vi "tui_DataLog Log Table.vi"() -> ()   [LabVIEW 2012]
doc: "Interactively retrieves and tabulates the content of multiple tag logs. The retrieved data can be filtered, graphed, and exported. This GUI is designed for quick and dirty analysis. When performing complex or recurring retrieval operations, it is advisable to use a query script instead.\n\nThis GUI has two phases. During the first phase you must specify what data is to be retrieved from the logging database. During the second phase you can perform actions on the retrieved data.\n\nSpecifying what data to retrieve involves assigning a set of tags to the table columns and specifying a time interval and optional interpolation time step. After retrieval and tabulation, it is possible to exclude or include rows of data so as to filter the dataset to a subset of interest. A suitable series of include and exclude actions can yield the equivalent of a boolean selection expression. For example, excluding all rows where tag \"foo\" is not equal to 2 and then including all rows where tag \"bar\" is larger than zero is equivalent to retaining all rows that satisfy the boolean expression \"foo==2 or bar>0\".\n\nThe optionally filtered data can be graphed or exported. Only when the dataset is cleared does it again become possible to specify a new set of tags, that is, the GUI will revert back from the second to the first phase.\n\nThe server-side memory usage is kept in check through configurable limits and by performing the retrieval on a per-tag basis. Still, some moderation is advisable since the client-side memory usage is not bounded. When retrieving lots of data for multiple tags, the table will likely take a long time to display and the client might even run out of memory."
uses:
  served/DataLog Database Infos_srv.ctl
  served/re_DataLog Query_srv.ctl
  served/DataLog Databases_srv.ctl
  typedefs/t_DataLog Log Table States.ctl
  library/typedefs/t_Library Session Methods.ctl
  typedefs/t_Datalog Table Columns Methods.ctl
  typedefs/t_DataLog Query Served Methods.ctl
  typedefs/t_DataLog Value Types.ctl
  library/glb_Library Configuration Globals.vi
panel:
  out "export path":path
  in  "string":string
  in  "match":T1(ring)
  in  "number":dbl
  in  "comparison":T2(ring)
  out "excluded":i32
  out "included":i32
  in  "xy graph":bool
  in  "time graph":bool
  in  "include":bool
  in  "exclude":bool
  in  "enable/disable":bool
  in  "time step":dbl=60.0 min=0.01 max=1000000000000.0 step=1.0 format="%<%H:%M:%S%2u>t"
  in  "mode":bool
  in  "reorder":bool
  in  "remove all":bool
  in  "insert":bool
  in  "subset":bool
  in  "add":bool
  in  "multi":bool
  in  "remove":bool
  in  "sort":bool
  in  "export":bool
  in  "clear":bool
  out "query":T3
  in  "database":i32(ring) items=["testdb"]
  out "log table":string[][](table)
  out "database infos":T4
  in  "earliest":bool
  in  "begin time":timestamp format="%<%H:%M:%S%2u\n%Y/%m/%d>T"
  in  "latest":bool
  in  "end time":timestamp format="%<%H:%M:%S%2u\n%Y/%m/%d>T"
  in  "retrieve":bool
  in  "exit":bool
  out "databases":T5
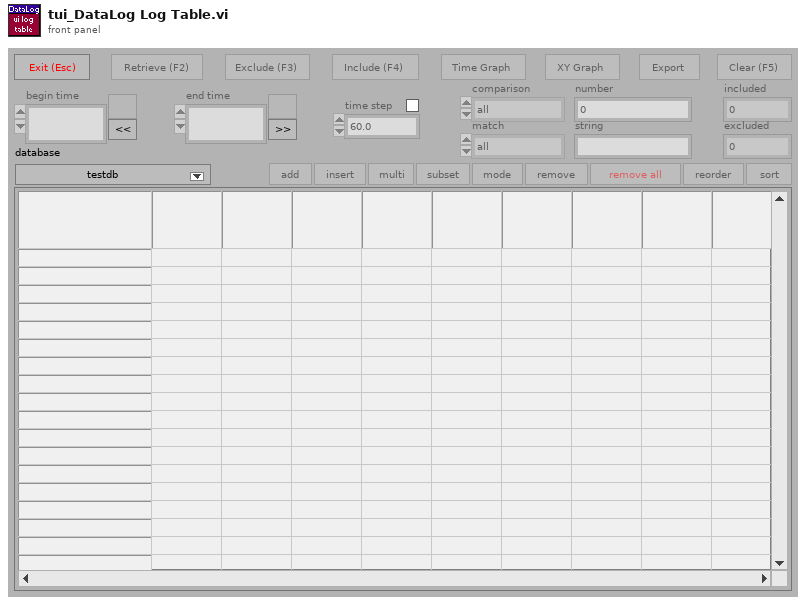
[diagram p1: front panel]
types:
  T1 = enum16{"all", "==", "~=", "contains", "contains c.i.", "lacks", "lacks c.i.", "starts with", "starts with c.i.", "UNDEFINED", "DEFINED"}
  T2 = enum16{"all", "==", "~=", ">", ">=", "<=", "<", "==NaN", "~=NaN"}
  T3 = typedef "re_DataLog Query_srv.ctl" = refnum<vi>
  T4 = typedef "DataLog Database Infos_srv.ctl" = refnum<vi>
  T5 = typedef "DataLog Databases_srv.ctl" = refnum<vi>
  T6 = typedef "t_DataLog Log Table States.ctl" = enum16{"empty queue", "retrieve", "ret clear", "ret presize", "ret range", "ret merge", "ret at", "ret step", "ret times", "ret interpolate", "ret tabulate", "ret free", "num. exclude", "num. include", "str. exclude", "str. include", "time graph", "graph xy", "xy query", "xy check", "xy open", "xy set", "xy correlate", "xy run", "export", "show string", "count rows", "time headers", "tabulate", "abort query", "clear query", "clear all", "set database", "deselect", "ablement", "resize", "initialize", "init refs", "init databases", "init persist", "cleanup", "stop"}
  T7 = typedef "t_Library Session Methods.ctl" = enum16{"run", "get arg", "set arg", "delist", "cleanup?", "start session", "stop session", "list empty?"}
  T8 = typedef "t_Datalog Table Columns Methods.ctl" = enum16{"clear", "#columns", "#number", "add", "insert", "remove", "change mode", "reorder", "sort", "index", "get by name", "interpolatable?", "ats?", "update"}
  T9 = typedef "t_DataLog Query Served Methods.ctl" = enum16{"set range", "step times", "get times", "interpolate", "interpolate str", "read range", "read str range", "merge&read range", "merge&read str range", "merge range", "clear"}
  T10 = cluster{"graph VI":refnum<vi>, "x tag":string, "y tag":string}
  T11 = cluster{"times":dbl[], "values":dbl[], "strings":string[]}
  T12 = typedef "t_DataLog Value Types.ctl" = enum16{"number", "string"}
  T13 = typedef "t_DataLog Tag Config.ctl" = cluster{"name":string, "unit":string, "temporal":T14, "value":T12, "index":i32, "capacity":i32, "is meta?":bool, "mincapacity":i32, "deadband":dbl, "limit delay":dbl, "format":T15, "precision":u8, "undefine":bool, "update":bool, "update period":u16, "expression":string, "description":string, "logging algorithm":T16, "logging parameters":dbl[]}
  T14 = typedef "t_DataLog Temporal Types.ctl" = enum16{"set&hold", "sample", "event"}
  T15 = typedef "t_DataLog Numerical Format.ctl" = enum8{"fractional", "exponential", "engineering"}
  T16 = typedef "t_DataLog Logging Algorithms.ctl" = enum16{"nothing", "changes", "everything", "every Nth", "time threshold", "value threshold + prior", "t or v threshold", "t or v threshold + prior"}
  T17 = enum32{"existing file", "new file", "new or existing file", "existing dir", "new dir", "new or existing dir", "existing file (use LLBs)", "new file (use LLBs)", "new or existing file (use LLBs)", "new or existing file or directory (use LLBs)"}
  T18 = typedef "LVRowAndColumnTypeDef.ctl" = cluster{"Row":i32, "Column":i32}
  T19 = typedef "eventvkey.ctl" = enum16{"ASCII", "Enter", "Return", "Shift", "Ctrl", "Alt", "Cmd", "Opt", "Caps", "NumLock", "Clear", "Break", "Up", "Down", "Left", "Right", "Insert", "Delete", "Home", "End", "PageUp", "PageDown", "Escape", "Help", "Pause", "ScrollLock", "F1", "F2", "F3", "F4", "F5", "F6", "F7", "F8", "F9", "F10", "F11", "F12", "F13", "F14", "F15", "F16", "F17", "F18", "F19", "F20", "F21", "F22", "F23", "F24", "Play", "VolumeUp", "VolumeDown", "Mute", "Two Byte Char"}
  T20 = cluster{"times":dbl[], "values":dbl[], "strings":string[]}[]
  T21 = typedef "t_DataLog Table Retrieval Modes.ctl" = enum16{"at", "interpolate", "at+interpolate"}
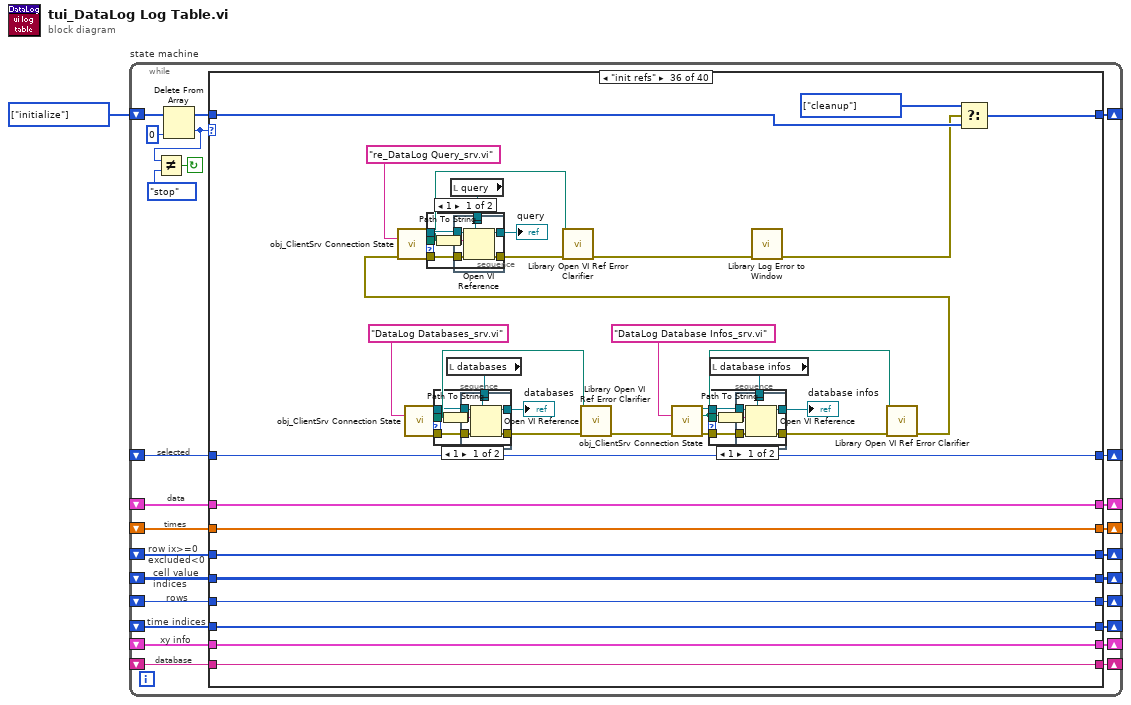
[diagram p0: block diagram]
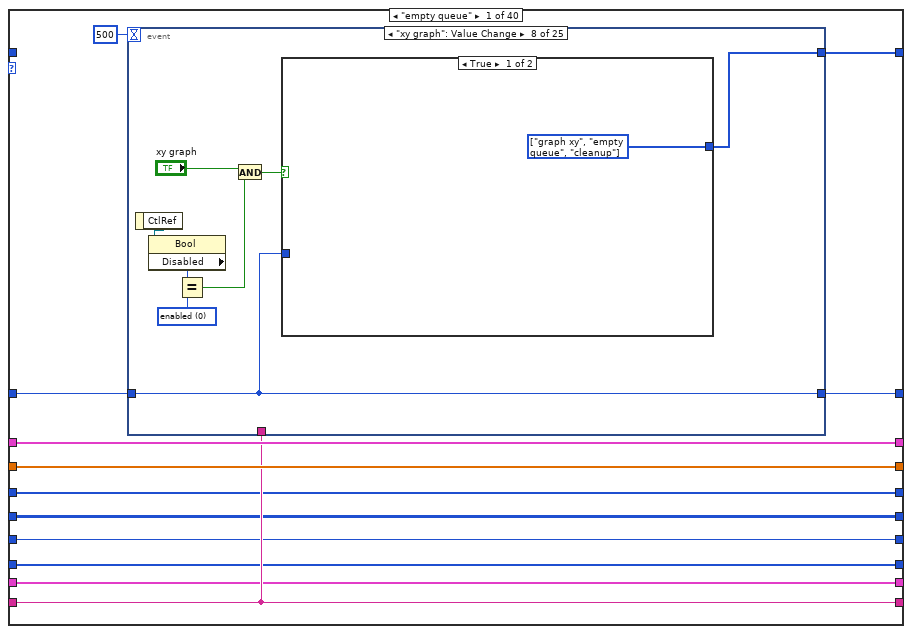
[diagram p2: hidden frame]
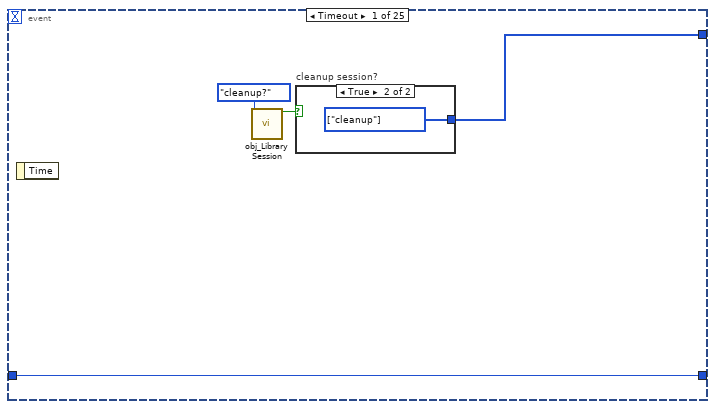
[diagram p3: hidden frame]
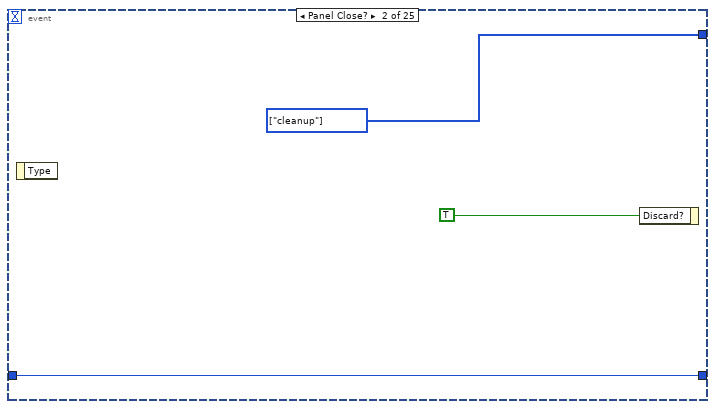
[diagram p5: hidden frame]
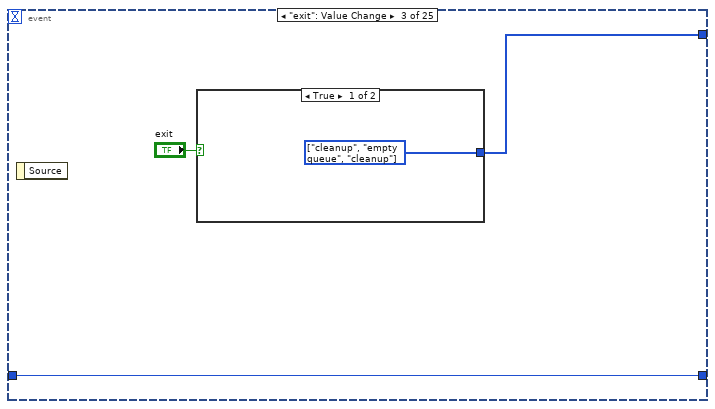
[diagram p6: hidden frame]
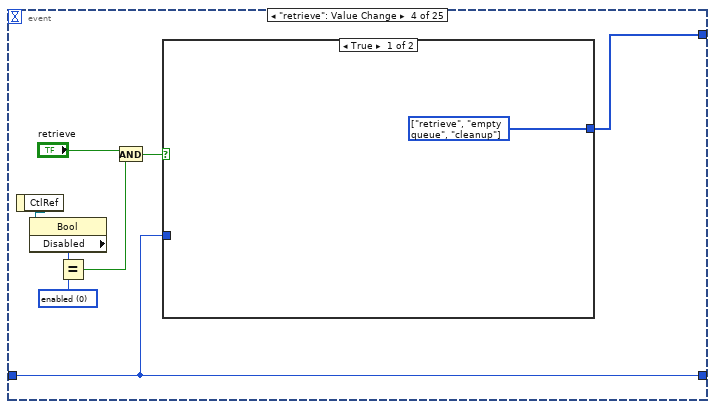
[diagram p8: hidden frame]
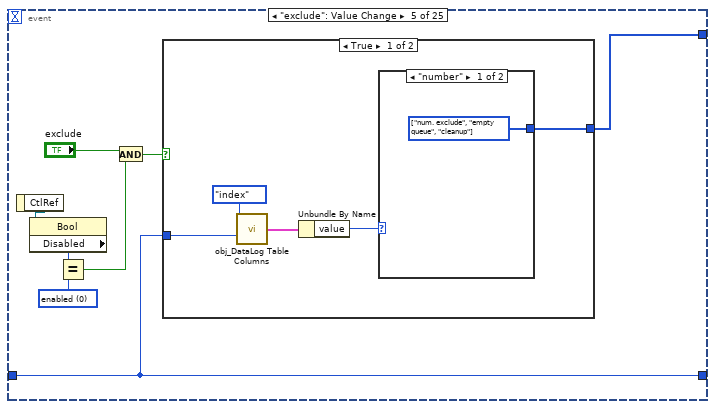
[diagram p10: hidden frame]
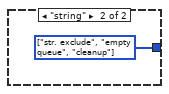
[diagram p11: hidden frame]
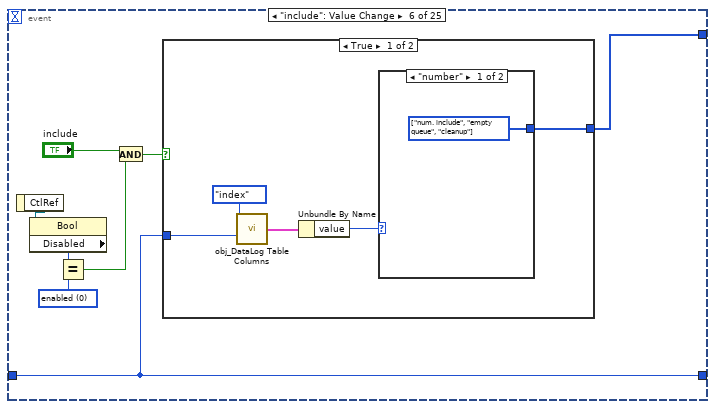
[diagram p13: hidden frame]
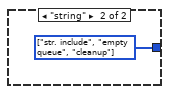
[diagram p14: hidden frame]
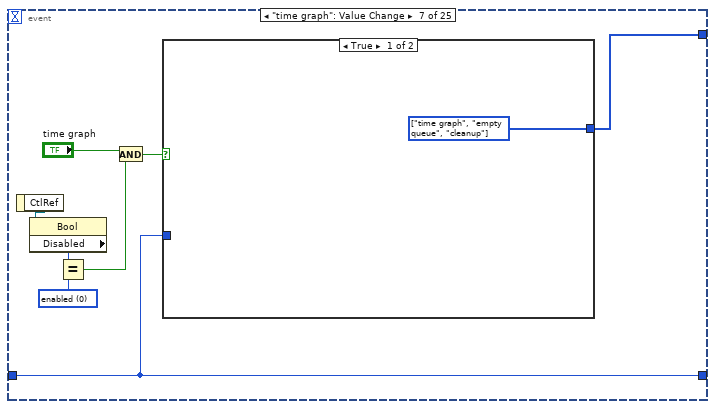
[diagram p16: hidden frame]
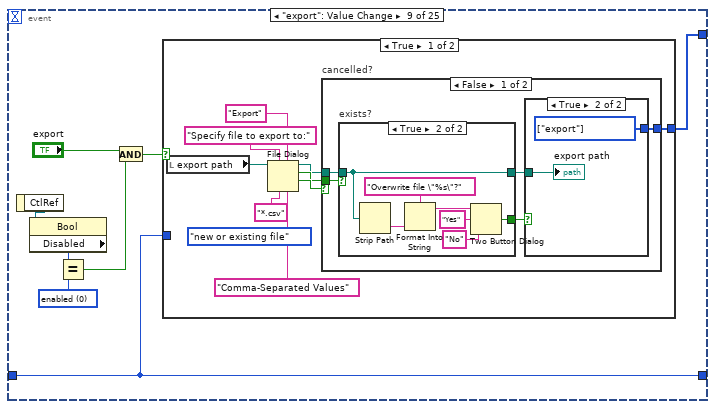
[diagram p19: hidden frame]
diagram:
  w1 = T6[] [enum."initialize"] items=["empty queue", "retrieve", "ret clear", "ret presize", "ret range", "ret merge", "ret at", "ret step", "ret times", "ret interpolate", "ret tabulate", "ret free", "num. exclude", "num. include", "str. exclude", "str. include", "time graph", "graph xy", "xy query", "xy check", "xy open", "xy set", "xy correlate", "xy run", "export", "show string", "count rows", "time headers", "tabulate", "abort query", "clear query", "clear all", "set database", "deselect", "ablement", "resize", "initialize", "init refs", "init databases", "init persist", "cleanup", "stop"] ("Array Constant")
  n1 = while "state machine" {
    shift-left: w1 -> [w23]
    shift-right: [w26] -> _
    shift-right: [w19] -> _
    shift-left: _ -> [w20]
    shift-right: [w17] -> _
    shift-left: _ -> [w18]
    shift-right: [w15] -> _
    shift-left: _ -> [w16]
    shift-right: [w12] -> _
    shift-left: _ -> [w13]
    shift-right: [w10] -> _
    shift-left: _ -> [w11]
    shift-right: [w9] -> _
    shift-left: _ -> [w8]
    shift-right: [w6] -> _
    shift-left: _ -> [w7]
    shift-right: [w5] -> _
    shift-left: _ -> [w4]
    shift-right: [w2] -> _
    shift-left: _ -> [w3]
    stop <- w25 continue-if-true
    # "xy info"
    # "time indices"
    # "cell value\nindices"
    # "rows"
    # "row ix>=0\nexcluded<0"
    # "selected"
    # "times"
    # "data"
    # "database"
    n2 = Delete From Array(array=w23, index=0) -> (deleted portion=w14:T6, array with subset deleted=w22:T6[])  [unwired: 1 in]
    n3 = Not Equal?(x=w14, y=t_DataLog_Log_Table_States."stop" ("states")) -> (x != y?=w25:bool)
    n4 = case "Case" shown="\"init refs\"" w14 {
      selector: w14 -> [_ _ _ _ _ _ _ _ _ _ _ _ w810 w982 _ _ _ _ _ _ _ _ _ _ _ _ _ _ _ _ _ _ _ _ _ _ _ _ _ _]
      tunnel: [w38 w371 w414 w428 w448 w479 w535 w638 w667 w689 w785 w797 w809 w981 w1217 w1295 w1331 w1388 w1450 w1483 w1505 w1754 w1776 w2011 w2077 w2127 w2167 w2408 w2428 w2453 w2483 w2502 w2579 w2618 w2680 w2741 w2825 w2836 w2854 w2864] -> w26
      tunnel: w22 -> [_ _ w418 w438 w446 w477 w533 w636 w666 w687 w789 w797 w820 w992 w1217 _ w1332 w1389 w1451 w1484 w1504 w1754 w1776 w2011 w2077 w2127 w2167 w2410 w2435 w2473 w2489 w2505 w2579 w2618 _ w2739 w2823 w2837 _ w2864]
      tunnel: w20 -> [w32 w374 w417 w437 w468 w482 w538 w641 w676 w692 w788 w803 w819 w991 w1199 w1298 w1341 w1390 w1460 w1485 w1524 w1756 w1778 w2010 w2081 w2131 w2166 w2411 w2437 w2464 _ w2504 w2578 w2617 w2679 w2738 w2826 w2839 _ w2863]
      tunnel: [w32 w374 w417 w437 w468 w482 w538 w641 w676 w692 w788 w803 w819 w991 w1199 w1298 w1341 w1390 w1460 w1485 w1524 w1756 w1778 w2010 w2081 w2131 w2166 w2411 w2437 w2464 w2484 w2504 w2578 w2617 w2679 w2738 w2826 w2839 "" w2863] -> w19
      tunnel: w18 -> [w36 w373 w415 w434 w467 w474 w541 w640 w675 w695 w783 w800 w817 w989 w1208 w1297 w1340 w1378 w1459 w1489 w1517 w1755 w1774 w2004 w2078 w2130 w2164 w2406 w2436 _ w2481 w2507 w2536 w2616 w2678 w2731 w2812 w2835 w2847 w2862]
      tunnel: [w36 w373 w415 w430 w467 w474 w539 w640 w675 w693 w783 w800 w818 w990 w1206 w1297 w1340 w1377 w1459 w1489 w1516 w1755 w1773 w2003 w2078 w2130 w2165 w2406 w2434 w2461 w2481 w2507 w2536 w2616 w2678 w2731 w2812 w2835 w2847 w2862] -> w17
      tunnel: w16 -> [w35 w372 w416 w436 w466 w485 w543 w639 _ w697 w787 w802 w816 w988 w1204 w1299 w1342 w1391 w1461 w1490 w1511 w1757 w1769 w2000 w2080 w2122 w2161 w2405 w2431 w2458 w2480 w2506 w2567 w2615 w2677 w2730 w2811 w2834 w2846 w2861]
      tunnel: [w35 w372 w416 w436 w466 w485 w543 w639 w658 w697 w787 w802 w815 w987 w1204 w1299 w1342 w1391 w1461 w1490 w1511 w1757 w1768 w2000 w2080 w2122 w2160 w2405 w2430 w2457 w2480 w2506 w2567 w2615 w2677 w2730 w2811 w2834 w2846 w2861] -> w15
      tunnel: w13 -> [w34 w370 w405 w429 w444 w475 w531 w634 w664 w685 w786 w801 w811 w983 w1218 w1304 w1347 w1394 w1466 w1495 w1527 w1762 w1777 w2009 w2079 w2128 w2163 w2409 w2429 _ w2479 w2500 w2542 w2614 w2676 w2729 w2810 w2833 w2845 w2860]
      tunnel: [w33 w370 w405 w429 w444 w475 w531 w634 w664 w685 w786 w801 w811 w983 w1218 w1304 w1347 w1394 w1466 w1495 w1527 w1762 w1777 w2009 w2079 w2128 w2162 w2409 w2429 -1 ("dimension size") w2479 -1 w2542 w2614 w2676 w2729 w2810 w2833 w2845 w2860] -> w12
      tunnel: w11 -> [w31 w369 w404 w426 w443 w473 w530 w630 _ w684 w782 w799 w812 w984 w1216 w1303 w1346 w1393 w1465 w1494 w1526 w1761 w1770 w2008 w2076 w2123 w2156 w2400 w2426 w2451 w2478 w2498 w2553 w2613 w2675 w2728 w2809 w2831 w2844 w2859]
      tunnel: [w31 w369 w404 w426 w443 w473 w530 w630 w653 w684 w782 w799 w813 w985 w1216 w1303 w1346 w1393 w1465 w1494 w1526 w1761 w1770 w2008 w2074 w2123 w2157 w2400 w2425 w2450 w2478 w2498 w2553 w2613 w2675 w2728 w2809 w2831 w2844 w2859] -> w10
      tunnel: [w30 w368 w403 w425 w442 w472 w529 w629 w654 w683 w781 w798 w814 w986 w1207 w1301 w1344 w1374 w1463 w1492 w1513 w1759 w1775 w2007 w2070 w2117 w2158 w2399 0 0 ("dimension size") w2477 w2497 w2552 w2612 w2674 w2727 w2808 w2830 w2843 w2858] -> w9
      tunnel: w8 -> [w30 w368 w403 w425 w442 w472 w529 w629 _ w683 w781 w798 w814 w986 w1207 w1301 w1344 w1374 w1463 w1492 w1513 w1759 w1775 w2007 _ w2117 w2159 w2399 _ _ w2477 w2497 w2552 w2612 w2674 w2727 w2808 w2830 w2843 w2858]
      tunnel: w7 -> [w29 w367 w402 w424 w441 w471 w528 w628 w655 w682 w780 w792 w806 w978 w1205 w1300 w1343 w1376 w1462 w1491 w1515 w1758 w1772 w2002 w2065 w2120 _ w2398 w2419 w2445 w2476 w2496 w2527 w2611 w2673 w2726 w2807 w2829 w2842 w2857]
      tunnel: [w29 w367 w402 w424 w441 w471 w528 w628 w655 w682 w780 w792 w806 w978 w1205 w1300 w1343 w1375 w1462 w1491 w1514 w1758 w1771 w2001 w2065 w2120 w2155 w2398 w2418 w2444 w2476 w2496 w2527 w2611 w2673 w2726 w2807 w2829 w2842 w2857] -> w6
      tunnel: [w28 w366 w401 w423 w440 w470 w527 w627 w652 w681 w779 w791 w805 w977 w1209 w1302 w1345 w1392 w1464 w1493 w1525 w1760 w1766 w1999 w2064 w2116 w2154 w2397 w2414 w2440 w2475 w2495 w2526 w2610 w2672 w2725 w2806 w2828 w2841 w2856] -> w5
      tunnel: w4 -> [w28 w366 w401 w423 w440 w470 w527 w627 w652 w681 w779 w791 w805 w977 w1209 w1302 w1345 w1392 w1464 w1493 w1525 w1760 w1767 w1999 w2064 _ w2154 w2397 w2415 w2441 w2475 w2495 w2526 w2610 w2672 w2725 w2806 w2828 w2841 w2856]
      tunnel: w3 -> [w27 w365 w400 w422 w439 w469 w526 w626 w651 w680 w778 w790 w804 w976 w1198 w1296 _ w1387 w1455 w1487 w1509 w1749 w1765 w1998 w2063 w2115 w2153 w2396 w2412 w2438 w2474 w2494 w2525 w2609 w2671 w2724 w2805 w2827 w2840 w2855]
      tunnel: [w27 w365 w400 w422 w439 w469 w526 w626 w651 w680 w778 w790 w804 w976 w1198 w1296 w1330 w1387 w1454 w1487 w1509 w1749 w1765 w1998 w2063 w2115 w2153 w2396 w2412 w2438 w2474 w2494 w2525 w2609 w2671 w2724 w2805 w2827 w2840 w2855] -> w2
      frame "empty queue" {
        n5 = event shown="[7] \"xy graph\": Value Change" {
          selector: _ -> [_ _ _ _ _ _ _ _ _ _ _ _ _ _ _ _ _ _ _ _ _ _ _ _ _]
          dyn-events: _ -> [_ _ _ _ _ _ _ _ _ _ _ _ _ _ _ _ _ _ _ _ _ _ _ _ _]
          timeout: 500 -> [_ _ _ _ _ _ _ _ _ _ _ _ _ _ _ _ _ _ _ _ _ _ _ _ _]
          tunnel: [w42 w46 w49 w58 w67 w75 w97 w106 w115 w148 w158 w176 w195 w205 w225 w244 w255 w264 w274 w278 w280 w281 _ _ w363] -> w38
          tunnel: w34 -> [w39 w44 w47 w52 w61 w77 w91 w100 w109 w142 w157 w175 w194 w206 w218 w237 w249 w258 w268 w277 w279 w285 w348 w359 w364]
          tunnel: [w39 w44 w47 w52 w61 w77 w91 w100 w109 w142 w157 w175 w194 w206 w218 w237 w249 w258 w268 w277 w279 w284 w348 w359 w364] -> w33
          tunnel: w32 -> [_ _ _ _ _ _ _ _ _ _ w150 w168 w188 w208 w217 _ _ _ _ _ _ _ _ _ _]
          event Timeout {
            n6 = event-data() -> ()  [unwired: 1 in, 1 out]
            n7 = call "obj_Library Session.vi"("method"=t_Library_Session_Methods."cleanup?") -> ("cleanup/empty?"=w40:bool)  [unwired: 11 in, 3 out]
            n8 = case "cleanup session?" shown="True" w40 {
              tunnel: [_ w43] -> w42
              frame False {
              }
              frame True {
                w43 = T6[] [enum."cleanup"] items=["empty queue", "retrieve", "ret clear", "ret presize", "ret range", "ret merge", "ret at", "ret step", "ret times", "ret interpolate", "ret tabulate", "ret free", "num. exclude", "num. include", "str. exclude", "str. include", "time graph", "graph xy", "xy query", "xy check", "xy open", "xy set", "xy correlate", "xy run", "export", "show string", "count rows", "time headers", "tabulate", "abort query", "clear query", "clear all", "set database", "deselect", "ablement", "resize", "initialize", "init refs", "init databases", "init persist", "cleanup", "stop"] ("Array Constant")
              }
            }
          }
          event Panel Close? {
            w46 = T6[] [enum."cleanup"] items=["empty queue", "retrieve", "ret clear", "ret presize", "ret range", "ret merge", "ret at", "ret step", "ret times", "ret interpolate", "ret tabulate", "ret free", "num. exclude", "num. include", "str. exclude", "str. include", "time graph", "graph xy", "xy query", "xy check", "xy open", "xy set", "xy correlate", "xy run", "export", "show string", "count rows", "time headers", "tabulate", "abort query", "clear query", "clear all", "set database", "deselect", "ablement", "resize", "initialize", "init refs", "init databases", "init persist", "cleanup", "stop"] ("Array Constant")
            n9 = event-data() -> ()  [unwired: 1 in, 1 out]
            n10 = event-data("Discard?"=TRUE) -> ()  [unwired: 1 in, 1 out]
          }
          event "exit": Value Change {
            n11 = event-data() -> ()  [unwired: 1 in, 1 out]
            n12 = case shown="True" "exit" {
              tunnel: [w50 _] -> w49
              frame True {
                w50 = T6[] [enum."cleanup", enum."empty queue", enum."cleanup"] items=["empty queue", "retrieve", "ret clear", "ret presize", "ret range", "ret merge", "ret at", "ret step", "ret times", "ret interpolate", "ret tabulate", "ret free", "num. exclude", "num. include", "str. exclude", "str. include", "time graph", "graph xy", "xy query", "xy check", "xy open", "xy set", "xy correlate", "xy run", "export", "show string", "count rows", "time headers", "tabulate", "abort query", "clear query", "clear all", "set database", "deselect", "ablement", "resize", "initialize", "init refs", "init databases", "init persist", "cleanup", "stop"] ("Array Constant")
              }
              frame False {
              }
            }
          }
          event "retrieve": Value Change {
            w55 = u8 0 items=["enabled", "disabled", "grayed"] ("disabled state")
            n13 = event-data() -> ("CtlRef"=w57:refnum<vi>)  [unwired: 1 in]
            n14 = property class="Bool"(reference=w57) -> ("Disabled"=w56:u8)  [unwired: 1 in, 2 out]
            n15 = Equal?(x=w56, y=w55) -> (x = y?=w53:bool)
            n16 = And(x="retrieve", y=w53) -> (x .and. y?=w54:bool)
            n17 = case shown="True" w54 {
              tunnel: [w59 _] -> w58
              tunnel: w52 -> [_ _]
              frame True {
                w59 = T6[] [enum."retrieve", enum."empty queue", enum."cleanup"] items=["empty queue", "retrieve", "ret clear", "ret presize", "ret range", "ret merge", "ret at", "ret step", "ret times", "ret interpolate", "ret tabulate", "ret free", "num. exclude", "num. include", "str. exclude", "str. include", "time graph", "graph xy", "xy query", "xy check", "xy open", "xy set", "xy correlate", "xy run", "export", "show string", "count rows", "time headers", "tabulate", "abort query", "clear query", "clear all", "set database", "deselect", "ablement", "resize", "initialize", "init refs", "init databases", "init persist", "cleanup", "stop"] ("Array Constant")
              }
              frame False {
              }
            }
          }
          event "exclude": Value Change {
            w64 = u8 0 items=["enabled", "disabled", "grayed"] ("disabled state")
            n18 = event-data() -> ("CtlRef"=w66:refnum<vi>)  [unwired: 1 in]
            n19 = property class="Bool"(reference=w66) -> ("Disabled"=w65:u8)  [unwired: 1 in, 2 out]
            n20 = Equal?(x=w65, y=w64) -> (x = y?=w62:bool)
            n21 = And(x="exclude", y=w62) -> (x .and. y?=w63:bool)
            n22 = case shown="True" w63 {
              tunnel: [w72 _] -> w67
              tunnel: w61 -> [w70 _]
              frame True {
                n23 = call "obj_DataLog Table Columns.vi"("method"=t_Datalog_Table_Columns_Methods."index", "index"=w70) -> ("tag config"=w69:T13)  [unwired: 8 in, 5 out]
                n24 = Unbundle By Name(w69) -> ("value"=w68:T12)
                n25 = case shown="\"number\"" w68 {
                  tunnel: [w73 w74] -> w72
                  frame "number" {
                    w73 = T6[] [enum."num. exclude", enum."empty queue", enum."cleanup"] items=["empty queue", "retrieve", "ret clear", "ret presize", "ret range", "ret merge", "ret at", "ret step", "ret times", "ret interpolate", "ret tabulate", "ret free", "num. exclude", "num. include", "str. exclude", "str. include", "time graph", "graph xy", "xy query", "xy check", "xy open", "xy set", "xy correlate", "xy run", "export", "show string", "count rows", "time headers", "tabulate", "abort query", "clear query", "clear all", "set database", "deselect", "ablement", "resize", "initialize", "init refs", "init databases", "init persist", "cleanup", "stop"] ("Array Constant")
                  }
                  frame "string" {
                    w74 = T6[] [enum."str. exclude", enum."empty queue", enum."cleanup"] items=["empty queue", "retrieve", "ret clear", "ret presize", "ret range", "ret merge", "ret at", "ret step", "ret times", "ret interpolate", "ret tabulate", "ret free", "num. exclude", "num. include", "str. exclude", "str. include", "time graph", "graph xy", "xy query", "xy check", "xy open", "xy set", "xy correlate", "xy run", "export", "show string", "count rows", "time headers", "tabulate", "abort query", "clear query", "clear all", "set database", "deselect", "ablement", "resize", "initialize", "init refs", "init databases", "init persist", "cleanup", "stop"] ("Array Constant")
                  }
                }
              }
              frame False {
              }
            }
          }
          event "include": Value Change {
            w80 = u8 0 items=["enabled", "disabled", "grayed"] ("disabled state")
            n26 = event-data() -> ("CtlRef"=w82:refnum<vi>)  [unwired: 1 in]
            n27 = property class="Bool"(reference=w82) -> ("Disabled"=w81:u8)  [unwired: 1 in, 2 out]
            n28 = Equal?(x=w81, y=w80) -> (x = y?=w79:bool)
            n29 = And(x="include", y=w79) -> (x .and. y?=w76:bool)
            n30 = case shown="True" w76 {
              tunnel: [w87 _] -> w75
              tunnel: w77 -> [w85 _]
              frame True {
                n31 = call "obj_DataLog Table Columns.vi"("method"=t_Datalog_Table_Columns_Methods."index", "index"=w85) -> ("tag config"=w84:T13)  [unwired: 8 in, 5 out]
                n32 = Unbundle By Name(w84) -> ("value"=w83:T12)
                n33 = case shown="\"number\"" w83 {
                  tunnel: [w88 w89] -> w87
                  frame "number" {
                    w88 = T6[] [enum."num. include", enum."empty queue", enum."cleanup"] items=["empty queue", "retrieve", "ret clear", "ret presize", "ret range", "ret merge", "ret at", "ret step", "ret times", "ret interpolate", "ret tabulate", "ret free", "num. exclude", "num. include", "str. exclude", "str. include", "time graph", "graph xy", "xy query", "xy check", "xy open", "xy set", "xy correlate", "xy run", "export", "show string", "count rows", "time headers", "tabulate", "abort query", "clear query", "clear all", "set database", "deselect", "ablement", "resize", "initialize", "init refs", "init databases", "init persist", "cleanup", "stop"] ("Array Constant")
                  }
                  frame "string" {
                    w89 = T6[] [enum."str. include", enum."empty queue", enum."cleanup"] items=["empty queue", "retrieve", "ret clear", "ret presize", "ret range", "ret merge", "ret at", "ret step", "ret times", "ret interpolate", "ret tabulate", "ret free", "num. exclude", "num. include", "str. exclude", "str. include", "time graph", "graph xy", "xy query", "xy check", "xy open", "xy set", "xy correlate", "xy run", "export", "show string", "count rows", "time headers", "tabulate", "abort query", "clear query", "clear all", "set database", "deselect", "ablement", "resize", "initialize", "init refs", "init databases", "init persist", "cleanup", "stop"] ("Array Constant")
                  }
                }
              }
              frame False {
              }
            }
          }
          event "time graph": Value Change {
            w94 = u8 0 items=["enabled", "disabled", "grayed"] ("disabled state")
            n34 = event-data() -> ("CtlRef"=w96:refnum<vi>)  [unwired: 1 in]
            n35 = property class="Bool"(reference=w96) -> ("Disabled"=w95:u8)  [unwired: 1 in, 2 out]
            n36 = Equal?(x=w95, y=w94) -> (x = y?=w92:bool)
            n37 = And(x="time graph", y=w92) -> (x .and. y?=w93:bool)
            n38 = case shown="True" w93 {
              tunnel: [w98 _] -> w97
              tunnel: w91 -> [_ _]
              frame True {
                w98 = T6[] [enum."time graph", enum."empty queue", enum."cleanup"] items=["empty queue", "retrieve", "ret clear", "ret presize", "ret range", "ret merge", "ret at", "ret step", "ret times", "ret interpolate", "ret tabulate", "ret free", "num. exclude", "num. include", "str. exclude", "str. include", "time graph", "graph xy", "xy query", "xy check", "xy open", "xy set", "xy correlate", "xy run", "export", "show string", "count rows", "time headers", "tabulate", "abort query", "clear query", "clear all", "set database", "deselect", "ablement", "resize", "initialize", "init refs", "init databases", "init persist", "cleanup", "stop"] ("Array Constant")
              }
              frame False {
              }
            }
          }
          event "xy graph": Value Change {
            w103 = u8 0 items=["enabled", "disabled", "grayed"] ("disabled state")
            n39 = event-data() -> ("CtlRef"=w105:refnum<vi>)  [unwired: 1 in]
            n40 = property class="Bool"(reference=w105) -> ("Disabled"=w104:u8)  [unwired: 1 in, 2 out]
            n41 = Equal?(x=w104, y=w103) -> (x = y?=w101:bool)
            n42 = And(x="xy graph", y=w101) -> (x .and. y?=w102:bool)
            n43 = case shown="True" w102 {
              tunnel: [w107 _] -> w106
              tunnel: w100 -> [_ _]
              frame True {
                w107 = T6[] [enum."graph xy", enum."empty queue", enum."cleanup"] items=["empty queue", "retrieve", "ret clear", "ret presize", "ret range", "ret merge", "ret at", "ret step", "ret times", "ret interpolate", "ret tabulate", "ret free", "num. exclude", "num. include", "str. exclude", "str. include", "time graph", "graph xy", "xy query", "xy check", "xy open", "xy set", "xy correlate", "xy run", "export", "show string", "count rows", "time headers", "tabulate", "abort query", "clear query", "clear all", "set database", "deselect", "ablement", "resize", "initialize", "init refs", "init databases", "init persist", "cleanup", "stop"] ("Array Constant")
              }
              frame False {
              }
            }
          }
          event "export": Value Change {
            w112 = u8 0 items=["enabled", "disabled", "grayed"] ("disabled state")
            n44 = event-data() -> ("CtlRef"=w114:refnum<vi>)  [unwired: 1 in]
            n45 = property class="Bool"(reference=w114) -> ("Disabled"=w113:u8)  [unwired: 1 in, 2 out]
            n46 = Equal?(x=w113, y=w112) -> (x = y?=w110:bool)
            n47 = And(x="export", y=w110) -> (x .and. y?=w111:bool)
            n48 = case shown="True" w111 {
              tunnel: [w118 _] -> w115
              tunnel: w109 -> [_ _]
              frame True {
                (unwired) T17."new or existing file" ("select mode (2)")
                n49 = local read "export path"() -> (w119:path)
                n50 = File Dialog(4:"Comma-Separated Values" ("pattern label"), 5:"Export" ("button label"), 6:"*.csv" ("pattern"), 7:"Specify file to export to:" ("prompt"), 11:w119) -> (1:w122:bool, 2:w121:bool, 3:w120:path)  [unwired: 2 in, 1 out]
                n51 = case "cancelled?" shown="False" w122 {
                  tunnel: w121 -> [w129 _]
                  tunnel: w120 -> [w128 _]
                  tunnel: [w125 _] -> w118
                  frame False {
                    n52 = case "exists?" shown="True" w129 {
                      tunnel: w128 -> [w133 w135]
                      tunnel: [TRUE ("T button?") w136] -> w126
                      tunnel: [w133 w135] -> w127
                      frame False {
                      }
                      frame True {
                        n53 = Strip Path(path=w135) -> (name=w134:string)  [unwired: 1 out]
                        n54 = Format Into String(format string="Overwrite file \"%s\"?", w134) -> (resulting string=w137:string)  [unwired: 2 in, 1 out]
                        n55 = Two Button Dialog(message=w137, 1:"No" ("F button name (\"Cancel\")"), 2:"Yes" ("T button name (\"OK\")")) -> (T button?=w136:bool)
                      }
                    }
                    n56 = case shown="True" w126 {
                      tunnel: w127 -> [_ w131]
                      tunnel: [_ w130] -> w125
                      frame False {
                      }
                      frame True {
                        w130 = T6[] [enum."export"] items=["empty queue", "retrieve", "ret clear", "ret presize", "ret range", "ret merge", "ret at", "ret step", "ret times", "ret interpolate", "ret tabulate", "ret free", "num. exclude", "num. include", "str. exclude", "str. include", "time graph", "graph xy", "xy query", "xy check", "xy open", "xy set", "xy correlate", "xy run", "export", "show string", "count rows", "time headers", "tabulate", "abort query", "clear query", "clear all", "set database", "deselect", "ablement", "resize", "initialize", "init refs", "init databases", "init persist", "cleanup", "stop"] ("Array Constant")
                        "export path" <- w131
                      }
                    }
                  }
                  frame True {
                  }
                }
              }
              frame False {
              }
            }
          }
          event "clear": Value Change {
            w145 = u8 0 items=["enabled", "disabled", "grayed"] ("disabled state")
            n57 = event-data() -> ("CtlRef"=w147:refnum<vi>)  [unwired: 1 in]
            n58 = property class="Bool"(reference=w147) -> ("Disabled"=w146:u8)  [unwired: 1 in, 2 out]
            n59 = Equal?(x=w146, y=w145) -> (x = y?=w143:bool)
            n60 = And(x="clear", y=w143) -> (x .and. y?=w144:bool)
            n61 = case shown="True" w144 {
              tunnel: [w149 _] -> w148
              tunnel: w142 -> [_ _]
              frame True {
                w149 = T6[] [enum."clear query", enum."empty queue", enum."cleanup"] items=["empty queue", "retrieve", "ret clear", "ret presize", "ret range", "ret merge", "ret at", "ret step", "ret times", "ret interpolate", "ret tabulate", "ret free", "num. exclude", "num. include", "str. exclude", "str. include", "time graph", "graph xy", "xy query", "xy check", "xy open", "xy set", "xy correlate", "xy run", "export", "show string", "count rows", "time headers", "tabulate", "abort query", "clear query", "clear all", "set database", "deselect", "ablement", "resize", "initialize", "init refs", "init databases", "init persist", "cleanup", "stop"] ("Array Constant")
              }
              frame False {
              }
            }
          }
          event "add": Value Change {
            w154 = u8 0 items=["enabled", "disabled", "grayed"] ("disabled state")
            n62 = event-data() -> ("CtlRef"=w156:refnum<vi>)  [unwired: 1 in]
            n63 = property class="Bool"(reference=w156) -> ("Disabled"=w155:u8)  [unwired: 1 in, 2 out]
            n64 = Equal?(x=w155, y=w154) -> (x = y?=w151:bool)
            n65 = And(x="add", y=w151) -> (x .and. y?=w153:bool)
            n66 = case shown="True" w153 {
              tunnel: [w163 _] -> w158
              tunnel: w150 -> [w159 _]
              frame True {
                n67 = call "ui_DataLog Query Tag.vi"("prompt"="Select tag to add to table:", "database"=w159) -> ("OK?"=w161:bool, "tag"=w160:string)  [unwired: 12 in]
                n68 = case shown="True" w161 {
                  tunnel: [_ w167] -> w163
                  tunnel: w160 -> [_ w164]
                  frame False {
                  }
                  frame True {
                    w167 = T6[] [enum."ablement", enum."empty queue", enum."cleanup"] items=["empty queue", "retrieve", "ret clear", "ret presize", "ret range", "ret merge", "ret at", "ret step", "ret times", "ret interpolate", "ret tabulate", "ret free", "num. exclude", "num. include", "str. exclude", "str. include", "time graph", "graph xy", "xy query", "xy check", "xy open", "xy set", "xy correlate", "xy run", "export", "show string", "count rows", "time headers", "tabulate", "abort query", "clear query", "clear all", "set database", "deselect", "ablement", "resize", "initialize", "init refs", "init databases", "init persist", "cleanup", "stop"] ("Array Constant")
                    n69 = call "obj_DataLog Table Columns.vi"("method"=t_Datalog_Table_Columns_Methods."add", "tag"=w164) -> ("error out"=w165:errorcluster)  [unwired: 8 in, 5 out]
                    n70 = call "Library Log Error to Window.vi"("error in (no error)"=w165) -> ()  [unwired: 13 in, 2 out]
                  }
                }
              }
              frame False {
              }
            }
          }
          event "multi": Value Change {
            w172 = u8 0 items=["enabled", "disabled", "grayed"] ("disabled state")
            n71 = event-data() -> ("CtlRef"=w174:refnum<vi>)  [unwired: 1 in]
            n72 = property class="Bool"(reference=w174) -> ("Disabled"=w173:u8)  [unwired: 1 in, 2 out]
            n73 = Equal?(x=w173, y=w172) -> (x = y?=w170:bool)
            n74 = And(x="multi", y=w170) -> (x .and. y?=w171:bool)
            n75 = case shown="True" w171 {
              tunnel: [w181 _] -> w176
              tunnel: w168 -> [w177 _]
              frame True {
                n76 = call "ui_DataLog Query Tags.vi"("prompt"="Select tags to add to table:", "database"=w177) -> ("OK?"=w179:bool, "tag"=w178:string[])  [unwired: 12 in]
                n77 = case shown="True" w179 {
                  tunnel: [_ w183] -> w181
                  tunnel: w178 -> [_ w182]
                  frame False {
                  }
                  frame True {
                    w183 = T6[] [enum."ablement", enum."empty queue", enum."cleanup"] items=["empty queue", "retrieve", "ret clear", "ret presize", "ret range", "ret merge", "ret at", "ret step", "ret times", "ret interpolate", "ret tabulate", "ret free", "num. exclude", "num. include", "str. exclude", "str. include", "time graph", "graph xy", "xy query", "xy check", "xy open", "xy set", "xy correlate", "xy run", "export", "show string", "count rows", "time headers", "tabulate", "abort query", "clear query", "clear all", "set database", "deselect", "ablement", "resize", "initialize", "init refs", "init databases", "init persist", "cleanup", "stop"] ("Array Constant")
                    n78 = for {
                      tunnel: w182 -> [w184] mode=indexing
                      n79 = call "obj_DataLog Table Columns.vi"("method"=t_Datalog_Table_Columns_Methods."add", "tag"=w184) -> ("error out"=w185:errorcluster)  [unwired: 8 in, 5 out]
                      n80 = call "Library Log Error to Window.vi"("error in (no error)"=w185) -> ()  [unwired: 13 in, 2 out]
                    }
                  }
                }
              }
              frame False {
              }
            }
          }
          event "subset": Value Change {
            w191 = u8 0 items=["enabled", "disabled", "grayed"] ("disabled state")
            n81 = event-data() -> ("CtlRef"=w193:refnum<vi>)  [unwired: 1 in]
            n82 = property class="Bool"(reference=w193) -> ("Disabled"=w192:u8)  [unwired: 1 in, 2 out]
            n83 = Equal?(x=w192, y=w191) -> (x = y?=w189:bool)
            n84 = And(x="subset", y=w189) -> (x .and. y?=w190:bool)
            n85 = case shown="True" w190 {
              tunnel: [w199 _] -> w195
              tunnel: w188 -> [w198 _]
              frame True {
                n86 = call "ui_DataLog Get or Query Subset.vi"("database"=w198) -> ("OK?"=w196:bool, "tags in subset"=w197:string[])  [unwired: 11 in, 2 out]
                n87 = case shown="True" w196 {
                  tunnel: [_ w201] -> w199
                  tunnel: w197 -> [_ w200]
                  frame False {
                  }
                  frame True {
                    w201 = T6[] [enum."ablement", enum."empty queue", enum."cleanup"] items=["empty queue", "retrieve", "ret clear", "ret presize", "ret range", "ret merge", "ret at", "ret step", "ret times", "ret interpolate", "ret tabulate", "ret free", "num. exclude", "num. include", "str. exclude", "str. include", "time graph", "graph xy", "xy query", "xy check", "xy open", "xy set", "xy correlate", "xy run", "export", "show string", "count rows", "time headers", "tabulate", "abort query", "clear query", "clear all", "set database", "deselect", "ablement", "resize", "initialize", "init refs", "init databases", "init persist", "cleanup", "stop"] ("Array Constant")
                    n88 = for {
                      tunnel: w200 -> [w202] mode=indexing
                      n89 = call "obj_DataLog Table Columns.vi"("method"=t_Datalog_Table_Columns_Methods."add", "tag"=w202) -> ("error out"=w203:errorcluster)  [unwired: 8 in, 5 out]
                      n90 = call "Library Log Error to Window.vi"("error in (no error)"=w203) -> ()  [unwired: 13 in, 2 out]
                    }
                  }
                }
              }
              frame False {
              }
            }
          }
          event "mode": Value Change {
            w211 = u8 0 items=["enabled", "disabled", "grayed"] ("disabled state")
            n91 = event-data() -> ("CtlRef"=w213:refnum<vi>)  [unwired: 1 in]
            n92 = property class="Bool"(reference=w213) -> ("Disabled"=w212:u8)  [unwired: 1 in, 2 out]
            n93 = Equal?(x=w212, y=w211) -> (x = y?=w209:bool)
            n94 = And(x="mode", y=w209) -> (x .and. y?=w210:bool)
            n95 = case shown="True" w210 {
              tunnel: w208 -> [_ _]
              tunnel: w206 -> [w215 _]
              tunnel: [w214 _] -> w205
              frame True {
                w214 = T6[] [enum."ablement"] items=["empty queue", "retrieve", "ret clear", "ret presize", "ret range", "ret merge", "ret at", "ret step", "ret times", "ret interpolate", "ret tabulate", "ret free", "num. exclude", "num. include", "str. exclude", "str. include", "time graph", "graph xy", "xy query", "xy check", "xy open", "xy set", "xy correlate", "xy run", "export", "show string", "count rows", "time headers", "tabulate", "abort query", "clear query", "clear all", "set database", "deselect", "ablement", "resize", "initialize", "init refs", "init databases", "init persist", "cleanup", "stop"] ("Array Constant")
                n96 = call "obj_DataLog Table Columns.vi"("method"=t_Datalog_Table_Columns_Methods."change mode", "index"=w215) -> ()  [unwired: 8 in, 6 out]
              }
              frame False {
              }
            }
          }
          event "insert": Value Change {
            w222 = u8 0 items=["enabled", "disabled", "grayed"] ("disabled state")
            n97 = event-data() -> ("CtlRef"=w224:refnum<vi>)  [unwired: 1 in]
            n98 = property class="Bool"(reference=w224) -> ("Disabled"=w223:u8)  [unwired: 1 in, 2 out]
            n99 = Equal?(x=w223, y=w222) -> (x = y?=w220:bool)
            n100 = And(x="insert", y=w220) -> (x .and. y?=w221:bool)
            n101 = case shown="True" w221 {
              tunnel: [w231 _] -> w225
              tunnel: w218 -> [w227 _]
              tunnel: w217 -> [w226 _]
              frame True {
                n102 = call "ui_DataLog Query Tag.vi"("prompt"="Select tag to insert:", "database"=w226) -> ("OK?"=w229:bool, "tag"=w228:string)  [unwired: 12 in]
                n103 = case shown="True" w229 {
                  tunnel: [_ w236] -> w231
                  tunnel: w228 -> [_ w233]
                  tunnel: w227 -> [_ w232]
                  frame False {
                  }
                  frame True {
                    w236 = T6[] [enum."ablement", enum."empty queue", enum."cleanup"] items=["empty queue", "retrieve", "ret clear", "ret presize", "ret range", "ret merge", "ret at", "ret step", "ret times", "ret interpolate", "ret tabulate", "ret free", "num. exclude", "num. include", "str. exclude", "str. include", "time graph", "graph xy", "xy query", "xy check", "xy open", "xy set", "xy correlate", "xy run", "export", "show string", "count rows", "time headers", "tabulate", "abort query", "clear query", "clear all", "set database", "deselect", "ablement", "resize", "initialize", "init refs", "init databases", "init persist", "cleanup", "stop"] ("Array Constant")
                    n104 = call "obj_DataLog Table Columns.vi"("method"=t_Datalog_Table_Columns_Methods."insert", "tag"=w233, "index"=w232) -> ("error out"=w234:errorcluster)  [unwired: 7 in, 5 out]
                    n105 = call "Library Log Error to Window.vi"("error in (no error)"=w234) -> ()  [unwired: 13 in, 2 out]
                  }
                }
              }
              frame False {
              }
            }
          }
          event "remove": Value Change {
            w241 = u8 0 items=["enabled", "disabled", "grayed"] ("disabled state")
            n106 = event-data() -> ("CtlRef"=w243:refnum<vi>)  [unwired: 1 in]
            n107 = property class="Bool"(reference=w243) -> ("Disabled"=w242:u8)  [unwired: 1 in, 2 out]
            n108 = Equal?(x=w242, y=w241) -> (x = y?=w239:bool)
            n109 = And(x="remove", y=w239) -> (x .and. y?=w240:bool)
            n110 = case shown="True" w240 {
              tunnel: [w247 _] -> w244
              tunnel: w237 -> [w245 _]
              frame True {
                w247 = T6[] [enum."deselect", enum."empty queue", enum."cleanup"] items=["empty queue", "retrieve", "ret clear", "ret presize", "ret range", "ret merge", "ret at", "ret step", "ret times", "ret interpolate", "ret tabulate", "ret free", "num. exclude", "num. include", "str. exclude", "str. include", "time graph", "graph xy", "xy query", "xy check", "xy open", "xy set", "xy correlate", "xy run", "export", "show string", "count rows", "time headers", "tabulate", "abort query", "clear query", "clear all", "set database", "deselect", "ablement", "resize", "initialize", "init refs", "init databases", "init persist", "cleanup", "stop"] ("Array Constant")
                n111 = call "obj_DataLog Table Columns.vi"("method"=t_Datalog_Table_Columns_Methods."remove", "index"=w245) -> ()  [unwired: 8 in, 6 out]
              }
              frame False {
              }
            }
          }
          event "remove all": Value Change {
            w252 = u8 0 items=["enabled", "disabled", "grayed"] ("disabled state")
            n112 = event-data() -> ("CtlRef"=w254:refnum<vi>)  [unwired: 1 in]
            n113 = property class="Bool"(reference=w254) -> ("Disabled"=w253:u8)  [unwired: 1 in, 2 out]
            n114 = Equal?(x=w253, y=w252) -> (x = y?=w250:bool)
            n115 = And(x="remove all", y=w250) -> (x .and. y?=w251:bool)
            n116 = case shown="True" w251 {
              tunnel: [w256 _] -> w255
              frame True {
                w256 = T6[] [enum."clear all", enum."empty queue", enum."cleanup"] items=["empty queue", "retrieve", "ret clear", "ret presize", "ret range", "ret merge", "ret at", "ret step", "ret times", "ret interpolate", "ret tabulate", "ret free", "num. exclude", "num. include", "str. exclude", "str. include", "time graph", "graph xy", "xy query", "xy check", "xy open", "xy set", "xy correlate", "xy run", "export", "show string", "count rows", "time headers", "tabulate", "abort query", "clear query", "clear all", "set database", "deselect", "ablement", "resize", "initialize", "init refs", "init databases", "init persist", "cleanup", "stop"] ("Array Constant")
              }
              frame False {
              }
            }
          }
          event "reorder": Value Change {
            w261 = u8 0 items=["enabled", "disabled", "grayed"] ("disabled state")
            n117 = event-data() -> ("CtlRef"=w263:refnum<vi>)  [unwired: 1 in]
            n118 = property class="Bool"(reference=w263) -> ("Disabled"=w262:u8)  [unwired: 1 in, 2 out]
            n119 = Equal?(x=w262, y=w261) -> (x = y?=w259:bool)
            n120 = And(x="reorder", y=w259) -> (x .and. y?=w260:bool)
            n121 = case shown="True" w260 {
              tunnel: [w266 _] -> w264
              frame True {
                w266 = T6[] [enum."deselect", enum."empty queue", enum."cleanup"] items=["empty queue", "retrieve", "ret clear", "ret presize", "ret range", "ret merge", "ret at", "ret step", "ret times", "ret interpolate", "ret tabulate", "ret free", "num. exclude", "num. include", "str. exclude", "str. include", "time graph", "graph xy", "xy query", "xy check", "xy open", "xy set", "xy correlate", "xy run", "export", "show string", "count rows", "time headers", "tabulate", "abort query", "clear query", "clear all", "set database", "deselect", "ablement", "resize", "initialize", "init refs", "init databases", "init persist", "cleanup", "stop"] ("Array Constant")
                n122 = call "obj_DataLog Table Columns.vi"("method"=t_Datalog_Table_Columns_Methods."reorder") -> ()  [unwired: 9 in, 6 out]
              }
              frame False {
              }
            }
          }
          event "sort": Value Change {
            w271 = u8 0 items=["enabled", "disabled", "grayed"] ("disabled state")
            n123 = event-data() -> ("CtlRef"=w273:refnum<vi>)  [unwired: 1 in]
            n124 = property class="Bool"(reference=w273) -> ("Disabled"=w272:u8)  [unwired: 1 in, 2 out]
            n125 = Equal?(x=w272, y=w271) -> (x = y?=w269:bool)
            n126 = And(x="sort", y=w269) -> (x .and. y?=w270:bool)
            n127 = case shown="True" w270 {
              tunnel: [w276 _] -> w274
              frame True {
                w276 = T6[] [enum."deselect", enum."empty queue", enum."cleanup"] items=["empty queue", "retrieve", "ret clear", "ret presize", "ret range", "ret merge", "ret at", "ret step", "ret times", "ret interpolate", "ret tabulate", "ret free", "num. exclude", "num. include", "str. exclude", "str. include", "time graph", "graph xy", "xy query", "xy check", "xy open", "xy set", "xy correlate", "xy run", "export", "show string", "count rows", "time headers", "tabulate", "abort query", "clear query", "clear all", "set database", "deselect", "ablement", "resize", "initialize", "init refs", "init databases", "init persist", "cleanup", "stop"] ("Array Constant")
                n128 = call "obj_DataLog Table Columns.vi"("method"=t_Datalog_Table_Columns_Methods."sort") -> ()  [unwired: 9 in, 6 out]
              }
              frame False {
              }
            }
          }
          event "database": Value Change {
            w278 = T6[] [enum."set database"] items=["empty queue", "retrieve", "ret clear", "ret presize", "ret range", "ret merge", "ret at", "ret step", "ret times", "ret interpolate", "ret tabulate", "ret free", "num. exclude", "num. include", "str. exclude", "str. include", "time graph", "graph xy", "xy query", "xy check", "xy open", "xy set", "xy correlate", "xy run", "export", "show string", "count rows", "time headers", "tabulate", "abort query", "clear query", "clear all", "set database", "deselect", "ablement", "resize", "initialize", "init refs", "init databases", "init persist", "cleanup", "stop"] ("Array Constant")
            n129 = event-data() -> ()  [unwired: 1 in, 1 out]
          }
          event "end time", "latest", "begin time", "earliest", "enable/disable", "comparison", "match": Value Change {
            w280 = T6[] [enum."ablement"] items=["empty queue", "retrieve", "ret clear", "ret presize", "ret range", "ret merge", "ret at", "ret step", "ret times", "ret interpolate", "ret tabulate", "ret free", "num. exclude", "num. include", "str. exclude", "str. include", "time graph", "graph xy", "xy query", "xy check", "xy open", "xy set", "xy correlate", "xy run", "export", "show string", "count rows", "time headers", "tabulate", "abort query", "clear query", "clear all", "set database", "deselect", "ablement", "resize", "initialize", "init refs", "init databases", "init persist", "cleanup", "stop"] ("Array Constant")
            n130 = event-data() -> ()  [unwired: 1 in, 1 out]
          }
          event "log table": Mouse Down {
            n131 = event-data() -> ("Button"=w283:u16, "CtlRef"=w282:refnum<vi>)  [unwired: 1 in]
            n132 = case shown="1" w283 {
              tunnel: w282 -> [_ w301]
              tunnel: w285 -> [w286 w300]
              tunnel: [w286 w299] -> w284
              tunnel: [_ w290] -> w281
              frame Default {
              }
              frame 1 {
                # "use the edit position to determine\nand toggle the clicked header"
                # "1==left mouse button"
                n133 = property class="Tbl (strict)"(reference=w301) -> (reference out=w302:refnum<vi>, "Old Edit Position"=w297:T18, "Column Header Strings[]"=w295:string[])  [unwired: 1 in, 1 out]
                n134 = Unbundle By Name(w297) -> ("Row"=w288:i32, "Column"=w294:i32)
                n135 = Array Size(array=w295) -> (size(s)=w293:i32)
                n136 = Bundle By Name(cluster=w297, "Row"=0) -> (w296:T18)
                n137 = Less?(x=w294, y=w293) -> (x < y?=w291:bool)
                n138 = Equal?(x=-1, y=w288) -> (x = y?=w289:bool)
                n139 = And(x=w289, y=w291) -> (x .and. y?=w292:bool)
                n140 = case shown="True" w292 {
                  tunnel: w302 -> [_ w314]
                  tunnel: w297 -> [_ w308]
                  tunnel: w300 -> [w304 w307]
                  tunnel: [w304 w312] -> w299
                  tunnel: w294 -> [_ w313]
                  tunnel: w296 -> [_ w309]
                  tunnel: [w303 w305] -> w290
                  frame False {
                    w303 = T6[] [enum."show string"] items=["empty queue", "retrieve", "ret clear", "ret presize", "ret range", "ret merge", "ret at", "ret step", "ret times", "ret interpolate", "ret tabulate", "ret free", "num. exclude", "num. include", "str. exclude", "str. include", "time graph", "graph xy", "xy query", "xy check", "xy open", "xy set", "xy correlate", "xy run", "export", "show string", "count rows", "time headers", "tabulate", "abort query", "clear query", "clear all", "set database", "deselect", "ablement", "resize", "initialize", "init refs", "init databases", "init persist", "cleanup", "stop"] ("Array Constant")
                  }
                  frame True {
                    w305 = T6[] [enum."ablement"] items=["empty queue", "retrieve", "ret clear", "ret presize", "ret range", "ret merge", "ret at", "ret step", "ret times", "ret interpolate", "ret tabulate", "ret free", "num. exclude", "num. include", "str. exclude", "str. include", "time graph", "graph xy", "xy query", "xy check", "xy open", "xy set", "xy correlate", "xy run", "export", "show string", "count rows", "time headers", "tabulate", "abort query", "clear query", "clear all", "set database", "deselect", "ablement", "resize", "initialize", "init refs", "init databases", "init persist", "cleanup", "stop"] ("Array Constant")
                    n141 = Bundle By Name(cluster=w308, "Column"=w307) -> (w306:T18)
                    n142 = Equal?(x=w313, y=w307) -> (x = y?=w311:bool)
                    n143 = Greater Or Equal To 0?(x=w307) -> (x >= 0?=w310:bool)
                    n144 = case shown="True" w311 {
                      tunnel: w314 -> [w319 w331]
                      tunnel: w308 -> [w318 w330]
                      tunnel: w309 -> [w317 w329]
                      tunnel: w313 -> [_ w328]
                      tunnel: [-1 w328] -> w312
                      tunnel: w310 -> [w316 w327]
                      tunnel: w306 -> [_ w326]
                      frame True {
                        n145 = case shown="True" w316 {
                          tunnel: w319 -> [_ w325]
                          tunnel: w318 -> [_ w324]
                          tunnel: w317 -> [_ w323]
                          frame False {
                          }
                          frame True {
                            n146 = property class="Tbl (strict)"(reference=w325, "Active Cell:Active Cell"=w324, "Old Edit Position"=w323, "Active Cell:Cell Background Color"=u32 15790320, "Active Cell:Cell FG Color"=u32 0, "Key Focus"=FALSE) -> ()  [unwired: 1 in, 2 out]
                          }
                        }
                      }
                      frame False {
                        n147 = case shown="True" w327 {
                          tunnel: w331 -> [w340 w346]
                          tunnel: w330 -> [w339 w345]
                          tunnel: w329 -> [w338 w344]
                          tunnel: w326 -> [w337 _]
                          frame True {
                            n148 = property class="Tbl (strict)"(reference=w340, "Active Cell:Active Cell"=w339, "Old Edit Position"=w338, "Active Cell:Cell Background Color"=u32 128, "Active Cell:Cell FG Color"=u32 16777215, "Active Cell:Active Cell"=w337, "Active Cell:Cell Background Color"=u32 15790320, "Active Cell:Cell FG Color"=u32 0, "Key Focus"=FALSE) -> ()  [unwired: 1 in, 2 out]
                          }
                          frame False {
                            n149 = property class="Tbl (strict)"(reference=w346, "Active Cell:Active Cell"=w345, "Old Edit Position"=w344, "Active Cell:Cell Background Color"=u32 128, "Active Cell:Cell FG Color"=u32 16777215, "Key Focus"=FALSE) -> ()  [unwired: 1 in, 2 out]
                          }
                        }
                      }
                    }
                  }
                }
              }
            }
          }
          event Key Down? {
            n150 = event-data() -> ("VKey"=w347:T19, "FocusObj"=w349:refnum<vi>)  [unwired: 1 in]
            n151 = call <vilib>:"compatReturnToEnter.vi"("VKey"=w347) -> ("VKey"=w351:T19)
            n152 = case shown="\"Up\", \"Down\"" w351 {
              tunnel: [TRUE _ _] -> w350
              tunnel: w349 -> [_ w356 _]
              frame "F1" {
                n153 = call "Library Show Help.vi"() -> ()  [unwired: 1 in]
              }
              frame "Up", "Down" {
                n154 = Type Cast(type=0, x=w356) -> (*(type *) &x=w355:i32)
                n155 = Equal To 0?(x=w355) -> (x = 0?=w353:bool)
                n156 = case shown="True" w353 {
                  frame False {
                  }
                  frame True {
                    n157 = property on="log table" class="Tbl (strict)"("Key Focus"=TRUE) -> ()  [unwired: 2 in, 2 out]
                  }
                }
              }
              frame Default {
              }
            }
            n158 = event-data("Discard?"=w350) -> ()  [unwired: 1 in, 1 out]
          }
          event event type 5.0.x8000000b {
            n159 = event-data() -> ("VKey"=w358:T19)  [unwired: 1 in]
            n160 = call <vilib>:"compatReturnToEnter.vi"("VKey"=w358) -> ("VKey"=w361:T19)
            n161 = case shown="\"F1\"" w361 {
              tunnel: [TRUE _] -> w360
              frame "F1" {
              }
              frame Default {
              }
            }
            n162 = event-data("Discard?"=w360) -> ()  [unwired: 1 in, 1 out]
          }
          event Panel Resize {
            w363 = T6[] [enum."resize"] items=["empty queue", "retrieve", "ret clear", "ret presize", "ret range", "ret merge", "ret at", "ret step", "ret times", "ret interpolate", "ret tabulate", "ret free", "num. exclude", "num. include", "str. exclude", "str. include", "time graph", "graph xy", "xy query", "xy check", "xy open", "xy set", "xy correlate", "xy run", "export", "show string", "count rows", "time headers", "tabulate", "abort query", "clear query", "clear all", "set database", "deselect", "ablement", "resize", "initialize", "init refs", "init databases", "init persist", "cleanup", "stop"] ("Array Constant")
            n163 = event-data() -> ()  [unwired: 1 in, 1 out]
          }
        }
      }
      frame "retrieve" {
        n164 = while "rebuild retrieve list on first run or after load or recompile" {
          shift-left: _ -> [w377]
          shift-right: [w376] -> w371
          stop <- FALSE continue-if-true
          n165 = Array Size(array=w377) -> (size(s)=w378:i32)
          n166 = case shown="0" w378 {
            tunnel: [w379 w399] -> w376
            tunnel: w377 -> [w380 w399]
            frame 0 {
              n167 = while {
                shift-left: w380 -> [w389]
                shift-right: [w387] -> w379
                shift-left: _ -> [w391]
                shift-right: [w386] -> _
                i -> [w394]
                stop <- w382 continue-if-true
                n168 = To Unsigned Word Integer(number=w394) -> (unsigned 16bit integer=w392:u16)
                n169 = Type Cast(type=t_DataLog_Log_Table_States."initialize" ("states"), x=w392) -> (*(type *) &x=w388:T6)
                n170 = Format Into String(format string="%s" ("Format String"), w388) -> (resulting string=w386:string)  [unwired: 2 in, 1 out]
                n171 = Not Equal?(x=w386, y=w391) -> (x != y?=w382:bool)
                n172 = Match Pattern(string=w386, regular expression="^ret ") -> (offset past match=w384:i32)  [unwired: 1 in, 3 out]
                n173 = Greater Or Equal To 0?(x=w384) -> (x >= 0?=w383:bool)
                n174 = And(x=w383, y=w382) -> (x .and. y?=w381:bool)
                n175 = case shown="True" w381 {
                  tunnel: w389 -> [w395 w398]
                  tunnel: w388 -> [_ w397]
                  tunnel: [w395 w396] -> w387
                  frame False {
                  }
                  frame True {
                    n176 = Build Array (concatenate)(w398, w397) -> (w396:T6[])
                  }
                }
              }
            }
            frame Default {
            }
          }
        }
      }
      frame "ret clear" {
        n177 = call "obj_ClientSrv Client Access State.vi"() -> ("certificate"=w410:string, "error out"=w412:errorcluster)  [unwired: 14 in]
        n178 = local read "query"() -> (w408:T3)
        n179 = call-by-ref "?"(reference=w408, error in=w412, "method"=t_DataLog_Query_Served_Methods."clear", "certificate"=w410) -> (error out=w413:errorcluster, 15:"error out"=w411:errorcluster)  [unwired: 8 in, 6 out]
        n180 = call "Library Remote Call Error Merger.vi"("call by reference node error"=w413, "called VI error (no error)"=w411) -> ("error out"=w407:errorcluster)  [unwired: 13 in]
        n181 = call "Library Log Error to Window.vi"("error in (no error)"=w407) -> ("dup error"=w406:errorcluster)  [unwired: 13 in, 1 out]
        n182 = case shown="No Error" w406 {
          tunnel: w418 -> [w421 _]
          tunnel: [w420 _] -> w414
          frame No Error {
            n183 = Build Array (concatenate)(t_DataLog_Log_Table_States."clear query" ("states"), w421) -> (w420:T6[])
          }
          frame Error {
          }
        }
      }
      frame "ret presize" {
        n184 = Index Array(array=w434, index=-1) -> (element=w432:T11)
        n185 = call "obj_DataLog Table Columns.vi"("method"=t_Datalog_Table_Columns_Methods."#columns") -> ("#columns"=w431:i32)  [unwired: 9 in, 5 out]
        n186 = Initialize Array(w432, w431) -> (w430:T20)
        n187 = Build Array (concatenate)(t_DataLog_Log_Table_States."deselect" ("states"), w438) -> (w428:T6[])
      }
      frame "ret range" {
        w447 = T6[] [enum."abort query"] items=["empty queue", "retrieve", "ret clear", "ret presize", "ret range", "ret merge", "ret at", "ret step", "ret times", "ret interpolate", "ret tabulate", "ret free", "num. exclude", "num. include", "str. exclude", "str. include", "time graph", "graph xy", "xy query", "xy check", "xy open", "xy set", "xy correlate", "xy run", "export", "show string", "count rows", "time headers", "tabulate", "abort query", "clear query", "clear all", "set database", "deselect", "ablement", "resize", "initialize", "init refs", "init databases", "init persist", "cleanup", "stop"] ("Array Constant")
        n188 = local read "earliest"() -> (w458:bool)
        n189 = local read "latest"() -> (w459:bool)
        n190 = To Double Precision Float(number="begin time") -> (double precision float=w463:dbl)
        n191 = To Double Precision Float(number="end time") -> (double precision float=w461:dbl)
        n192 = Select(t=-inf ("double precision float"), s=w458, f=w463) -> (s? t:f=w453:dbl)
        n193 = Select(t=inf ("double precision float"), s=w459, f=w461) -> (s? t:f=w450:dbl)
        n194 = call "obj_ClientSrv Client Access State.vi"() -> ("certificate"=w454:string, "error out"=w456:errorcluster)  [unwired: 14 in]
        n195 = local read "query"() -> (w451:T3)
        n196 = call-by-ref "?"(reference=w451, error in=w456, "method"=t_DataLog_Query_Served_Methods."set range", "begin of range"=w453, "certificate"=w454, "end of range"=w450, "database (current)"=w468) -> (error out=w457:errorcluster, 15:"error out"=w455:errorcluster)  [unwired: 5 in, 6 out]
        n197 = call "Library Remote Call Error Merger.vi"("call by reference node error"=w457, "called VI error (no error)"=w455) -> ("error out"=w449:errorcluster)  [unwired: 13 in]
        n198 = call "Library Log Error to Window.vi"("error in (no error)"=w449) -> ("dup error"=w445:errorcluster)  [unwired: 13 in, 1 out]
        n199 = Select(t=w447, s=w445, f=w446) -> (s? t:f=w448:T6[])
      }
      frame "ret merge" {
        w480 = T6[] [enum."abort query"] items=["empty queue", "retrieve", "ret clear", "ret presize", "ret range", "ret merge", "ret at", "ret step", "ret times", "ret interpolate", "ret tabulate", "ret free", "num. exclude", "num. include", "str. exclude", "str. include", "time graph", "graph xy", "xy query", "xy check", "xy open", "xy set", "xy correlate", "xy run", "export", "show string", "count rows", "time headers", "tabulate", "abort query", "clear query", "clear all", "set database", "deselect", "ablement", "resize", "initialize", "init refs", "init databases", "init persist", "cleanup", "stop"] ("Array Constant")
        n200 = call "obj_DataLog Table Columns.vi"("method"=t_Datalog_Table_Columns_Methods."#columns") -> ("#columns"=w483:i32)  [unwired: 9 in, 5 out]
        n201 = for {
          N: w483 -> [_]
          tunnel: w482 -> [w489]
          shift-right: [w487] -> w481
          shift-left: errorcluster {"status"=FALSE, "code"=0, "source"=""} -> [w486]
          i -> [w488]
          n202 = case shown="No Error" w486 {
            selector: w486 -> [w491 w525]
            tunnel: w489 -> [w495 _]
            tunnel: w488 -> [w494 _]
            tunnel: [w493 w525] -> w487
            frame No Error {
              n203 = call "obj_DataLog Table Columns.vi"("method"=t_Datalog_Table_Columns_Methods."index", "index"=w494, "error in (no error)"=w491) -> ("tag config"=w496:T13, "mode"=w490:T21, "error out"=w492:errorcluster)  [unwired: 7 in, 3 out]
              n204 = case shown="\"at+interpolate\"" w490 {
                tunnel: w496 -> [_ w503]
                tunnel: w495 -> [_ w502]
                tunnel: w494 -> [_ w501]
                tunnel: [w498 w500] -> w493
                tunnel: w492 -> [w498 w499]
                frame "at", "interpolate" {
                }
                frame "at+interpolate" {
                  n205 = stacked-sequence {
                    tunnel: w503 -> [_ w513 _]
                    tunnel: w502 -> [_ w509 _]
                    tunnel: w501 -> [w506 _ w524]
                    tunnel: [_ w511 _] -> w500
                    tunnel: w499 -> [_ w510 _]
                    frame #0 {
                      n206 = Bundle("element"=-1, w506) -> (w505:cluster{"element":i32, i32})  [unwired: 1 in]
                      n207 = call <vilib>:"Set Busy.vi"() -> ()  [unwired: 10 in, 2 out]
                      n208 = property on="log table" class="Tbl (strict)"("Active Cell:Active Cell"=w505, "Active Cell:Cell Background Color"=u32 8404992, "Active Cell:Cell FG Color"=u32 16777215) -> ()  [unwired: 2 in, 2 out]
                    }
                    frame #1 {
                      n209 = Unbundle By Name(w513) -> ("name"=w512:string)
                      n210 = local read "query"() -> (w514:T3)
                      n211 = call "obj_ClientSrv Client Access State.vi"("error in (no error)"=w510) -> ("certificate"=w516:string, "error out"=w518:errorcluster)  [unwired: 13 in]
                      n212 = call-by-ref "?"(reference=w514, error in=w518, "method"=t_DataLog_Query_Served_Methods."merge range", "certificate"=w516, "tag"=w512, "database (current)"=w509) -> (error out=w519:errorcluster, 15:"error out"=w517:errorcluster)  [unwired: 6 in, 6 out]
                      n213 = call "Library Remote Call Error Merger.vi"("call by reference node error"=w519, "called VI error (no error)"=w517) -> ("error out"=w511:errorcluster)  [unwired: 13 in]
                    }
                    frame #2 {
                      n214 = Bundle("element"=-1, w524) -> (w523:cluster{"element":i32, i32})  [unwired: 1 in]
                      n215 = call <vilib>:"Unset Busy.vi"() -> ()  [unwired: 11 in, 1 out]
                      n216 = property on="log table" class="Tbl (strict)"("Active Cell:Active Cell"=w523, "Active Cell:Cell Background Color"=u32 15790320, "Active Cell:Cell FG Color"=u32 0) -> ()  [unwired: 2 in, 2 out]
                    }
                  }
                }
              }
            }
            frame Error {
            }
          }
        }
        n217 = call "Library Log Error to Window.vi"("error in (no error)"=w481) -> ("dup error"=w478:errorcluster)  [unwired: 13 in, 1 out]
        n218 = Select(t=w480, s=w478, f=w477) -> (s? t:f=w479:T6[])
      }
      frame "ret at" {
        w536 = T6[] [enum."abort query"] items=["empty queue", "retrieve", "ret clear", "ret presize", "ret range", "ret merge", "ret at", "ret step", "ret times", "ret interpolate", "ret tabulate", "ret free", "num. exclude", "num. include", "str. exclude", "str. include", "time graph", "graph xy", "xy query", "xy check", "xy open", "xy set", "xy correlate", "xy run", "export", "show string", "count rows", "time headers", "tabulate", "abort query", "clear query", "clear all", "set database", "deselect", "ablement", "resize", "initialize", "init refs", "init databases", "init persist", "cleanup", "stop"] ("Array Constant")
        n219 = call "obj_DataLog Table Columns.vi"("method"=t_Datalog_Table_Columns_Methods."#columns") -> ("#columns"=w540:i32)  [unwired: 9 in, 5 out]
        n220 = for {
          N: w540 -> [_]
          shift-right: [w547] -> w539
          shift-left: w541 -> [w548]
          tunnel: w538 -> [w549]
          shift-right: [w545] -> w537
          shift-left: errorcluster {"status"=FALSE, "code"=0, "source"=""} -> [w544]
          i -> [w546]
          n221 = case shown="No Error" w544 {
            selector: w544 -> [w551 w624]
            tunnel: w549 -> [w557 _]
            tunnel: w548 -> [w556 w625]
            tunnel: [w555 w625] -> w547
            tunnel: w546 -> [w554 _]
            tunnel: [w553 w624] -> w545
            frame No Error {
              n222 = call "obj_DataLog Table Columns.vi"("method"=t_Datalog_Table_Columns_Methods."index", "index"=w554, "error in (no error)"=w551) -> ("tag config"=w558:T13, "mode"=w550:T21, "error out"=w552:errorcluster)  [unwired: 7 in, 3 out]
              n223 = case shown="\"at\"" w550 {
                tunnel: w558 -> [_ w568]
                tunnel: w557 -> [_ w567]
                tunnel: w556 -> [w560 w566]
                tunnel: [w560 w565] -> w555
                tunnel: w554 -> [_ w564]
                tunnel: [w561 w563] -> w553
                tunnel: w552 -> [w561 w562]
                frame "interpolate", "at+interpolate" {
                }
                frame "at" {
                  n224 = stacked-sequence {
                    tunnel: w568 -> [_ w575 _]
                    tunnel: w567 -> [_ w581 _]
                    tunnel: w566 -> [_ w580 _]
                    tunnel: [_ w579 _] -> w565
                    tunnel: w564 -> [w571 w578 w623]
                    tunnel: [_ w577 _] -> w563
                    tunnel: w562 -> [_ w576 _]
                    frame #0 {
                      n225 = Bundle("element"=-1, w571) -> (w570:cluster{"element":i32, i32})  [unwired: 1 in]
                      n226 = call <vilib>:"Set Busy.vi"() -> ()  [unwired: 10 in, 2 out]
                      n227 = property on="log table" class="Tbl (strict)"("Active Cell:Active Cell"=w570, "Active Cell:Cell Background Color"=u32 32768, "Active Cell:Cell FG Color"=u32 16777215) -> ()  [unwired: 2 in, 2 out]
                    }
                    frame #1 {
                      n228 = Unbundle By Name(w575) -> ("value"=w574:T12)
                      n229 = case shown="\"string\"" w574 {
                        tunnel: w575 -> [w593 w612]
                        tunnel: w581 -> [w591 w610]
                        tunnel: w580 -> [w590 w609]
                        tunnel: [w588 w607] -> w579
                        tunnel: w578 -> [w587 w606]
                        tunnel: [w585 w604] -> w577
                        tunnel: w576 -> [w584 w603]
                        frame "number" {
                          n230 = Unbundle By Name(w593) -> ("name"=w592:string)
                          n231 = local read "query"() -> (w594:T3)
                          n232 = call "obj_ClientSrv Client Access State.vi"("error in (no error)"=w584) -> ("certificate"=w596:string, "error out"=w598:errorcluster)  [unwired: 13 in]
                          n233 = Index Array(array=w590, index=w587) -> (element=w589:T11)
                          n234 = call-by-ref "?"(reference=w594, error in=w598, "method"=t_DataLog_Query_Served_Methods."merge&read range", "certificate"=w596, "tag"=w592, "database (current)"=w591) -> (error out=w599:errorcluster, "values"=w583:dbl[], "times"=w582:dbl[], 15:"error out"=w597:errorcluster)  [unwired: 6 in, 4 out]
                          n235 = Bundle By Name(cluster=w589, "values"=w583, "times"=w582) -> (w586:T11)
                          n236 = call "Library Remote Call Error Merger.vi"("call by reference node error"=w599, "called VI error (no error)"=w597) -> ("error out"=w585:errorcluster)  [unwired: 13 in]
                          n237 = Replace Array Subset(array=w590, new element=w586, index=w587) -> (w588:T20)
                        }
                        frame "string" {
                          n238 = Unbundle By Name(w612) -> ("name"=w611:string)
                          n239 = local read "query"() -> (w613:T3)
                          n240 = call "obj_ClientSrv Client Access State.vi"("error in (no error)"=w603) -> ("certificate"=w615:string, "error out"=w617:errorcluster)  [unwired: 13 in]
                          n241 = Index Array(array=w609, index=w606) -> (element=w608:T11)
                          n242 = call-by-ref "?"(reference=w613, error in=w617, "method"=t_DataLog_Query_Served_Methods."merge&read str range", "certificate"=w615, "tag"=w611, "database (current)"=w610) -> (error out=w618:errorcluster, "values"=w600:dbl[], "times"=w601:dbl[], "strings"=w602:string[], 15:"error out"=w616:errorcluster)  [unwired: 6 in, 3 out]
                          n243 = Bundle By Name(cluster=w608, "values"=w600, "times"=w601, "strings"=w602) -> (w605:T11)
                          n244 = call "Library Remote Call Error Merger.vi"("call by reference node error"=w618, "called VI error (no error)"=w616) -> ("error out"=w604:errorcluster)  [unwired: 13 in]
                          n245 = Replace Array Subset(array=w609, new element=w605, index=w606) -> (w607:T20)
                        }
                      }
                    }
                    frame #2 {
                      n246 = Bundle("element"=-1, w623) -> (w622:cluster{"element":i32, i32})  [unwired: 1 in]
                      n247 = call <vilib>:"Unset Busy.vi"() -> ()  [unwired: 11 in, 1 out]
                      n248 = property on="log table" class="Tbl (strict)"("Active Cell:Active Cell"=w622, "Active Cell:Cell Background Color"=u32 15790320, "Active Cell:Cell FG Color"=u32 0) -> ()  [unwired: 2 in, 2 out]
                    }
                  }
                }
              }
            }
            frame Error {
            }
          }
        }
        n249 = call "Library Log Error to Window.vi"("error in (no error)"=w537) -> ("dup error"=w534:errorcluster)  [unwired: 13 in, 1 out]
        n250 = Select(t=w536, s=w534, f=w533) -> (s? t:f=w535:T6[])
      }
      frame "ret step" {
        w632 = u8 0 items=["enabled", "disabled", "grayed"] ("disabled state")
        w637 = T6[] [enum."abort query"] items=["empty queue", "retrieve", "ret clear", "ret presize", "ret range", "ret merge", "ret at", "ret step", "ret times", "ret interpolate", "ret tabulate", "ret free", "num. exclude", "num. include", "str. exclude", "str. include", "time graph", "graph xy", "xy query", "xy check", "xy open", "xy set", "xy correlate", "xy run", "export", "show string", "count rows", "time headers", "tabulate", "abort query", "clear query", "clear all", "set database", "deselect", "ablement", "resize", "initialize", "init refs", "init databases", "init persist", "cleanup", "stop"] ("Array Constant")
        n251 = property on="time step" class="DigNum (strict)"() -> ("Disabled"=w633:u8)  [unwired: 2 in, 2 out]
        n252 = Equal?(x=w633, y=w632) -> (x = y?=w631:bool)
        n253 = case shown="True" w631 {
          tunnel: [_ w643] -> w635
          frame False {
          }
          frame True {
            n254 = call "obj_ClientSrv Client Access State.vi"() -> ("certificate"=w647:string, "error out"=w649:errorcluster)  [unwired: 14 in]
            n255 = local read "query"() -> (w645:T3)
            n256 = call-by-ref "?"(reference=w645, error in=w649, "method"=t_DataLog_Query_Served_Methods."step times", "time step"="time step", "certificate"=w647) -> (error out=w650:errorcluster, 15:"error out"=w648:errorcluster)  [unwired: 7 in, 6 out]
            n257 = call "Library Remote Call Error Merger.vi"("call by reference node error"=w650, "called VI error (no error)"=w648) -> ("error out"=w644:errorcluster)  [unwired: 13 in]
            n258 = call "Library Log Error to Window.vi"("error in (no error)"=w644) -> ("dup error"=w643:errorcluster)  [unwired: 13 in, 1 out]
          }
        }
        n259 = Select(t=w637, s=w635, f=w636) -> (s? t:f=w638:T6[])
      }
      frame "ret times" {
        w668 = T6[] [enum."abort query"] items=["empty queue", "retrieve", "ret clear", "ret presize", "ret range", "ret merge", "ret at", "ret step", "ret times", "ret interpolate", "ret tabulate", "ret free", "num. exclude", "num. include", "str. exclude", "str. include", "time graph", "graph xy", "xy query", "xy check", "xy open", "xy set", "xy correlate", "xy run", "export", "show string", "count rows", "time headers", "tabulate", "abort query", "clear query", "clear all", "set database", "deselect", "ablement", "resize", "initialize", "init refs", "init databases", "init persist", "cleanup", "stop"] ("Array Constant")
        n260 = call "obj_ClientSrv Client Access State.vi"() -> ("certificate"=w672:string, "error out"=w665:errorcluster)  [unwired: 14 in]
        n261 = local read "query"() -> (w670:T3)
        n262 = call-by-ref "?"(reference=w670, error in=w665, "method"=t_DataLog_Query_Served_Methods."get times", "certificate"=w672) -> (error out=w674:errorcluster, "times"=w658:dbl[], 15:"error out"=w673:errorcluster)  [unwired: 8 in, 5 out]
        n263 = call "Library Remote Call Error Merger.vi"("call by reference node error"=w674, "called VI error (no error)"=w673) -> ("error out"=w669:errorcluster)  [unwired: 13 in]
        n264 = Array Size(array=w658) -> (size(s)=w654:i32)
        n265 = Equal To 0?(x=w654) -> (x = 0?=w657:bool)
        n266 = call "Library Log Error to Window.vi"("error in (no error)"=w669) -> ("error?"=w661:bool)  [unwired: 13 in, 1 out]
        n267 = local write "included"(w654) -> ()
        n268 = for {
          N: w654 -> [_]
          tunnel: [w679] -> w653 mode=indexing
          i -> [w679]
        }
        n269 = case shown="True" w657 {
          tunnel: [_ w678] -> w659
          frame False {
          }
          frame True {
            n270 = One Button Dialog(message="No data could be retrieved.\nNone of the tags with \"at\" or\n\"at+interpolate\" retrieval mode\nhave logged data within the\nspecified time range.") -> (true=w678:bool)  [unwired: 1 in]
          }
        }
        n271 = Build Array (concatenate)(t_DataLog_Log_Table_States."time headers" ("states"), w666) -> (w663:T6[])
        n272 = local write "excluded"(0 ("dimension size")) -> ()
        n273 = Or(x=w661, y=w659) -> (x .or. y?=w660:bool)
        n274 = Select(t=w668, s=w660, f=w663) -> (s? t:f=w667:T6[])
      }
      frame "ret interpolate" {
        w690 = T6[] [enum."abort query"] items=["empty queue", "retrieve", "ret clear", "ret presize", "ret range", "ret merge", "ret at", "ret step", "ret times", "ret interpolate", "ret tabulate", "ret free", "num. exclude", "num. include", "str. exclude", "str. include", "time graph", "graph xy", "xy query", "xy check", "xy open", "xy set", "xy correlate", "xy run", "export", "show string", "count rows", "time headers", "tabulate", "abort query", "clear query", "clear all", "set database", "deselect", "ablement", "resize", "initialize", "init refs", "init databases", "init persist", "cleanup", "stop"] ("Array Constant")
        n275 = call "obj_DataLog Table Columns.vi"("method"=t_Datalog_Table_Columns_Methods."#columns") -> ("#columns"=w694:i32)  [unwired: 9 in, 5 out]
        n276 = for {
          N: w694 -> [_]
          shift-right: [w701] -> w693
          shift-left: w695 -> [w702]
          tunnel: w692 -> [w703]
          shift-right: [w699] -> w691
          shift-left: errorcluster {"status"=FALSE, "code"=0, "source"=""} -> [w698]
          i -> [w700]
          n277 = case shown="No Error" w698 {
            selector: w698 -> [w705 w776]
            tunnel: w703 -> [w711 _]
            tunnel: w702 -> [w710 w777]
            tunnel: [w709 w777] -> w701
            tunnel: w700 -> [w708 _]
            tunnel: [w707 w776] -> w699
            frame No Error {
              n278 = call "obj_DataLog Table Columns.vi"("method"=t_Datalog_Table_Columns_Methods."index", "index"=w708, "error in (no error)"=w705) -> ("tag config"=w712:T13, "mode"=w704:T21, "error out"=w706:errorcluster)  [unwired: 7 in, 3 out]
              n279 = case shown="\"interpolate\", \"at+interpolate\"" w704 {
                tunnel: w712 -> [_ w716]
                tunnel: w711 -> [_ w722]
                tunnel: w710 -> [w714 w721]
                tunnel: [w714 w720] -> w709
                tunnel: w708 -> [_ w719]
                tunnel: [w715 w718] -> w707
                tunnel: w706 -> [w715 w717]
                frame "at" {
                }
                frame "interpolate", "at+interpolate" {
                  n280 = stacked-sequence {
                    tunnel: w716 -> [_ w728 _]
                    tunnel: w722 -> [_ w735 _]
                    tunnel: w721 -> [_ w734 _]
                    tunnel: [_ w733 _] -> w720
                    tunnel: w719 -> [w725 w732 w775]
                    tunnel: [_ w731 _] -> w718
                    tunnel: w717 -> [_ w730 _]
                    frame #0 {
                      n281 = Bundle("element"=-1, w725) -> (w724:cluster{"element":i32, i32})  [unwired: 1 in]
                      n282 = call <vilib>:"Set Busy.vi"() -> ()  [unwired: 10 in, 2 out]
                      n283 = property on="log table" class="Tbl (strict)"("Active Cell:Active Cell"=w724, "Active Cell:Cell Background Color"=u32 32768, "Active Cell:Cell FG Color"=u32 16777215) -> ()  [unwired: 2 in, 2 out]
                    }
                    frame #1 {
                      n284 = Unbundle By Name(w728) -> ("value"=w729:T12)
                      n285 = case shown="\"string\"" w729 {
                        tunnel: w728 -> [w747 w764]
                        tunnel: w735 -> [w745 w762]
                        tunnel: w734 -> [w744 w761]
                        tunnel: [w741 w759] -> w733
                        tunnel: w732 -> [w740 w758]
                        tunnel: [w738 w756] -> w731
                        tunnel: w730 -> [w737 w755]
                        frame "number" {
                          n286 = Unbundle By Name(w747) -> ("name"=w746:string)
                          n287 = local read "query"() -> (w736:T3)
                          n288 = call "obj_ClientSrv Client Access State.vi"("error in (no error)"=w737) -> ("certificate"=w749:string, "error out"=w751:errorcluster)  [unwired: 13 in]
                          n289 = Index Array(array=w744, index=w740) -> (element=w743:T11)
                          n290 = call-by-ref "?"(reference=w736, error in=w751, "method"=t_DataLog_Query_Served_Methods."interpolate", "certificate"=w749, "tag"=w746, "database (current)"=w745) -> (error out=w752:errorcluster, "values"=w742:dbl[], 15:"error out"=w750:errorcluster)  [unwired: 6 in, 5 out]
                          n291 = call "Library Remote Call Error Merger.vi"("call by reference node error"=w752, "called VI error (no error)"=w750) -> ("error out"=w738:errorcluster)  [unwired: 13 in]
                          n292 = Bundle By Name(cluster=w743, "values"=w742) -> (w739:T11)
                          n293 = Replace Array Subset(array=w744, new element=w739, index=w740) -> (w741:T20)
                        }
                        frame "string" {
                          n294 = Unbundle By Name(w764) -> ("name"=w763:string)
                          n295 = local read "query"() -> (w765:T3)
                          n296 = call "obj_ClientSrv Client Access State.vi"("error in (no error)"=w755) -> ("certificate"=w767:string, "error out"=w769:errorcluster)  [unwired: 13 in]
                          n297 = Index Array(array=w761, index=w758) -> (element=w760:T11)
                          n298 = call-by-ref "?"(reference=w765, error in=w769, "method"=t_DataLog_Query_Served_Methods."interpolate str", "certificate"=w767, "tag"=w763, "database (current)"=w762) -> (error out=w770:errorcluster, "values"=w753:dbl[], "strings"=w754:string[], 15:"error out"=w768:errorcluster)  [unwired: 6 in, 4 out]
                          n299 = Bundle By Name(cluster=w760, "values"=w753, "strings"=w754) -> (w757:T11)
                          n300 = call "Library Remote Call Error Merger.vi"("call by reference node error"=w770, "called VI error (no error)"=w768) -> ("error out"=w756:errorcluster)  [unwired: 13 in]
                          n301 = Replace Array Subset(array=w761, new element=w757, index=w758) -> (w759:T20)
                        }
                      }
                    }
                    frame #2 {
                      n302 = Bundle("element"=-1, w775) -> (w774:cluster{"element":i32, i32})  [unwired: 1 in]
                      n303 = call <vilib>:"Unset Busy.vi"() -> ()  [unwired: 11 in, 1 out]
                      n304 = property on="log table" class="Tbl (strict)"("Active Cell:Active Cell"=w774, "Active Cell:Cell Background Color"=u32 15790320, "Active Cell:Cell FG Color"=u32 0) -> ()  [unwired: 2 in, 2 out]
                    }
                  }
                }
              }
            }
            frame Error {
            }
          }
        }
        n305 = call "Library Log Error to Window.vi"("error in (no error)"=w691) -> ("dup error"=w688:errorcluster)  [unwired: 13 in, 1 out]
        n306 = Select(t=w690, s=w688, f=w687) -> (s? t:f=w689:T6[])
      }
      frame "ret tabulate" {
        n307 = Build Array (concatenate)(t_DataLog_Log_Table_States."tabulate" ("states"), w789) -> (w785:T6[])
      }
      frame "ret free" {
        # "ignore errors:\nthis serves to free server-side\nmemory but is not essential"
        n308 = local read "query"() -> (w793:T3)
        n309 = call "obj_ClientSrv Client Access State.vi"() -> ("certificate"=w795:string, "error out"=w796:errorcluster)  [unwired: 14 in]
        n310 = call-by-ref "?"(reference=w793, error in=w796, "method"=t_DataLog_Query_Served_Methods."clear", "certificate"=w795) -> ()  [unwired: 8 in, 8 out]
      }
      frame "num. exclude", "num. include" {
        w808 = T6[] [enum."count rows", enum."time headers", enum."tabulate"] items=["empty queue", "retrieve", "ret clear", "ret presize", "ret range", "ret merge", "ret at", "ret step", "ret times", "ret interpolate", "ret tabulate", "ret free", "num. exclude", "num. include", "str. exclude", "str. include", "time graph", "graph xy", "xy query", "xy check", "xy open", "xy set", "xy correlate", "xy run", "export", "show string", "count rows", "time headers", "tabulate", "abort query", "clear query", "clear all", "set database", "deselect", "ablement", "resize", "initialize", "init refs", "init databases", "init persist", "cleanup", "stop"] ("Array Constant")
        n311 = local read "comparison"() -> (w807:T2)
        n312 = case shown="Default" w807 {
          selector: w807 -> [_ w832]
          tunnel: [w823 w844] -> w818
          tunnel: w817 -> [w823 w843]
          tunnel: w816 -> [w824 w842]
          tunnel: [w824 w841] -> w815
          tunnel: [w821 w840] -> w813
          tunnel: w812 -> [w822 w839]
          tunnel: w811 -> [_ w835]
          tunnel: w810 -> [w825 w833]
          frame "all" {
            n313 = for {
              tunnel: w825 -> [w828]
              tunnel: w822 -> [w827] mode=indexing
              tunnel: [w826] -> w821 mode=indexing
              n314 = case shown="\"num. include\"" w828 {
                tunnel: [w829 -1 0] -> w826
                tunnel: w827 -> [w829 _ _]
                frame Default {
                }
                frame "num. exclude" {
                }
                frame "num. include" {
                }
              }
            }
          }
          frame Default {
            n315 = call "obj_DataLog Table Columns.vi"("method"=t_Datalog_Table_Columns_Methods."index", "index"=w835) -> ("tag config"=w837:T13, "mode"=w836:T21)  [unwired: 8 in, 4 out]
            n316 = case shown="\"at\"" w836 {
              tunnel: w843 -> [w853 w912]
              tunnel: w835 -> [w849 w911]
              tunnel: w837 -> [_ _]
              tunnel: [w853 w912] -> w844
              tunnel: w842 -> [w852 w910]
              tunnel: [w852 w909] -> w841
              tunnel: w839 -> [w851 w908]
              tunnel: [w848 w907] -> w840
              tunnel: "number" -> [w846 w905]
              tunnel: w832 -> [w847 w904]
              tunnel: w833 -> [w845 w903]
              frame "interpolate", "at+interpolate" {
                n317 = Index Array(array=w853, index=w849) -> (element=w854:T11)
                n318 = Unbundle By Name(w854) -> ("values"=w850:dbl[])
                n319 = for {
                  tunnel: w850 -> [w861] mode=indexing
                  shift-right: [w857] -> w848
                  shift-left: w851 -> [w858]
                  tunnel: w847 -> [w862]
                  tunnel: w846 -> [w860]
                  tunnel: w845 -> [w859]
                  i -> [w855]
                  n320 = case shown="\"~=NaN\"" w862 {
                    tunnel: w861 -> [_ w880 w883 w886 w889 w892 w895 w897 w900]
                    tunnel: w860 -> [_ w879 w882 w885 w888 w891 w894 _ _]
                    tunnel: [TRUE w878 w881 w884 w887 w890 w893 w896 w898] -> w856
                    frame "all" {
                    }
                    frame "==" {
                      n321 = Equal?(x=w880, y=w879) -> (x = y?=w878:bool)
                    }
                    frame "~=" {
                      n322 = Not Equal?(x=w883, y=w882) -> (x != y?=w881:bool)
                    }
                    frame ">" {
                      n323 = Greater?(x=w886, y=w885) -> (0:w884:bool)
                    }
                    frame ">=" {
                      n324 = Less?(x=w889, y=w888) -> (x < y?=w887:bool)
                    }
                    frame "<=" {
                      n325 = Less Or Equal?(x=w892, y=w891) -> (x <= y?=w890:bool)
                    }
                    frame "<" {
                      n326 = Less?(x=w895, y=w894) -> (x < y?=w893:bool)
                    }
                    frame "==NaN" {
                      n327 = Not A Number/Path/Refnum?(number/path/refnum=w897) -> (NaN/Path/Refnum?=w896:bool)
                    }
                    frame "~=NaN" {
                      n328 = Not A Number/Path/Refnum?(number/path/refnum=w900) -> (NaN/Path/Refnum?=w899:bool)
                      n329 = Not(x=w899) -> (.not. x?=w898:bool)
                    }
                  }
                  n330 = case shown="True" w856 {
                    tunnel: w859 -> [_ w867]
                    tunnel: w858 -> [w863 w866]
                    tunnel: [w863 w865] -> w857
                    tunnel: w855 -> [_ w864]
                    frame False {
                    }
                    frame True {
                      n331 = case shown="\"num. include\"" w867 {
                        tunnel: [w868 w869 w873] -> w865
                        tunnel: w866 -> [w868 w872 w876]
                        tunnel: w864 -> [_ w871 w875]
                        frame Default {
                        }
                        frame "num. exclude" {
                          n332 = Replace Array Subset(array=w872, new element=-1, index=w871) -> (w869:i32[])
                        }
                        frame "num. include" {
                          n333 = Replace Array Subset(array=w876, new element=0, index=w875) -> (w873:i32[])
                        }
                      }
                    }
                  }
                }
              }
              frame "at" {
                n334 = Index Array(array=w912, index=w911) -> (element=w913:T11)
                n335 = Unbundle By Name(w913) -> ("values"=w902:dbl[], "times"=w901:dbl[])
                n336 = for {
                  shift-right: [w928] -> w909
                  shift-left: w910 -> [w929]
                  shift-right: [w926] -> _
                  shift-left: 0 -> [w927]
                  shift-right: [w920] -> w907
                  shift-left: w908 -> [w919]
                  tunnel: w905 -> [w924]
                  tunnel: w904 -> [w923]
                  tunnel: w903 -> [w921]
                  tunnel: w902 -> [w915] mode=indexing
                  tunnel: w901 -> [w914] mode=indexing
                  n337 = Search 1D Array(1D array=w929, element=w914, start index (0)=w927) -> (index of element=w925:i32)
                  n338 = case shown="\"~=NaN\"" w923 {
                    tunnel: w915 -> [_ w948 w951 w954 w957 w960 w963 w964 w967]
                    tunnel: w924 -> [_ w947 w950 w953 w956 w959 w962 _ _]
                    tunnel: [TRUE w946 w949 w952 w955 w958 w961 w965 w966] -> w922
                    frame "all" {
                    }
                    frame "==" {
                      n339 = Equal?(x=w948, y=w947) -> (x = y?=w946:bool)
                    }
                    frame "~=" {
                      n340 = Not Equal?(x=w951, y=w950) -> (x != y?=w949:bool)
                    }
                    frame ">" {
                      n341 = Greater?(x=w954, y=w953) -> (0:w952:bool)
                    }
                    frame ">=" {
                      n342 = Less?(x=w957, y=w956) -> (x < y?=w955:bool)
                    }
                    frame "<=" {
                      n343 = Less Or Equal?(x=w960, y=w959) -> (x <= y?=w958:bool)
                    }
                    frame "<" {
                      n344 = Less?(x=w963, y=w962) -> (x < y?=w961:bool)
                    }
                    frame "==NaN" {
                      n345 = Not A Number/Path/Refnum?(number/path/refnum=w964) -> (NaN/Path/Refnum?=w965:bool)
                    }
                    frame "~=NaN" {
                      n346 = Not A Number/Path/Refnum?(number/path/refnum=w967) -> (NaN/Path/Refnum?=w968:bool)
                      n347 = Not(x=w968) -> (.not. x?=w966:bool)
                    }
                  }
                  n348 = Greater Or Equal To 0?(x=w925) -> (x >= 0?=w930:bool)
                  n349 = case shown="False" w930 {
                    tunnel: w929 -> [w970 w975]
                    tunnel: [w970 w975] -> w928
                    tunnel: w927 -> [w971 _]
                    tunnel: [w971 w973] -> w926
                    tunnel: w925 -> [_ w974]
                    tunnel: [w972 w974] -> w916
                    tunnel: w914 -> [w969 _]
                    frame False {
                      n350 = Search 1D Array(1D array=w970, element=w969) -> (index of element=w972:i32)  [unwired: 1 in]
                    }
                    frame True {
                      n351 = Increment(x=w974) -> (x+1=w973:i32)
                    }
                  }
                  n352 = Greater Or Equal To 0?(x=w916) -> (x >= 0?=w917:bool)
                  n353 = And(x=w922, y=w917) -> (x .and. y?=w918:bool)
                  n354 = case shown="True" w918 {
                    tunnel: w921 -> [_ w935]
                    tunnel: w919 -> [w931 w934]
                    tunnel: [w931 w933] -> w920
                    tunnel: w916 -> [_ w932]
                    frame False {
                    }
                    frame True {
                      n355 = case shown="\"num. include\"" w935 {
                        tunnel: [w936 w937 w941] -> w933
                        tunnel: w934 -> [w936 w940 w944]
                        tunnel: w932 -> [_ w939 w943]
                        frame Default {
                        }
                        frame "num. exclude" {
                          n356 = Replace Array Subset(array=w940, new element=-1, index=w939) -> (w937:i32[])
                        }
                        frame "num. include" {
                          n357 = Replace Array Subset(array=w944, new element=0, index=w943) -> (w941:i32[])
                        }
                      }
                    }
                  }
                }
              }
            }
          }
        }
        n358 = Build Array (concatenate)(w808, w820) -> (w809:T6[])
      }
      frame "str. exclude", "str. include" {
        w980 = T6[] [enum."count rows", enum."time headers", enum."tabulate"] items=["empty queue", "retrieve", "ret clear", "ret presize", "ret range", "ret merge", "ret at", "ret step", "ret times", "ret interpolate", "ret tabulate", "ret free", "num. exclude", "num. include", "str. exclude", "str. include", "time graph", "graph xy", "xy query", "xy check", "xy open", "xy set", "xy correlate", "xy run", "export", "show string", "count rows", "time headers", "tabulate", "abort query", "clear query", "clear all", "set database", "deselect", "ablement", "resize", "initialize", "init refs", "init databases", "init persist", "cleanup", "stop"] ("Array Constant")
        n359 = local read "match"() -> (w979:T1)
        n360 = case shown="Default" w979 {
          selector: w979 -> [_ w1005]
          tunnel: [w995 w1016] -> w990
          tunnel: w989 -> [w995 w1015]
          tunnel: w988 -> [w996 w1014]
          tunnel: [w996 w1013] -> w987
          tunnel: [w993 w1012] -> w985
          tunnel: w984 -> [w994 w1011]
          tunnel: w983 -> [_ w1007]
          tunnel: w982 -> [w997 w1006]
          frame "all" {
            n361 = for {
              tunnel: w997 -> [w1000]
              tunnel: w994 -> [w999] mode=indexing
              tunnel: [w998] -> w993 mode=indexing
              n362 = case shown="\"str. include\"" w1000 {
                tunnel: [w1001 -1 0] -> w998
                tunnel: w999 -> [w1001 _ _]
                frame Default {
                }
                frame "str. exclude" {
                }
                frame "str. include" {
                }
              }
            }
          }
          frame Default {
            n363 = call "obj_DataLog Table Columns.vi"("method"=t_Datalog_Table_Columns_Methods."index", "index"=w1007) -> ("tag config"=w1009:T13, "mode"=w1008:T21)  [unwired: 8 in, 4 out]
            n364 = case shown="\"at\"" w1008 {
              tunnel: w1015 -> [w1026 w1110]
              tunnel: w1007 -> [w1022 w1109]
              tunnel: w1009 -> [_ _]
              tunnel: [w1026 w1110] -> w1016
              tunnel: w1014 -> [w1025 w1108]
              tunnel: [w1025 w1107] -> w1013
              tunnel: w1011 -> [w1024 w1106]
              tunnel: [w1021 w1105] -> w1012
              tunnel: "string" -> [w1019 w1103]
              tunnel: w1005 -> [w1020 w1102]
              tunnel: w1006 -> [w1018 w1101]
              frame "interpolate", "at+interpolate" {
                n365 = Index Array(array=w1026, index=w1022) -> (element=w1027:T11)
                n366 = Unbundle By Name(w1027) -> ("strings"=w1017:string[], "values"=w1023:dbl[])
                n367 = for {
                  tunnel: w1023 -> [w1031] mode=indexing
                  shift-right: [w1034] -> w1021
                  shift-left: w1024 -> [w1035]
                  tunnel: w1020 -> [w1038]
                  tunnel: w1019 -> [w1037]
                  tunnel: w1018 -> [w1036]
                  tunnel: w1017 -> [w1030]
                  i -> [w1032]
                  n368 = To Long Integer(number=w1031) -> (32bit integer=w1029:i32)
                  n369 = Index Array(array=w1030, index=w1029) -> (element=w1028:string)
                  n370 = case shown="\"contains c.i.\"" w1038 {
                    tunnel: w1028 -> [_ w1056 w1059 w1063 w1069 w1073 w1079 w1084 w1091 w1093 w1096]
                    tunnel: w1037 -> [_ w1055 w1058 w1062 w1068 w1072 w1078 w1080 w1087 _ _]
                    tunnel: [TRUE w1054 w1057 w1060 w1066 w1070 w1076 w1081 w1088 w1094 w1097] -> w1033
                    frame "all" {
                    }
                    frame "==" {
                      n371 = Equal?(x=w1056, y=w1055) -> (x = y?=w1054:bool)
                    }
                    frame "~=" {
                      n372 = Not Equal?(x=w1059, y=w1058) -> (x != y?=w1057:bool)
                    }
                    frame "contains" {
                      n373 = Search/Split String(string=w1063, search string/char (-)=w1062) -> (offset of match=w1061:i32)  [unwired: 1 in, 2 out]
                      n374 = Greater Or Equal To 0?(x=w1061) -> (x >= 0?=w1060:bool)
                    }
                    frame "contains c.i." {
                      n375 = To Lower Case(string=w1069) -> (all lower case string=w1065:string)
                      n376 = To Lower Case(string=w1068) -> (all lower case string=w1064:string)
                      n377 = Search/Split String(string=w1065, search string/char (-)=w1064) -> (offset of match=w1067:i32)  [unwired: 1 in, 2 out]
                      n378 = Greater Or Equal To 0?(x=w1067) -> (x >= 0?=w1066:bool)
                    }
                    frame "lacks" {
                      n379 = Search/Split String(string=w1073, search string/char (-)=w1072) -> (offset of match=w1071:i32)  [unwired: 1 in, 2 out]
                      n380 = Less Than 0?(x=w1071) -> (x < 0?=w1070:bool)
                    }
                    frame "lacks c.i." {
                      n381 = To Lower Case(string=w1079) -> (all lower case string=w1075:string)
                      n382 = To Lower Case(string=w1078) -> (all lower case string=w1074:string)
                      n383 = Search/Split String(string=w1075, search string/char (-)=w1074) -> (offset of match=w1077:i32)  [unwired: 1 in, 2 out]
                      n384 = Less Than 0?(x=w1077) -> (x < 0?=w1076:bool)
                    }
                    frame "starts with" {
                      n385 = String Length(string=w1080) -> (length=w1083:i32)
                      n386 = String Subset(string=w1084, length (rest)=w1083) -> (substring=w1082:string)  [unwired: 1 in]
                      n387 = Equal?(x=w1082, y=w1080) -> (x = y?=w1081:bool)
                    }
                    frame "starts with c.i." {
                      n388 = String Length(string=w1087) -> (length=w1090:i32)
                      n389 = To Lower Case(string=w1087) -> (all lower case string=w1085:string)
                      n390 = String Subset(string=w1091, length (rest)=w1090) -> (substring=w1089:string)  [unwired: 1 in]
                      n391 = To Lower Case(string=w1089) -> (all lower case string=w1086:string)
                      n392 = Equal?(x=w1086, y=w1085) -> (x = y?=w1088:bool)
                    }
                    frame "UNDEFINED" {
                      n393 = Equal?(x=w1093, y="UNDEFINED") -> (x = y?=w1094:bool)
                    }
                    frame "DEFINED" {
                      n394 = Not Equal?(x=w1096, y="UNDEFINED") -> (x != y?=w1097:bool)
                    }
                  }
                  n395 = case shown="True" w1033 {
                    tunnel: w1036 -> [_ w1043]
                    tunnel: w1035 -> [w1039 w1042]
                    tunnel: [w1039 w1041] -> w1034
                    tunnel: w1032 -> [_ w1040]
                    frame False {
                    }
                    frame True {
                      n396 = case shown="\"str. exclude\"" w1043 {
                        tunnel: [w1044 w1045 w1049] -> w1041
                        tunnel: w1042 -> [w1044 w1048 w1052]
                        tunnel: w1040 -> [_ w1047 w1051]
                        frame Default {
                        }
                        frame "str. exclude" {
                          n397 = Replace Array Subset(array=w1048, new element=-1, index=w1047) -> (w1045:i32[])
                        }
                        frame "str. include" {
                          n398 = Replace Array Subset(array=w1052, new element=0, index=w1051) -> (w1049:i32[])
                        }
                      }
                    }
                  }
                }
              }
              frame "at" {
                n399 = Index Array(array=w1110, index=w1109) -> (element=w1111:T11)
                n400 = Unbundle By Name(w1111) -> ("strings"=w1098:string[], "values"=w1100:dbl[], "times"=w1099:dbl[])
                n401 = for {
                  shift-right: [w1129] -> w1107
                  shift-left: w1108 -> [w1130]
                  shift-right: [w1127] -> _
                  shift-left: 0 -> [w1128]
                  shift-right: [w1124] -> w1105
                  shift-left: w1106 -> [w1123]
                  tunnel: w1103 -> [w1115]
                  tunnel: w1102 -> [w1114]
                  tunnel: w1101 -> [w1125]
                  tunnel: w1100 -> [w1119] mode=indexing
                  tunnel: w1099 -> [w1118] mode=indexing
                  tunnel: w1098 -> [w1117]
                  n402 = To Long Integer(number=w1119) -> (32bit integer=w1116:i32)
                  n403 = Index Array(array=w1117, index=w1116) -> (element=w1113:string)
                  n404 = Search 1D Array(1D array=w1130, element=w1118, start index (0)=w1128) -> (index of element=w1126:i32)
                  n405 = case shown="\"contains c.i.\"" w1114 {
                    tunnel: w1113 -> [_ w1135 w1138 w1142 w1148 w1152 w1158 w1163 w1170 w1172 w1175]
                    tunnel: w1115 -> [_ w1134 w1137 w1141 w1147 w1151 w1157 w1159 w1166 _ _]
                    tunnel: [TRUE w1133 w1136 w1139 w1145 w1149 w1155 w1160 w1167 w1173 w1176] -> w1112
                    frame "all" {
                    }
                    frame "==" {
                      n406 = Equal?(x=w1135, y=w1134) -> (x = y?=w1133:bool)
                    }
                    frame "~=" {
                      n407 = Not Equal?(x=w1138, y=w1137) -> (x != y?=w1136:bool)
                    }
                    frame "contains" {
                      n408 = Search/Split String(string=w1142, search string/char (-)=w1141) -> (offset of match=w1140:i32)  [unwired: 1 in, 2 out]
                      n409 = Greater Or Equal To 0?(x=w1140) -> (x >= 0?=w1139:bool)
                    }
                    frame "contains c.i." {
                      n410 = To Lower Case(string=w1147) -> (all lower case string=w1143:string)
                      n411 = To Lower Case(string=w1148) -> (all lower case string=w1144:string)
                      n412 = Search/Split String(string=w1144, search string/char (-)=w1143) -> (offset of match=w1146:i32)  [unwired: 1 in, 2 out]
                      n413 = Greater Or Equal To 0?(x=w1146) -> (x >= 0?=w1145:bool)
                    }
                    frame "lacks" {
                      n414 = Search/Split String(string=w1152, search string/char (-)=w1151) -> (offset of match=w1150:i32)  [unwired: 1 in, 2 out]
                      n415 = Less Than 0?(x=w1150) -> (x < 0?=w1149:bool)
                    }
                    frame "lacks c.i." {
                      n416 = To Lower Case(string=w1157) -> (all lower case string=w1153:string)
                      n417 = To Lower Case(string=w1158) -> (all lower case string=w1154:string)
                      n418 = Search/Split String(string=w1154, search string/char (-)=w1153) -> (offset of match=w1156:i32)  [unwired: 1 in, 2 out]
                      n419 = Less Than 0?(x=w1156) -> (x < 0?=w1155:bool)
                    }
                    frame "starts with" {
                      n420 = String Length(string=w1159) -> (length=w1162:i32)
                      n421 = String Subset(string=w1163, length (rest)=w1162) -> (substring=w1161:string)  [unwired: 1 in]
                      n422 = Equal?(x=w1161, y=w1159) -> (x = y?=w1160:bool)
                    }
                    frame "starts with c.i." {
                      n423 = String Length(string=w1166) -> (length=w1169:i32)
                      n424 = To Lower Case(string=w1166) -> (all lower case string=w1164:string)
                      n425 = String Subset(string=w1170, length (rest)=w1169) -> (substring=w1168:string)  [unwired: 1 in]
                      n426 = To Lower Case(string=w1168) -> (all lower case string=w1165:string)
                      n427 = Equal?(x=w1165, y=w1164) -> (x = y?=w1167:bool)
                    }
                    frame "UNDEFINED" {
                      n428 = Equal?(x=w1172, y="UNDEFINED") -> (x = y?=w1173:bool)
                    }
                    frame "DEFINED" {
                      n429 = Not Equal?(x=w1175, y="UNDEFINED") -> (x != y?=w1176:bool)
                    }
                  }
                  n430 = Greater Or Equal To 0?(x=w1126) -> (x >= 0?=w1131:bool)
                  n431 = case shown="False" w1131 {
                    tunnel: w1130 -> [w1192 w1197]
                    tunnel: [w1192 w1197] -> w1129
                    tunnel: w1128 -> [w1193 _]
                    tunnel: [w1193 w1195] -> w1127
                    tunnel: w1126 -> [_ w1196]
                    tunnel: [w1194 w1196] -> w1120
                    tunnel: w1118 -> [w1191 _]
                    frame False {
                      n432 = Search 1D Array(1D array=w1192, element=w1191) -> (index of element=w1194:i32)  [unwired: 1 in]
                    }
                    frame True {
                      n433 = Increment(x=w1196) -> (x+1=w1195:i32)
                    }
                  }
                  n434 = Greater Or Equal To 0?(x=w1120) -> (x >= 0?=w1121:bool)
                  n435 = And(x=w1112, y=w1121) -> (x .and. y?=w1122:bool)
                  n436 = case shown="True" w1122 {
                    tunnel: w1125 -> [_ w1181]
                    tunnel: w1123 -> [w1177 w1180]
                    tunnel: [w1177 w1179] -> w1124
                    tunnel: w1120 -> [_ w1178]
                    frame False {
                    }
                    frame True {
                      n437 = case shown="\"str. exclude\"" w1181 {
                        tunnel: [w1182 w1183 w1187] -> w1179
                        tunnel: w1180 -> [w1182 w1186 w1190]
                        tunnel: w1178 -> [_ w1185 w1189]
                        frame Default {
                        }
                        frame "str. exclude" {
                          n438 = Replace Array Subset(array=w1186, new element=-1, index=w1185) -> (w1183:i32[])
                        }
                        frame "str. include" {
                          n439 = Replace Array Subset(array=w1190, new element=0, index=w1189) -> (w1187:i32[])
                        }
                      }
                    }
                  }
                }
              }
            }
          }
        }
        n440 = Build Array (concatenate)(w980, w992) -> (w981:T6[])
      }
      frame "time graph" {
        n441 = call "obj_DataLog Table Columns.vi"("method"=t_Datalog_Table_Columns_Methods."#columns") -> ("#columns"=w1214:i32)  [unwired: 9 in, 5 out]
        n442 = for {
          N: w1214 -> [_]
          shift-right: [w1285] -> w1212
          shift-left: string[] [] -> [w1287]
          i -> [w1284]
          n443 = call "obj_DataLog Table Columns.vi"("method"=t_Datalog_Table_Columns_Methods."index", "index"=w1284) -> ("tag config"=w1289:T13)  [unwired: 8 in, 5 out]
          n444 = Unbundle By Name(w1289) -> ("name"=w1286:string, "value"=w1288:T12)
          n445 = case shown="\"number\"" w1288 {
            tunnel: w1287 -> [w1293 w1294]
            tunnel: w1286 -> [w1292 _]
            tunnel: [w1291 w1294] -> w1285
            frame "number" {
              n446 = Build Array (concatenate)(w1293, w1292) -> (w1291:string[])
            }
            frame "string" {
            }
          }
        }
        n447 = call "Library Resolve VI Path.vi"("VI name"="ui_Datalog Time Graph.vit", "sub path of toolkit (none)"=path "dynamic" ("subdirectory of tree (none)")) -> ("VI path"=w1200:path)  [unwired: 13 in]
        n448 = call "ui_DataLog Query Listed Strings.vi"("prompt"="Select Tag(s) to graph:", "list of strings"=w1212) -> ("OKed?"=w1203:bool, "selected strings"=w1210:string[])  [unwired: 12 in]
        n449 = case "OKed?" shown="True" w1203 {
          tunnel: w1210 -> [_ w1225]
          tunnel: w1208 -> [w1219 w1224]
          tunnel: [w1219 w1223] -> w1206
          tunnel: w1204 -> [_ w1222]
          tunnel: w1200 -> [_ w1221]
          tunnel: w1199 -> [_ w1220]
          frame False {
          }
          frame True {
            n450 = stacked-sequence {
              seq-local: [w1228 _] -> [_ w1269]
              seq-local: [w1227 _] -> [_ w1274]
              seq-local: [w1226 _] -> [_ w1272]
              tunnel: w1225 -> [w1234 _]
              tunnel: w1224 -> [w1231 _]
              tunnel: [w1230 _] -> w1223
              tunnel: w1222 -> [w1229 _]
              tunnel: w1221 -> [_ w1281]
              tunnel: w1220 -> [_ w1278]
              frame #0 {
                n451 = for {
                  tunnel: w1234 -> [w1260] mode=indexing
                  tunnel: [w1258] -> w1233 mode=indexing
                  tunnel: [w1257] -> w1226 mode=indexing
                  tunnel: [w1256] -> w1232 mode=indexing
                  n452 = call "obj_DataLog Table Columns.vi"("method"=t_Datalog_Table_Columns_Methods."get by name", "tag"=w1260) -> ("column index"=w1258:i32, "tag config"=w1257:T13, "mode"=w1256:T21)  [unwired: 8 in, 3 out]
                }
                n453 = for {
                  tunnel: w1233 -> [w1240] mode=indexing
                  tunnel: w1232 -> [w1241] mode=indexing
                  shift-right: [w1238] -> w1230
                  shift-left: w1231 -> [w1239]
                  tunnel: w1229 -> [w1237]
                  tunnel: [w1236] -> w1228 mode=indexing
                  tunnel: [w1235] -> w1227 mode=indexing
                  n454 = case shown="\"at\"" w1241 {
                    tunnel: w1240 -> [w1245 w1252]
                    tunnel: w1239 -> [w1248 w1255]
                    tunnel: [w1248 w1255] -> w1238
                    tunnel: w1237 -> [_ w1251]
                    tunnel: [w1246 w1253] -> w1236
                    tunnel: [FALSE TRUE] -> w1235
                    frame "at" {
                      n455 = Index Array(array=w1248, index=w1245) -> (element=w1247:T11)
                      n456 = Unbundle By Name(w1247) -> ("times"=w1244:dbl[], "values"=w1243:dbl[])
                      n457 = Bundle("times"=w1244, "values"=w1243) -> (w1246:cluster{"times":dbl[], "values":dbl[]})  [unwired: 1 in]
                    }
                    frame "interpolate", "at+interpolate" {
                      n458 = Index Array(array=w1255, index=w1252) -> (element=w1254:T11)
                      n459 = Unbundle By Name(w1254) -> ("values"=w1250:dbl[])
                      n460 = Bundle("times"=w1251, "values"=w1250) -> (w1253:cluster{"times":dbl[], "values":dbl[]})  [unwired: 1 in]
                    }
                  }
                }
              }
              frame #1 {
                n461 = Open VI Reference(vi path=w1281) -> (vi reference=w1263:refnum<vi>, error out=w1280:errorcluster)  [unwired: 5 in]
                n462 = invoke class="VI" method="Ctrl Val.Set"(reference=w1263, error in=w1280, "Control Name"="database", "Value"=w1278) -> (reference out=w1277:refnum<vi>, error out=w1276:errorcluster)  [unwired: 1 in, 3 out]
                n463 = invoke class="VI" method="Ctrl Val.Set"(reference=w1277, error in=w1276, "Control Name"="interpolated?", "Value"=w1274) -> (error out=w1271:errorcluster)  [unwired: 1 in, 4 out]
                n464 = invoke class="VI" method="Ctrl Val.Set"(reference=w1263, error in=w1271, "Control Name"="tag configs", "Value"=w1272) -> (reference out=w1268:refnum<vi>, error out=w1270:errorcluster)  [unwired: 1 in, 3 out]
                n465 = invoke class="VI" method="Ctrl Val.Set"(reference=w1268, error in=w1270, "Control Name"="time graph", "Value"=w1269) -> (error out=w1264:errorcluster)  [unwired: 1 in, 4 out]
                n466 = invoke class="VI" method="Run VI"(reference=w1263, error in=w1264, "Wait until done"=FALSE, "Auto Dispose Ref"=TRUE) -> (reference out=w1261:refnum<vi>, error out=w1262:errorcluster)  [unwired: 1 in, 3 out]
                n467 = case shown="Error" w1262 {
                  selector: w1262 -> [_ w1282]
                  tunnel: w1261 -> [_ w1283]
                  frame No Error {
                  }
                  frame Error {
                    n468 = call "Library Log Error to Window.vi"("error in (no error)"=w1282) -> ()  [unwired: 13 in, 2 out]
                    n469 = Close Reference(reference=w1283) -> ()  [unwired: 1 in, 1 out]
                  }
                }
              }
            }
          }
        }
      }
      frame "graph xy" {
        n470 = while "rebuild xy list on first run or after load or recompile" {
          shift-left: _ -> [w1307]
          shift-right: [w1306] -> w1295
          stop <- FALSE continue-if-true
          n471 = Array Size(array=w1307) -> (size(s)=w1308:i32)
          n472 = case shown="0" w1308 {
            tunnel: [w1309 w1329] -> w1306
            tunnel: w1307 -> [w1310 w1329]
            frame 0 {
              n473 = while {
                shift-left: w1310 -> [w1319]
                shift-right: [w1317] -> w1309
                shift-left: _ -> [w1321]
                shift-right: [w1316] -> _
                i -> [w1324]
                stop <- w1312 continue-if-true
                n474 = To Unsigned Word Integer(number=w1324) -> (unsigned 16bit integer=w1322:u16)
                n475 = Type Cast(type=t_DataLog_Log_Table_States."initialize" ("states"), x=w1322) -> (*(type *) &x=w1318:T6)
                n476 = Format Into String(format string="%s" ("Format String"), w1318) -> (resulting string=w1316:string)  [unwired: 2 in, 1 out]
                n477 = Not Equal?(x=w1316, y=w1321) -> (x != y?=w1312:bool)
                n478 = Match Pattern(string=w1316, regular expression="^xy ") -> (offset past match=w1314:i32)  [unwired: 1 in, 3 out]
                n479 = Greater Or Equal To 0?(x=w1314) -> (x >= 0?=w1313:bool)
                n480 = And(x=w1313, y=w1312) -> (x .and. y?=w1311:bool)
                n481 = case shown="True" w1311 {
                  tunnel: w1319 -> [w1325 w1328]
                  tunnel: w1318 -> [_ w1327]
                  tunnel: [w1325 w1326] -> w1317
                  frame False {
                  }
                  frame True {
                    n482 = Build Array (concatenate)(w1328, w1327) -> (w1326:T6[])
                  }
                }
              }
            }
            frame Default {
            }
          }
        }
      }
      frame "xy query" {
        n483 = call "obj_DataLog Table Columns.vi"("method"=t_Datalog_Table_Columns_Methods."#columns") -> ("#columns"=w1334:i32)  [unwired: 9 in, 5 out]
        n484 = for {
          N: w1334 -> [_]
          shift-right: [w1364] -> w1339
          shift-left: string[] [] -> [w1366]
          i -> [w1363]
          n485 = call "obj_DataLog Table Columns.vi"("method"=t_Datalog_Table_Columns_Methods."index", "index"=w1363) -> ("tag config"=w1368:T13)  [unwired: 8 in, 5 out]
          n486 = Unbundle By Name(w1368) -> ("name"=w1365:string, "value"=w1367:T12)
          n487 = case shown="\"number\"" w1367 {
            tunnel: w1366 -> [w1372 w1373]
            tunnel: w1365 -> [w1371 _]
            tunnel: [w1370 w1373] -> w1364
            frame "number" {
              n488 = Build Array (concatenate)(w1372, w1371) -> (w1370:string[])
            }
            frame "string" {
            }
          }
        }
        n489 = call "ui_Library Query Listed String.vi"("prompt"="Select x-axis tag:", "list of strings"=w1339) -> ("OKed?"=w1337:bool, "selected string"=w1338:string)  [unwired: 12 in]
        n490 = case shown="True" w1337 {
          tunnel: w1338 -> [_ w1353]
          tunnel: w1339 -> [_ w1357]
          tunnel: w1332 -> [_ w1350]
          tunnel: [_ w1349] -> w1331
          tunnel: [_ w1348] -> w1330
          frame False {
          }
          frame True {
            n491 = Search 1D Array(1D array=w1357, element=w1353) -> (index of element=w1356:i32)  [unwired: 1 in]
            n492 = Delete From Array(array=w1357, index=w1356) -> (array with subset deleted=w1355:string[])  [unwired: 1 in, 1 out]
            n493 = call "ui_Library Query Listed String.vi"("prompt"="Select y-axis tag:", "list of strings"=w1355) -> ("OKed?"=w1351:bool, "selected string"=w1352:string)  [unwired: 12 in]
            n494 = case shown="True" w1351 {
              tunnel: w1353 -> [_ w1360]
              tunnel: w1352 -> [_ w1359]
              tunnel: w1350 -> [_ w1362]
              tunnel: [_ w1362] -> w1349
              tunnel: [_ w1358] -> w1348
              frame False {
              }
              frame True {
                n495 = Bundle By Name(cluster=T10 {"graph VI"=refnum, "x tag"="", "y tag"=""}, "y tag"=w1359, "x tag"=w1360) -> (w1358:T10)
              }
            }
          }
        }
      }
      frame "xy check" {
        n496 = Unbundle By Name(w1387) -> ("x tag"=w1386:string, "y tag"=w1383:string)
        n497 = call "obj_DataLog Table Columns.vi"("method"=t_Datalog_Table_Columns_Methods."get by name", "tag"=w1386) -> ("column index"=w1379:i32, "mode"=w1382:T21)  [unwired: 8 in, 4 out]
        n498 = call "obj_DataLog Table Columns.vi"("method"=t_Datalog_Table_Columns_Methods."get by name", "tag"=w1383) -> ("column index"=w1380:i32, "mode"=w1381:T21)  [unwired: 8 in, 4 out]
        n499 = case shown="\"at\"" w1382 {
          tunnel: w1389 -> [w1403 w1449]
          tunnel: [w1402 w1449] -> w1388
          tunnel: w1381 -> [w1404 _]
          tunnel: w1380 -> [w1401 _]
          tunnel: w1379 -> [w1400 _]
          tunnel: w1378 -> [w1399 w1448]
          tunnel: [w1398 w1448] -> w1377
          tunnel: w1376 -> [w1397 w1447]
          tunnel: [w1396 w1447] -> w1375
          tunnel: w1374 -> [w1395 _]
          frame "at" {
            n500 = case shown="\"at\"" w1404 {
              tunnel: w1403 -> [w1407 w1409]
              tunnel: [w1407 w1408] -> w1402
              tunnel: w1401 -> [_ w1413]
              tunnel: w1400 -> [_ w1414]
              tunnel: w1399 -> [w1406 w1421]
              tunnel: [w1406 w1421] -> w1398
              tunnel: w1397 -> [w1405 w1417]
              tunnel: [w1405 w1411] -> w1396
              tunnel: w1395 -> [_ w1418]
              frame "interpolate", "at+interpolate" {
              }
              frame "at" {
                n501 = Index Array(array=w1421, index=w1414) -> (element=w1420:T11)
                n502 = Index Array(array=w1421, index=w1413) -> (element=w1419:T11)
                n503 = Unbundle By Name(w1420) -> ("times"=w1415:dbl[])
                n504 = Unbundle By Name(w1419) -> ("times"=w1416:dbl[])
                n505 = for "see if all included timestamps are the same" {
                  N: w1418 -> [_]
                  shift-right: [w1432] -> w1411
                  shift-left: w1417 -> [w1432]
                  tunnel: w1416 -> [w1435]
                  tunnel: w1415 -> [w1434]
                  tunnel: w1414 -> [w1437]
                  tunnel: w1413 -> [w1436]
                  shift-right: [w1424] -> w1410
                  shift-left: TRUE -> [w1426]
                  i -> [w1438]
                  n506 = Index Array(array=w1432, index (row) #1=w1438, index (col) #1=w1437, index (row) #2=w1438, index (col) #2=w1436) -> (element #1=w1429:i32, element #2=w1433:i32)
                  n507 = Greater Or Equal To 0?(x=w1429) -> (x >= 0?=w1431:bool)
                  n508 = Greater Or Equal To 0?(x=w1429) -> (x >= 0?=w1430:bool)
                  n509 = case shown="True" w1431 {
                    tunnel: w1434 -> [_ w1442]
                    tunnel: w1429 -> [_ w1440]
                    tunnel: [-1111.0 ("timestep") w1441] -> w1428
                    frame False {
                    }
                    frame True {
                      n510 = Index Array(array=w1442, index=w1440) -> (element=w1441:dbl)
                    }
                  }
                  n511 = case shown="True" w1430 {
                    tunnel: w1435 -> [_ w1446]
                    tunnel: w1433 -> [_ w1445]
                    tunnel: [-1111.0 ("timestep") w1444] -> w1427
                    frame False {
                    }
                    frame True {
                      n512 = Index Array(array=w1446, index=w1445) -> (element=w1444:dbl)
                    }
                  }
                  n513 = Equal?(x=w1428, y=w1427) -> (x = y?=w1425:bool)
                  n514 = And(x=w1426, y=w1425) -> (x .and. y?=w1424:bool)
                }
                n515 = case shown="False" w1410 {
                  tunnel: w1409 -> [_ w1423]
                  tunnel: [_ w1423] -> w1408
                  frame False {
                    n516 = One Button Dialog(message="Both tags have \"at\" retrieval mode.\nSuch a pair of tags can only be displayed\nin an xy graph when they have values at\nthe same times for all included rows.") -> ()  [unwired: 1 in, 1 out]
                  }
                  frame True {
                  }
                }
              }
            }
          }
          frame "interpolate", "at+interpolate" {
          }
        }
      }
      frame "xy open" {
        n517 = call "Library Resolve VI Path.vi"("VI name"="ui_Datalog XY Graph.vit", "sub path of toolkit (none)"=path "dynamic" ("subdirectory of tree (none)")) -> ("VI path"=w1458:path)  [unwired: 13 in]
        n518 = Open VI Reference(vi path=w1458) -> (vi reference=w1453:refnum<vi>, error out=w1452:errorcluster)  [unwired: 5 in]
        n519 = Bundle By Name(cluster=w1455, "graph VI"=w1453) -> (w1454:T10)
        n520 = case shown="Error" w1452 {
          selector: w1452 -> [_ w1468]
          tunnel: w1451 -> [w1467 _]
          tunnel: [w1467 _] -> w1450
          frame No Error {
          }
          frame Error {
            n521 = call "Library Log Error to Window.vi"("error in (no error)"=w1468) -> ()  [unwired: 13 in, 2 out]
          }
        }
      }
      frame "xy set" {
        n522 = Unbundle By Name(w1487) -> ("graph VI"=w1486:refnum<vi>, "x tag"=w1480:string, "y tag"=w1479:string)
        n523 = invoke class="VI" method="Ctrl Val.Set"(reference=w1486, "Control Name"="database", "Value"=w1485) -> (reference out=w1482:refnum<vi>, error out=w1481:errorcluster)  [unwired: 2 in, 3 out]
        n524 = call "obj_DataLog Table Columns.vi"("method"=t_Datalog_Table_Columns_Methods."get by name", "tag"=w1480) -> ("tag config"=w1475:T13)  [unwired: 8 in, 5 out]
        n525 = call "obj_DataLog Table Columns.vi"("method"=t_Datalog_Table_Columns_Methods."get by name", "tag"=w1479) -> ("tag config"=w1471:T13)  [unwired: 8 in, 5 out]
        n526 = invoke class="VI" method="Ctrl Val.Set"(reference=w1482, error in=w1481, "Control Name"="x config", "Value"=w1475) -> (reference out=w1473:refnum<vi>, error out=w1472:errorcluster)  [unwired: 1 in, 3 out]
        n527 = invoke class="VI" method="Ctrl Val.Set"(reference=w1473, error in=w1472, "Control Name"="y config", "Value"=w1471) -> (reference out=w1469:refnum<vi>, error out=w1470:errorcluster)  [unwired: 1 in, 3 out]
        n528 = case shown="No Error" w1470 {
          selector: w1470 -> [_ w1498]
          tunnel: w1484 -> [w1496 _]
          tunnel: [w1496 _] -> w1483
          tunnel: w1469 -> [_ w1497]
          frame No Error {
          }
          frame Error {
            n529 = Close Reference(reference=w1497) -> ()  [unwired: 1 in, 1 out]
            n530 = call "Library Log Error to Window.vi"("error in (no error)"=w1498) -> ()  [unwired: 13 in, 2 out]
          }
        }
      }
      frame "xy correlate" {
        w1503 = T6[] [enum."empty queue"] items=["empty queue", "retrieve", "ret clear", "ret presize", "ret range", "ret merge", "ret at", "ret step", "ret times", "ret interpolate", "ret tabulate", "ret free", "num. exclude", "num. include", "str. exclude", "str. include", "time graph", "graph xy", "xy query", "xy check", "xy open", "xy set", "xy correlate", "xy run", "export", "show string", "count rows", "time headers", "tabulate", "abort query", "clear query", "clear all", "set database", "deselect", "ablement", "resize", "initialize", "init refs", "init databases", "init persist", "cleanup", "stop"] ("Array Constant")
        w1512 = t_Datalog_Table_Columns_Methods."get by name" ("method")
        n531 = Unbundle By Name(w1509) -> ("x tag"=w1523:string, "y tag"=w1522:string)
        n532 = call "obj_DataLog Table Columns.vi"("method"=w1512, "tag"=w1523) -> ("column index"=w1518:i32, "mode"=w1521:T21)  [unwired: 8 in, 4 out]
        n533 = call "obj_DataLog Table Columns.vi"("method"=w1512, "tag"=w1522) -> ("column index"=w1519:i32, "mode"=w1520:T21)  [unwired: 8 in, 4 out]
        n534 = case shown="\"at\"" w1521 {
          tunnel: w1520 -> [w1541 w1649]
          tunnel: w1519 -> [w1540 w1648]
          tunnel: w1518 -> [w1539 w1647]
          tunnel: w1517 -> [w1538 w1646]
          tunnel: [w1537 w1645] -> w1516
          tunnel: w1515 -> [w1536 w1644]
          tunnel: [w1535 w1643] -> w1514
          tunnel: w1513 -> [w1534 w1642]
          tunnel: [w1533 w1641] -> w1500
          tunnel: [w1532 w1640] -> w1499
          frame "interpolate", "at+interpolate" {
            n535 = case shown="\"interpolate\", \"at+interpolate\"" w1541 {
              tunnel: w1540 -> [w1545 w1588]
              tunnel: w1539 -> [w1546 w1590]
              tunnel: w1538 -> [w1553 w1593]
              tunnel: [w1553 w1593] -> w1537
              tunnel: w1536 -> [w1549 w1591]
              tunnel: [w1544 w1589] -> w1535
              tunnel: w1534 -> [w1550 w1582]
              tunnel: [w1543 w1577] -> w1533
              tunnel: [w1542 w1576] -> w1532
              frame "interpolate", "at+interpolate" {
                n536 = Index Array(array=w1553, index=w1546) -> (element=w1552:T11)
                n537 = Index Array(array=w1553, index=w1545) -> (element=w1551:T11)
                n538 = Unbundle By Name(w1552) -> ("values"=w1547:dbl[])
                n539 = Unbundle By Name(w1551) -> ("values"=w1548:dbl[])
                n540 = for {
                  N: w1550 -> [_]
                  shift-right: [w1560] -> w1544
                  shift-left: w1549 -> [w1560]
                  tunnel: w1548 -> [w1562]
                  tunnel: w1547 -> [w1561]
                  tunnel: w1546 -> [w1564]
                  tunnel: w1545 -> [w1563]
                  tunnel: [w1556] -> w1543 mode=indexing
                  tunnel: [w1555] -> w1542 mode=indexing
                  i -> [w1565]
                  n541 = Index Array(array=w1560, index (row) #1=w1565, index (col) #1=w1564, index (row) #2=w1565, index (col) #2=w1563) -> (element #1=w1557:i32, element #2=w1554:i32)
                  n542 = Greater Or Equal To 0?(x=w1557) -> (x >= 0?=w1559:bool)
                  n543 = Greater Or Equal To 0?(x=w1554) -> (x >= 0?=w1558:bool)
                  n544 = case shown="False" w1559 {
                    tunnel: w1561 -> [_ w1569]
                    tunnel: w1557 -> [_ w1567]
                    tunnel: [nan ("timestep") w1568] -> w1556
                    frame False {
                    }
                    frame True {
                      n545 = Index Array(array=w1569, index=w1567) -> (element=w1568:dbl)
                    }
                  }
                  n546 = case shown="False" w1558 {
                    tunnel: w1562 -> [_ w1573]
                    tunnel: w1554 -> [_ w1572]
                    tunnel: [nan ("timestep") w1571] -> w1555
                    frame False {
                    }
                    frame True {
                      n547 = Index Array(array=w1573, index=w1572) -> (element=w1571:dbl)
                    }
                  }
                }
              }
              frame "at" {
                n548 = Index Array(array=w1593, index #1=w1590, index #2=w1588) -> (element #1=w1592:T11, element #2=w1587:T11)
                n549 = Unbundle By Name(w1592) -> ("values"=w1580:dbl[])
                n550 = Unbundle By Name(w1587) -> ("values"=w1579:dbl[])
                n551 = Initialize Array(nan, w1582) -> (w1581:dbl[])
                n552 = Initialize Array(nan, w1582) -> (w1586:dbl[])
                n553 = for {
                  N: w1582 -> [_]
                  shift-right: [w1606] -> w1589
                  shift-left: w1591 -> [w1606]
                  tunnel: w1590 -> [w1608]
                  tunnel: w1588 -> [w1607]
                  shift-right: [w1599] -> w1575
                  shift-left: w1586 -> [w1600]
                  shift-right: [w1603] -> w1574
                  shift-left: -1 -> [w1604]
                  shift-right: [w1594] -> w1578
                  shift-left: w1581 -> [w1601]
                  tunnel: w1580 -> [w1598]
                  tunnel: w1579 -> [w1596]
                  i -> [w1609]
                  n554 = Index Array(array=w1606, index (row) #1=w1609, index (col) #1=w1608, index (row) #2=w1609, index (col) #2=w1607) -> (element #1=w1597:i32, element #2=w1595:i32)
                  n555 = Greater Or Equal To 0?(x=w1597) -> (x >= 0?=w1605:bool)
                  n556 = Greater Or Equal To 0?(x=w1595) -> (x >= 0?=w1602:bool)
                  n557 = case shown="True" w1605 {
                    tunnel: w1604 -> [w1613 w1620]
                    tunnel: [w1612 w1619] -> w1603
                    tunnel: w1602 -> [_ w1624]
                    tunnel: w1601 -> [w1611 w1623]
                    tunnel: w1600 -> [w1610 w1622]
                    tunnel: [w1610 w1621] -> w1599
                    tunnel: w1598 -> [_ w1618]
                    tunnel: w1597 -> [_ w1617]
                    tunnel: w1596 -> [_ w1616]
                    tunnel: w1595 -> [_ w1615]
                    tunnel: [w1611 w1614] -> w1594
                    frame False {
                      n558 = Increment(x=w1613) -> (x+1=w1612:i32)
                    }
                    frame True {
                      n559 = case shown="True" w1624 {
                        tunnel: w1623 -> [w1625 w1639]
                        tunnel: w1622 -> [w1626 w1638]
                        tunnel: [w1626 w1637] -> w1621
                        tunnel: w1620 -> [w1627 w1636]
                        tunnel: [w1627 w1635] -> w1619
                        tunnel: w1618 -> [_ w1634]
                        tunnel: w1617 -> [_ w1633]
                        tunnel: w1616 -> [_ w1632]
                        tunnel: w1615 -> [_ w1629]
                        tunnel: [w1625 w1628] -> w1614
                        frame False {
                        }
                        frame True {
                          n560 = Increment(x=w1636) -> (x+1=w1635:i32)
                          n561 = Index Array(array=w1634, index=w1633) -> (element=w1631:dbl)
                          n562 = Replace Array Subset(array=w1639, new element=w1631, index=w1635) -> (w1628:dbl[])
                          n563 = Index Array(array=w1632, index=w1629) -> (element=w1630:dbl)
                          n564 = Replace Array Subset(array=w1638, new element=w1630, index=w1635) -> (w1637:dbl[])
                        }
                      }
                    }
                  }
                }
                n565 = Reshape Array(w1578, w1574) -> (w1577:dbl[])
                n566 = Reshape Array(w1575, w1574) -> (w1576:dbl[])
              }
            }
          }
          frame "at" {
            n567 = case shown="\"at\"" w1649 {
              tunnel: w1648 -> [w1664 w1719]
              tunnel: w1647 -> [w1666 w1720]
              tunnel: w1646 -> [w1669 w1727]
              tunnel: [w1669 w1727] -> w1645
              tunnel: w1644 -> [w1667 w1723]
              tunnel: [w1665 w1718] -> w1643
              tunnel: w1642 -> [w1658 w1724]
              tunnel: [w1653 w1717] -> w1641
              tunnel: [w1652 w1716] -> w1640
              frame "interpolate", "at+interpolate" {
                n568 = Index Array(array=w1669, index #1=w1666, index #2=w1664) -> (element #1=w1668:T11, element #2=w1663:T11)
                n569 = Unbundle By Name(w1668) -> ("values"=w1656:dbl[])
                n570 = Unbundle By Name(w1663) -> ("values"=w1655:dbl[])
                n571 = Initialize Array(nan, w1658) -> (w1657:dbl[])
                n572 = Initialize Array(nan, w1658) -> (w1662:dbl[])
                n573 = for {
                  N: w1658 -> [_]
                  shift-right: [w1682] -> w1665
                  shift-left: w1667 -> [w1682]
                  tunnel: w1666 -> [w1684]
                  tunnel: w1664 -> [w1683]
                  shift-right: [w1677] -> w1651
                  shift-left: w1662 -> [w1678]
                  shift-right: [w1680] -> w1650
                  shift-left: -1 -> [w1681]
                  shift-right: [w1672] -> w1654
                  shift-left: w1657 -> [w1679]
                  tunnel: w1656 -> [w1676]
                  tunnel: w1655 -> [w1674]
                  i -> [w1685]
                  n574 = Index Array(array=w1682, index (row) #1=w1685, index (col) #1=w1684, index (row) #2=w1685, index (col) #2=w1683) -> (element #1=w1675:i32, element #2=w1673:i32)
                  n575 = Greater Or Equal To 0?(x=w1675) -> (x >= 0?=w1670:bool)
                  n576 = Greater Or Equal To 0?(x=w1673) -> (x >= 0?=w1671:bool)
                  n577 = case shown="True" w1671 {
                    tunnel: w1681 -> [w1689 w1697]
                    tunnel: [w1688 w1696] -> w1680
                    tunnel: w1679 -> [w1687 w1700]
                    tunnel: w1678 -> [w1686 w1699]
                    tunnel: [w1686 w1698] -> w1677
                    tunnel: w1676 -> [_ w1695]
                    tunnel: w1675 -> [_ w1694]
                    tunnel: w1674 -> [_ w1693]
                    tunnel: w1673 -> [_ w1692]
                    tunnel: [w1687 w1691] -> w1672
                    tunnel: w1670 -> [_ w1690]
                    frame False {
                      n578 = Increment(x=w1689) -> (x+1=w1688:i32)
                    }
                    frame True {
                      n579 = case shown="True" w1690 {
                        tunnel: w1700 -> [w1701 w1715]
                        tunnel: w1699 -> [w1702 w1714]
                        tunnel: [w1702 w1713] -> w1698
                        tunnel: w1697 -> [w1703 w1712]
                        tunnel: [w1703 w1711] -> w1696
                        tunnel: w1695 -> [_ w1710]
                        tunnel: w1694 -> [_ w1709]
                        tunnel: w1693 -> [_ w1708]
                        tunnel: w1692 -> [_ w1705]
                        tunnel: [w1701 w1704] -> w1691
                        frame False {
                        }
                        frame True {
                          n580 = Increment(x=w1712) -> (x+1=w1711:i32)
                          n581 = Index Array(array=w1710, index=w1709) -> (element=w1707:dbl)
                          n582 = Replace Array Subset(array=w1715, new element=w1707, index=w1711) -> (w1704:dbl[])
                          n583 = Index Array(array=w1708, index=w1705) -> (element=w1706:dbl)
                          n584 = Replace Array Subset(array=w1714, new element=w1706, index=w1711) -> (w1713:dbl[])
                        }
                      }
                    }
                  }
                }
                n585 = Reshape Array(w1654, w1650) -> (w1653:dbl[])
                n586 = Reshape Array(w1651, w1650) -> (w1652:dbl[])
              }
              frame "at" {
                n587 = Index Array(array=w1727, index=w1720) -> (element=w1726:T11)
                n588 = Index Array(array=w1727, index=w1719) -> (element=w1725:T11)
                n589 = Unbundle By Name(w1726) -> ("values"=w1721:dbl[])
                n590 = Unbundle By Name(w1725) -> ("values"=w1722:dbl[])
                n591 = for {
                  N: w1724 -> [_]
                  shift-right: [w1734] -> w1718
                  shift-left: w1723 -> [w1734]
                  tunnel: w1722 -> [w1736]
                  tunnel: w1721 -> [w1735]
                  tunnel: w1720 -> [w1738]
                  tunnel: w1719 -> [w1737]
                  tunnel: [w1730] -> w1717 mode=indexing
                  tunnel: [w1729] -> w1716 mode=indexing
                  i -> [w1739]
                  n592 = Index Array(array=w1734, index (row) #1=w1739, index (col) #1=w1738, index (row) #2=w1739, index (col) #2=w1737) -> (element #1=w1731:i32, element #2=w1728:i32)
                  n593 = Greater Or Equal To 0?(x=w1731) -> (x >= 0?=w1733:bool)
                  n594 = Greater Or Equal To 0?(x=w1728) -> (x >= 0?=w1732:bool)
                  n595 = case shown="False" w1733 {
                    tunnel: w1735 -> [_ w1743]
                    tunnel: w1731 -> [_ w1741]
                    tunnel: [nan ("timestep") w1742] -> w1730
                    frame False {
                    }
                    frame True {
                      n596 = Index Array(array=w1743, index=w1741) -> (element=w1742:dbl)
                    }
                  }
                  n597 = case shown="False" w1732 {
                    tunnel: w1736 -> [_ w1747]
                    tunnel: w1728 -> [_ w1746]
                    tunnel: [nan ("timestep") w1745] -> w1729
                    frame False {
                    }
                    frame True {
                      n598 = Index Array(array=w1747, index=w1746) -> (element=w1745:dbl)
                    }
                  }
                }
              }
            }
          }
        }
        n599 = Unbundle By Name(w1509) -> ("graph VI"=w1508:refnum<vi>)
        n600 = Bundle(w1500, w1499) -> (w1501:cluster{dbl[], dbl[]})  [unwired: 1 in]
        n601 = invoke class="VI" method="Ctrl Val.Set"(reference=w1508, "Control Name"="xy graph", "Value"=w1501) -> (reference out=w1507:refnum<vi>, error out=w1506:errorcluster)  [unwired: 2 in, 3 out]
        n602 = case shown="Error" w1506 {
          selector: w1506 -> [w1528 w1531]
          tunnel: w1507 -> [_ w1530]
          tunnel: [w1528 w1529] -> w1502
          frame No Error {
          }
          frame Error {
            n603 = Close Reference(reference=w1530) -> ()  [unwired: 1 in, 1 out]
            n604 = call "Library Log Error to Window.vi"("error in (no error)"=w1531) -> ("dup error"=w1529:errorcluster)  [unwired: 13 in, 1 out]
          }
        }
        n605 = Select(t=w1503, s=w1502, f=w1504) -> (s? t:f=w1505:T6[])
      }
      frame "xy run" {
        n606 = Unbundle By Name(w1749) -> ("graph VI"=w1748:refnum<vi>)
        n607 = invoke class="VI" method="Run VI"(reference=w1748, "Wait until done"=FALSE, "Auto Dispose Ref"=TRUE) -> (reference out=w1753:refnum<vi>, error out=w1752:errorcluster)  [unwired: 2 in, 3 out]
        n608 = case shown="Error" w1752 {
          selector: w1752 -> [_ w1763]
          tunnel: w1753 -> [_ w1764]
          frame No Error {
          }
          frame Error {
            n609 = call "Library Log Error to Window.vi"("error in (no error)"=w1763) -> ()  [unwired: 13 in, 2 out]
            n610 = Close Reference(reference=w1764) -> ()  [unwired: 1 in, 1 out]
          }
        }
      }
      frame "export" {
        n611 = stacked-sequence {
          seq-local: [_ w1780 _ _] -> [_ _ w1817 _]
          seq-local: [_ w1779 _ _] -> [_ _ w1818 _]
          tunnel: w1775 -> [_ _ w1826 _]
          tunnel: w1772 -> [_ _ w1815 _]
          tunnel: [_ _ w1814 _] -> w1771
          tunnel: w1774 -> [_ _ w1813 _]
          tunnel: [_ _ w1812 _] -> w1773
          tunnel: w1769 -> [_ _ w1811 _]
          tunnel: [_ _ w1810 _] -> w1768
          tunnel: w1767 -> [_ _ w1808 _]
          tunnel: [_ _ w1807 _] -> w1766
          frame #0 {
            n612 = call <vilib>:"Set Busy.vi"() -> ()  [unwired: 10 in, 2 out]
          }
          frame #1 {
            w1784 = "\n"
            # "Prepare column headers with tag names and their units."
            n613 = call "obj_DataLog Table Columns.vi"("method"=t_Datalog_Table_Columns_Methods."#columns") -> ("#columns"=w1786:i32)  [unwired: 9 in, 5 out]
            n614 = for {
              N: w1786 -> [_]
              tunnel: [w1802] -> w1780 mode=indexing
              tunnel: [w1789] -> w1783 mode=indexing
              tunnel: [w1788] -> w1785 mode=indexing
              i -> [w1803]
              w1791 = "\"" ("search string")
              w1801 = "\"" ("search string")
              n615 = call "obj_DataLog Table Columns.vi"("method"=t_Datalog_Table_Columns_Methods."index", "index"=w1803) -> ("tag config"=w1804:T13)  [unwired: 8 in, 5 out]
              n616 = Unbundle By Name(w1804) -> ("value"=w1802:T12, "name"=w1790:string, "unit"=w1797:string)
              n617 = Search and Replace String(replace all?=TRUE ("replace all? (F)"), input string=w1797, search string=w1801, replace string="\"\"" ("replace string (\"\")")) -> (result string=w1800:string)  [unwired: 4 in, 3 out]
              n618 = Concatenate Strings(",", w1801, w1800, w1801) -> (w1789:string)
              n619 = Search and Replace String(replace all?=TRUE ("replace all? (F)"), input string=w1790, search string=w1791, replace string="\"\"" ("replace string (\"\")")) -> (result string=w1792:string)  [unwired: 4 in, 3 out]
              n620 = Concatenate Strings(",", w1791, w1792, w1791) -> (w1788:string)
            }
            n621 = Concatenate Strings("time", w1785, w1784, "s", w1783, w1784) -> (w1779:string)
          }
          frame #2 {
            # "Write up to 500 lines at a time to limit memory use"
            n622 = local read "export path"() -> (w1827:path)
            n623 = call "Library New File.vi"("overwrite (F)"=TRUE, "file path"=w1827) -> ("error out"=w1821:errorcluster, "refnum"=w1823:refnum<file>)  [unwired: 8 in]
            n624 = Write to Binary File(file (use dialog)=w1823, data=w1818, error in=w1821, 5:FALSE ("prepend array or string size? (T)")) -> (refnum out=w1822:refnum<file>, error out=w1820:errorcluster)  [unwired: 2 in, 1 out]
            n625 = while {
              tunnel: w1826 -> [w1830]
              shift-right: [w1851] -> _
              shift-left: 0 -> [w1845]
              shift-right: [w1850] -> w1824
              shift-left: w1820 -> [w1849]
              tunnel: w1822 -> [w1848]
              tunnel: [w1847] -> w1819
              tunnel: w1817 -> [w1836]
              shift-right: [w1839] -> w1812
              shift-left: w1813 -> [w1840]
              shift-right: [w1841] -> w1814
              shift-left: w1815 -> [w1842]
              shift-right: [w1837] -> w1810
              shift-left: w1811 -> [w1838]
              tunnel: 500 ("y") -> [w1833]
              shift-right: [w1828] -> w1807
              shift-left: w1808 -> [w1829]
              stop <- w1846 stop-if-true
              # "row index"
              # "value types\nper column"
              # "rows"
              n626 = Array Size(array=w1836) -> (size(s)=w1831:i32)
              n627 = Subtract(x=w1830, y=w1845) -> (x-y=w1844:i32)
              n628 = Increment(x=w1831) -> (x+1=w1832:i32)
              n629 = Max & Min(x=w1844, y=w1833) -> (min(x,y)=w1843:i32)  [unwired: 1 out]
              n630 = Multiply(x=2 ("y"), y=w1832) -> (x*y=w1835:i32)
              n631 = case shown="No Error" w1849 {
                selector: w1849 -> [_ w1996]
                tunnel: w1836 -> [w1875 _]
                tunnel: w1845 -> [w1859 w1994]
                tunnel: [w1856 w1994] -> w1851
                tunnel: [w1872 w1996] -> w1850
                tunnel: w1848 -> [w1871 w1997]
                tunnel: [w1871 w1997] -> w1847
                tunnel: [w1858 TRUE] -> w1846
                tunnel: w1843 -> [w1860 _]
                tunnel: w1842 -> [w1855 w1992]
                tunnel: [w1870 w1992] -> w1841
                tunnel: w1840 -> [w1869 w1993]
                tunnel: [w1868 w1993] -> w1839
                tunnel: w1838 -> [w1865 w1991]
                tunnel: [w1862 w1991] -> w1837
                tunnel: w1835 -> [w1864 _]
                tunnel: w1830 -> [w1857 _]
                tunnel: w1829 -> [w1854 w1990]
                tunnel: [w1853 w1990] -> w1828
                frame No Error {
                  n632 = Initialize Array("", w1860, w1864) -> (w1866:string[][])
                  n633 = Decrement(x=w1864) -> (x-1=w1863:i32)
                  n634 = for {
                    N: w1860 -> [_]
                    shift-right: [w1886] -> w1861
                    shift-left: w1866 -> [w1889]
                    shift-right: [w1877] -> w1862
                    shift-left: w1865 -> [w1878]
                    shift-right: [w1884] -> w1856
                    shift-left: w1859 -> [w1881]
                    tunnel: w1863 -> [w1887]
                    shift-right: [w1882] -> w1853
                    shift-left: w1854 -> [w1882]
                    i -> [w1883]
                    n635 = Index Array(array=w1882, index=w1881) -> (element=w1876:i32)
                    n636 = Greater Or Equal To 0?(x=w1876) -> (x >= 0?=w1880:bool)
                    n637 = case shown="True" w1880 {
                      tunnel: w1889 -> [w1891 w1901]
                      tunnel: [w1891 w1899] -> w1888
                      tunnel: w1883 -> [w1892 w1898]
                      tunnel: [w1892 w1898] -> w1879
                      tunnel: w1878 -> [w1890 w1897]
                      tunnel: [w1890 w1897] -> w1877
                      tunnel: w1876 -> [_ w1896]
                      frame False {
                      }
                      frame True {
                        n638 = Index Array(array=w1897, index=w1896) -> (element=w1895:dbl)
                        n639 = Format Date/Time String(time format string (%c)="%Y/%m/%d %H:%M:%S%6u", seconds (now)=w1895) -> (date/time string=w1894:string)  [unwired: 1 in]
                        n640 = Replace Array Subset(array=w1901, new element=w1894, index (row)=w1898, index (col)=0 ("disabled index (col)")) -> (w1899:string[][])
                      }
                    }
                    n641 = Replace Array Subset(array=w1888, new element="\n", index (row)=w1879, index (col)=w1887) -> (w1886:string[][])
                    n642 = Increment(x=w1881) -> (x+1=w1884:i32)
                  }
                  n643 = for {
                    tunnel: w1875 -> [w1913] mode=indexing
                    shift-right: [w1909] -> w1868
                    shift-left: w1869 -> [w1909]
                    shift-right: [w1907] -> w1870
                    shift-left: w1855 -> [w1908]
                    shift-right: [w1902] -> w1874
                    shift-left: w1861 -> [w1906]
                    tunnel: w1860 -> [w1911]
                    tunnel: w1859 -> [w1910]
                    i -> [w1905]
                    n644 = Add(x=w1905, y=w1905) -> (x+y=w1904:i32)
                    n645 = Index Array(array=w1909, index=w1905) -> (element=w1912:T11)
                    n646 = Increment(x=w1904) -> (x+1=w1903:i32)
                    n647 = case shown="\"number\"" w1913 {
                      tunnel: w1912 -> [w1923 w1960]
                      tunnel: w1911 -> [w1921 w1958]
                      tunnel: w1910 -> [w1920 w1957]
                      tunnel: w1908 -> [w1919 w1956]
                      tunnel: [w1918 w1955] -> w1907
                      tunnel: w1905 -> [w1917 w1954]
                      tunnel: w1906 -> [w1916 w1953]
                      tunnel: w1903 -> [w1915 w1952]
                      tunnel: [w1914 w1951] -> w1902
                      frame "string" {
                        n648 = Unbundle By Name(w1923) -> ("strings"=w1922:string[])
                        n649 = for {
                          N: w1921 -> [_]
                          tunnel: w1922 -> [w1933]
                          tunnel: w1920 -> [w1930]
                          shift-right: [w1935] -> w1918
                          shift-left: w1919 -> [w1935]
                          tunnel: w1917 -> [w1934]
                          shift-right: [w1931] -> w1914
                          shift-left: w1916 -> [w1928]
                          tunnel: w1915 -> [w1925]
                          i -> [w1927]
                          n650 = Add(x=w1927, y=w1930) -> (x+y=w1926:i32)
                          n651 = Index Array(array=w1935, index (row)=w1926, index (col)=w1934) -> (element=w1932:i32)
                          n652 = Replace Array Subset(array=w1928, new element=",", index (row)=w1926, index (col)=w1925) -> (w1929:string[][])
                          n653 = case shown="Default" w1932 {
                            selector: w1932 -> [_ w1948]
                            tunnel: w1933 -> [_ w1949]
                            tunnel: w1929 -> [w1936 w1937]
                            tunnel: w1925 -> [_ w1941]
                            tunnel: [w1936 w1939] -> w1931
                            tunnel: w1926 -> [_ w1938]
                            frame -1 {
                              # "no value"
                            }
                            frame Default {
                              w1944 = "\"" ("search string")
                              n654 = Index Array(array=w1949, index=w1948) -> (element=w1943:string)
                              n655 = Increment(x=w1941) -> (x+1=w1940:i32)
                              n656 = Search and Replace String(replace all?=TRUE ("replace all? (F)"), input string=w1943, search string=w1944, replace string="\"\"" ("replace string (\"\")")) -> (result string=w1947:string)  [unwired: 4 in, 3 out]
                              n657 = Concatenate Strings(w1944, w1947, w1944) -> (w1942:string)
                              n658 = Replace Array Subset(array=w1937, new element=w1942, index (row)=w1938, index (col)=w1940) -> (w1939:string[][])
                            }
                          }
                        }
                      }
                      frame "number" {
                        n659 = Unbundle By Name(w1960) -> ("values"=w1959:dbl[])
                        n660 = for {
                          N: w1958 -> [_]
                          tunnel: w1959 -> [w1971]
                          tunnel: w1957 -> [w1967]
                          shift-right: [w1973] -> w1955
                          shift-left: w1956 -> [w1973]
                          tunnel: w1954 -> [w1972]
                          shift-right: [w1969] -> w1951
                          shift-left: w1953 -> [w1966]
                          tunnel: w1952 -> [w1961]
                          tunnel: "%.;%#_14g" ("format string") -> [w1968]
                          i -> [w1964]
                          n661 = Add(x=w1964, y=w1967) -> (x+y=w1962:i32)
                          n662 = Index Array(array=w1973, index (row)=w1962, index (col)=w1972) -> (element=w1970:i32)
                          n663 = Replace Array Subset(array=w1966, new element=",", index (row)=w1962, index (col)=w1961) -> (w1965:string[][])
                          n664 = case shown="Default" w1970 {
                            selector: w1970 -> [_ w1984]
                            tunnel: w1971 -> [_ w1985]
                            tunnel: w1965 -> [w1974 w1975]
                            tunnel: w1961 -> [_ w1983]
                            tunnel: [w1974 w1981] -> w1969
                            tunnel: w1968 -> [_ w1977]
                            tunnel: w1962 -> [_ w1976]
                            frame -1 {
                              # "no value"
                            }
                            frame Default {
                              n665 = Index Array(array=w1985, index=w1984) -> (element=w1978:dbl)
                              n666 = Not A Number/Path/Refnum?(number/path/refnum=w1978) -> (NaN/Path/Refnum?=w1979:bool)
                              n667 = Increment(x=w1983) -> (x+1=w1982:i32)
                              n668 = case shown="False" w1979 {
                                tunnel: w1978 -> [w1988 _]
                                tunnel: [w1987 ""] -> w1980
                                tunnel: w1977 -> [w1986 _]
                                frame False {
                                n669 = Format Into String(format string=w1986, w1988) -> (resulting string=w1987:string)  [unwired: 2 in, 1 out]
                                }
                                frame True {
                                }
                              }
                              n670 = Replace Array Subset(array=w1975, new element=w1980, index (row)=w1976, index (col)=w1982) -> (w1981:string[][])
                            }
                          }
                        }
                      }
                    }
                  }
                  n671 = Concatenate Strings(w1874) -> (w1873:string)
                  n672 = Less Or Equal?(x=w1857, y=w1856) -> (x <= y?=w1858:bool)
                  n673 = Write to Binary File(file (use dialog)=w1871, data=w1873, 5:FALSE ("prepend array or string size? (T)")) -> (error out=w1872:errorcluster)  [unwired: 3 in, 2 out]
                }
                frame Error {
                }
              }
            }
            n674 = call "Library Log Error to Window.vi"("error in (no error)"=w1824) -> ()  [unwired: 13 in, 2 out]
            n675 = Close File(refnum=w1819) -> ()  [unwired: 1 in, 2 out]
          }
          frame #3 {
            n676 = call <vilib>:"Unset Busy.vi"() -> ()  [unwired: 11 in, 1 out]
          }
        }
      }
      frame "show string" {
        n677 = property on="log table" class="Tbl (strict)"() -> ("Key Focus"=w2005:bool, "Old Edit Position"=w2006:T18)  [unwired: 2 in, 2 out]
        n678 = case shown="True" w2005 {
          tunnel: w2006 -> [_ w2025]
          tunnel: w2004 -> [w2013 w2017]
          tunnel: [w2013 w2023] -> w2003
          tunnel: w2002 -> [w2012 w2015]
          tunnel: [w2012 w2014] -> w2001
          frame False {
          }
          frame True {
            n679 = Unbundle By Name(w2025) -> ("Column"=w2022:i32, "Row"=w2021:i32)
            n680 = property on="log table" class="Tbl (strict)"("Key Focus"=FALSE) -> ()  [unwired: 2 in, 2 out]
            n681 = Array Size(array=w2017) -> (size(s)=w2016:i32)
            n682 = Greater Or Equal To 0?(x=w2022) -> (x >= 0?=w2020:bool)
            n683 = Greater Or Equal To 0?(x=w2021) -> (x >= 0?=w2019:bool)
            n684 = And(x=w2020, y=w2019) -> (x .and. y?=w2018:bool)
            n685 = case shown="True" w2018 {
              tunnel: w2022 -> [_ w2034]
              tunnel: [w2027 w2033] -> w2023
              tunnel: w2021 -> [_ w2032]
              tunnel: w2017 -> [w2027 w2031]
              tunnel: w2016 -> [_ w2030]
              tunnel: w2015 -> [w2026 w2029]
              tunnel: [w2026 w2028] -> w2014
              frame False {
              }
              frame True {
                n686 = case shown="Default" w2030 {
                  tunnel: w2034 -> [_ w2040]
                  tunnel: w2031 -> [w2036 w2043]
                  tunnel: [w2036 w2042] -> w2033
                  tunnel: w2032 -> [_ w2041]
                  tunnel: w2029 -> [w2035 w2039]
                  tunnel: [w2035 w2038] -> w2028
                  frame 0 {
                  }
                  frame Default {
                    n687 = call "obj_DataLog Table Columns.vi"("method"=t_Datalog_Table_Columns_Methods."index", "index"=w2040) -> ("tag config"=w2045:T13)  [unwired: 8 in, 5 out]
                    n688 = Unbundle By Name(w2045) -> ("name"=w2037:string, "value"=w2044:T12)
                    n689 = case shown="\"string\"" w2044 {
                      tunnel: w2043 -> [w2048 w2058]
                      tunnel: [w2048 w2058] -> w2042
                      tunnel: w2041 -> [_ w2059]
                      tunnel: w2040 -> [_ w2060]
                      tunnel: w2039 -> [w2047 w2057]
                      tunnel: [w2047 w2057] -> w2038
                      tunnel: w2037 -> [_ w2051]
                      frame "number" {
                      }
                      frame "string" {
                        n690 = Index Array(array=w2057, index (row)=w2059, index (col)=w2060) -> (element=w2052:i32)
                        n691 = Index Array(array=w2058, index=w2060) -> (element=w2054:T11)
                        n692 = Unbundle By Name(w2054) -> ("strings"=w2053:string[])
                        n693 = Concatenate Strings("Value of Tag " ("string"), w2051) -> (w2049:string)
                        n694 = Index Array(array=w2053, index=w2052) -> (element=w2055:string)
                        n695 = Empty String/Path?(string/path=w2055) -> (empty?=w2056:bool)
                        n696 = case shown="False" w2056 {
                          tunnel: w2055 -> [w2062 _]
                          tunnel: w2049 -> [w2061 _]
                          frame False {
                            n697 = call "ui_DataLog Show Big String.vi"("title"=w2061, "string to show"=w2062) -> ()  [unwired: 14 in]
                          }
                          frame True {
                          }
                        }
                      }
                    }
                  }
                }
              }
            }
          }
        }
      }
      frame "count rows" {
        # "rows included in filtered\ndataset + break skips"
        # "Instead of throwing away data, we use an array of indices to mark the rows of the filtered dataset. These indices are specified for each row in the full dataset. When the index is negative, that row is excluded from the filtered dataset. When the index is positive or zero, that row of the full dataset is included at the row of the reduced dataset specified by the index. The presence of excluded rows is marked in the filtered dataset by skipping a row."
        n698 = Array Size(array=w2076) -> (size(s)=w2068:i32)
        n699 = for {
          N: w2068 -> [_]
          shift-right: [w2089] -> w2074
          shift-left: w2076 -> [w2095]
          shift-right: [w2092] -> w2071
          shift-left: 0 -> [w2093]
          shift-right: [w2091] -> w2072
          shift-left: FALSE -> [w2090]
          shift-right: [w2087] -> w2067
          shift-left: 0 -> [w2088]
          i -> [w2094]
          # "include count"
          # "row index"
          n700 = Index Array(array=w2095, index=w2094) -> (element=w2097:i32)
          n701 = Greater Or Equal To 0?(x=w2097) -> (x >= 0?=w2096:bool)
          n702 = case "included?" shown="True" w2096 {
            selector: w2096 -> [w2103 w2110]
            tunnel: w2095 -> [w2099 w2114]
            tunnel: w2094 -> [_ w2113]
            tunnel: w2093 -> [w2102 w2112]
            tunnel: [w2101 w2111] -> w2092
            tunnel: [w2103 w2110] -> w2091
            tunnel: w2090 -> [w2100 _]
            tunnel: [w2099 w2109] -> w2089
            tunnel: w2088 -> [w2098 w2108]
            tunnel: [w2098 w2107] -> w2087
            frame False {
              # "skip a display row on encountering\nthe first excluded row of data"
              n703 = case shown="True" w2100 {
                tunnel: w2102 -> [w2104 w2106]
                tunnel: [w2104 w2105] -> w2101
                frame False {
                }
                frame True {
                  n704 = Increment(x=w2106) -> (x+1=w2105:i32)
                }
              }
            }
            frame True {
              n705 = Replace Array Subset(array=w2114, new element=w2112, index=w2113) -> (w2109:i32[])
              n706 = Increment(x=w2108) -> (x+1=w2107:i32)
              n707 = Increment(x=w2112) -> (x+1=w2111:i32)
            }
          }
        }
        "included" <- w2067
        n708 = case shown="False" w2072 {
          tunnel: w2071 -> [w2085 w2086]
          tunnel: [w2082 w2086] -> w2070
          frame False {
            # "revert superfluous\nskip at end"
            n709 = Decrement(x=w2085) -> (x-1=w2084:i32)
            n710 = Max & Min(x=w2084, y=0) -> (max(x,y)=w2082:i32)  [unwired: 1 out]
          }
          frame True {
          }
        }
        n711 = Subtract(x=w2068, y=w2067) -> (x-y=→"excluded":i32)
      }
      frame "time headers" {
        n712 = Initialize Array("", w2117) -> (w2125:string[])
        n713 = global read "glb_Library Configuration Globals.vi" "time format"() -> (w2129:string)
        n714 = Initialize Array(-1, w2117) -> (w2118:i32[])
        n715 = for {
          tunnel: w2129 -> [w2140]
          shift-right: [w2136] -> w2124
          shift-left: w2125 -> [w2137]
          tunnel: w2122 -> [w2139] mode=indexing
          tunnel: w2123 -> [w2133] mode=indexing
          shift-right: [w2134] -> w2116
          shift-left: w2118 -> [w2135]
          i -> [w2132]
          n716 = Greater Or Equal To 0?(x=w2133) -> (x >= 0?=w2138:bool)
          n717 = case shown="True" w2138 {
            tunnel: w2140 -> [_ w2152]
            tunnel: w2139 -> [_ w2144]
            tunnel: w2137 -> [w2142 w2149]
            tunnel: w2133 -> [_ w2151]
            tunnel: [w2142 w2148] -> w2136
            tunnel: w2135 -> [w2141 w2147]
            tunnel: [w2141 w2146] -> w2134
            tunnel: w2133 -> [_ w2145]
            tunnel: w2132 -> [_ w2143]
            frame False {
            }
            frame True {
              n718 = Format Date/Time String(time format string (%c)=w2152, seconds (now)=w2144) -> (date/time string=w2150:string)  [unwired: 1 in]
              n719 = Replace Array Subset(array=w2149, new element=w2150, index=w2151) -> (w2148:string[])
              n720 = Replace Array Subset(array=w2147, new element=w2143, index=w2145) -> (w2146:i32[])
            }
          }
        }
        n721 = property on="log table" class="Tbl (strict)"("Row Header Strings[]"=w2124, "Value"=string[][] [] ("log table")) -> ()  [unwired: 2 in, 2 out]
      }
      frame "tabulate" {
        n722 = stacked-sequence {
          tunnel: [_ w2181 _] -> w2165
          tunnel: w2164 -> [_ w2180 _]
          tunnel: w2163 -> [_ _ w2395]
          tunnel: [_ _ w2395] -> w2162
          tunnel: w2161 -> [_ w2178 _]
          tunnel: [_ w2179 _] -> w2160
          tunnel: w2159 -> [_ w2170 _]
          tunnel: [_ w2170 _] -> w2158
          tunnel: w2156 -> [_ w2174 _]
          tunnel: [_ w2173 _] -> w2157
          tunnel: [_ w2168 _] -> w2155
          frame #0 {
            n723 = call <vilib>:"Set Busy.vi"() -> ()  [unwired: 10 in, 2 out]
          }
          frame #1 {
            n724 = Array Size(array=w2180) -> (size(s)=w2171:i32)
            n725 = Initialize Array(-1, w2170, w2171) -> (w2172:i32[][])
            n726 = Initialize Array("", w2170, w2171) -> (w2177:string[][])
            n727 = for {
              N: w2171 -> [_]
              shift-right: [w2192] -> w2181
              shift-left: w2180 -> [w2196]
              shift-right: [w2190] -> w2179
              shift-left: w2178 -> [w2191]
              shift-right: [w2186] -> w2175
              shift-left: w2177 -> [w2187]
              shift-right: [w2188] -> w2173
              shift-left: w2174 -> [w2189]
              shift-right: [w2182] -> w2168
              shift-left: w2172 -> [w2183]
              i -> [w2195]
              n728 = call "obj_DataLog Table Columns.vi"("method"=t_Datalog_Table_Columns_Methods."index", "index"=w2195) -> ("tag config"=w2185:T13, "mode"=w2193:T21)  [unwired: 8 in, 4 out]
              n729 = Unbundle By Name(w2185) -> ("value"=w2184:T12)
              n730 = case shown="\"at\"" w2193 {
                tunnel: w2196 -> [w2206 w2283]
                tunnel: w2195 -> [w2200 w2279]
                tunnel: w2185 -> [w2202 w2275]
                tunnel: [w2206 w2271] -> w2192
                tunnel: w2191 -> [w2205 w2282]
                tunnel: [w2205 w2281] -> w2190
                tunnel: w2189 -> [w2203 w2278]
                tunnel: [w2203 w2277] -> w2188
                tunnel: w2187 -> [w2204 w2280]
                tunnel: [w2201 w2276] -> w2186
                tunnel: w2184 -> [w2199 w2274]
                tunnel: w2183 -> [w2198 w2273]
                tunnel: [w2197 w2272] -> w2182
                frame "interpolate", "at+interpolate" {
                  n731 = Index Array(array=w2206, index=w2200) -> (element=w2207:T11)
                  n732 = case shown="\"number\"" w2199 {
                    tunnel: w2207 -> [w2216 w2247]
                    tunnel: w2204 -> [w2215 w2246]
                    tunnel: w2203 -> [w2214 w2245]
                    tunnel: w2202 -> [w2212 _]
                    tunnel: [w2211 w2243] -> w2201
                    tunnel: w2200 -> [w2210 w2242]
                    tunnel: w2198 -> [w2209 w2240]
                    tunnel: [w2208 w2239] -> w2197
                    frame "number" {
                      n733 = Unbundle By Name(w2216) -> ("values"=w2213:dbl[])
                      n734 = for {
                        shift-right: [w2222] -> w2211
                        shift-left: w2215 -> [w2223]
                        tunnel: w2214 -> [w2221] mode=indexing
                        tunnel: w2213 -> [w2226] mode=indexing
                        tunnel: w2212 -> [w2224]
                        tunnel: w2210 -> [w2220]
                        shift-right: [w2218] -> w2208
                        shift-left: w2209 -> [w2219]
                        i -> [w2217]
                        n735 = Greater Or Equal To 0?(x=w2221) -> (x >= 0?=w2225:bool)
                        n736 = case shown="True" w2225 {
                          tunnel: w2226 -> [_ w2238]
                          tunnel: w2224 -> [_ w2237]
                          tunnel: w2221 -> [_ w2231]
                          tunnel: w2223 -> [w2228 w2236]
                          tunnel: [w2228 w2235] -> w2222
                          tunnel: w2220 -> [_ w2230]
                          tunnel: w2219 -> [w2227 w2233]
                          tunnel: [w2227 w2232] -> w2218
                          tunnel: w2217 -> [_ w2229]
                          frame False {
                          }
                          frame True {
                            n737 = call "DataLog Format Point Value.vi"("value"=w2238, "tag config"=w2237) -> ("formatted value"=w2234:string)  [unwired: 13 in]
                            n738 = Replace Array Subset(array=w2233, new element=w2229, index (row)=w2231, index (col)=w2230) -> (w2232:i32[][])
                            n739 = Replace Array Subset(array=w2236, new element=w2234, index (row)=w2231, index (col)=w2230) -> (w2235:string[][])
                          }
                        }
                      }
                    }
                    frame "string" {
                      n740 = Unbundle By Name(w2247) -> ("strings"=w2241:string[], "values"=w2244:dbl[])
                      n741 = for {
                        shift-right: [w2254] -> w2243
                        shift-left: w2246 -> [w2255]
                        tunnel: w2245 -> [w2253] mode=indexing
                        tunnel: w2244 -> [w2250] mode=indexing
                        tunnel: w2242 -> [w2252]
                        tunnel: w2241 -> [w2251]
                        shift-right: [w2248] -> w2239
                        shift-left: w2240 -> [w2249]
                        n742 = Greater Or Equal To 0?(x=w2253) -> (x >= 0?=w2256:bool)
                        n743 = case shown="True" w2256 {
                          tunnel: w2253 -> [_ w2261]
                          tunnel: w2255 -> [w2258 w2270]
                          tunnel: [w2258 w2269] -> w2254
                          tunnel: w2252 -> [_ w2260]
                          tunnel: w2251 -> [_ w2265]
                          tunnel: w2250 -> [_ w2266]
                          tunnel: w2249 -> [w2257 w2263]
                          tunnel: [w2257 w2262] -> w2248
                          frame False {
                          }
                          frame True {
                            n744 = To Long Integer(number=w2266) -> (32bit integer=w2259:i32)
                            n745 = Index Array(array=w2265, index=w2259) -> (element=w2264:string)
                            n746 = String Subset(string=w2264, length (rest)=100 ("length (rest)")) -> (substring=w2267:string)  [unwired: 1 in]
                            n747 = Replace Array Subset(array=w2263, new element=w2259, index (row)=w2261, index (col)=w2260) -> (w2262:i32[][])
                            n748 = Replace Array Subset(array=w2270, new element=w2267, index (row)=w2261, index (col)=w2260) -> (w2269:string[][])
                          }
                        }
                      }
                    }
                  }
                }
                frame "at" {
                  n749 = case shown="\"string\"" w2274 {
                    tunnel: w2283 -> [w2284 w2339]
                    tunnel: w2282 -> [w2297 w2352]
                    tunnel: [w2296 w2351] -> w2281
                    tunnel: w2280 -> [w2294 w2348]
                    tunnel: w2279 -> [w2293 w2347]
                    tunnel: w2278 -> [w2292 w2346]
                    tunnel: [w2291 w2345] -> w2277
                    tunnel: [w2290 w2344] -> w2276
                    tunnel: w2275 -> [w2289 _]
                    tunnel: w2273 -> [w2286 w2341]
                    tunnel: [w2285 w2340] -> w2272
                    tunnel: [w2284 w2339] -> w2271
                    frame "number" {
                      n750 = Index Array(array=w2284, index=w2293) -> (element=w2298:T11)
                      n751 = Unbundle By Name(w2298) -> ("values"=w2288:dbl[], "times"=w2287:dbl[])
                      n752 = for {
                        shift-right: [w2317] -> w2296
                        shift-left: w2297 -> [w2318]
                        shift-right: [w2315] -> _
                        shift-left: 0 -> [w2316]
                        shift-right: [w2308] -> w2290
                        shift-left: w2294 -> [w2313]
                        tunnel: w2293 -> [w2304]
                        shift-right: [w2312] -> w2291
                        shift-left: w2292 -> [w2312]
                        tunnel: w2289 -> [w2305]
                        tunnel: w2288 -> [w2303] mode=indexing
                        tunnel: w2287 -> [w2302] mode=indexing
                        shift-right: [w2300] -> w2285
                        shift-left: w2286 -> [w2301]
                        i -> [w2299]
                        n753 = Search 1D Array(1D array=w2318, element=w2302, start index (0)=w2316) -> (index of element=w2314:i32)
                        n754 = Greater Or Equal To 0?(x=w2314) -> (x >= 0?=w2319:bool)
                        n755 = case shown="False" w2319 {
                          tunnel: w2318 -> [w2333 w2338]
                          tunnel: [w2333 w2338] -> w2317
                          tunnel: w2316 -> [w2334 _]
                          tunnel: [w2334 w2336] -> w2315
                          tunnel: w2314 -> [_ w2337]
                          tunnel: [w2335 w2337] -> w2311
                          tunnel: w2302 -> [w2332 _]
                          frame False {
                            n756 = Search 1D Array(1D array=w2333, element=w2332) -> (index of element=w2335:i32)  [unwired: 1 in]
                          }
                          frame True {
                            n757 = Increment(x=w2337) -> (x+1=w2336:i32)
                          }
                        }
                        n758 = Index Array(array=w2312, index=w2311) -> (element=w2307:i32)
                        n759 = Greater Or Equal To 0?(x=w2311) -> (x >= 0?=w2309:bool)
                        n760 = Greater Or Equal To 0?(x=w2307) -> (x >= 0?=w2310:bool)
                        n761 = And(x=w2310, y=w2309) -> (x .and. y?=w2306:bool)
                        n762 = case shown="True" w2306 {
                          tunnel: w2313 -> [w2321 w2331]
                          tunnel: [w2321 w2330] -> w2308
                          tunnel: w2307 -> [_ w2324]
                          tunnel: w2303 -> [_ w2328]
                          tunnel: w2305 -> [_ w2329]
                          tunnel: w2304 -> [_ w2323]
                          tunnel: w2301 -> [w2320 w2326]
                          tunnel: [w2320 w2325] -> w2300
                          tunnel: w2299 -> [_ w2322]
                          frame False {
                          }
                          frame True {
                            n763 = call "DataLog Format Point Value.vi"("value"=w2328, "tag config"=w2329) -> ("formatted value"=w2327:string)  [unwired: 13 in]
                            n764 = Replace Array Subset(array=w2326, new element=w2322, index (row)=w2324, index (col)=w2323) -> (w2325:i32[][])
                            n765 = Replace Array Subset(array=w2331, new element=w2327, index (row)=w2324, index (col)=w2323) -> (w2330:string[][])
                          }
                        }
                      }
                    }
                    frame "string" {
                      n766 = Index Array(array=w2339, index=w2347) -> (element=w2353:T11)
                      n767 = Unbundle By Name(w2353) -> ("strings"=w2342:string[], "values"=w2343:dbl[], "times"=w2350:dbl[])
                      n768 = for {
                        shift-right: [w2372] -> w2351
                        shift-left: w2352 -> [w2373]
                        tunnel: w2350 -> [w2358] mode=indexing
                        shift-right: [w2370] -> _
                        shift-left: 0 -> [w2371]
                        shift-right: [w2363] -> w2344
                        shift-left: w2348 -> [w2368]
                        tunnel: w2347 -> [w2360]
                        shift-right: [w2367] -> w2345
                        shift-left: w2346 -> [w2367]
                        tunnel: w2343 -> [w2359] mode=indexing
                        tunnel: w2342 -> [w2356]
                        shift-right: [w2354] -> w2340
                        shift-left: w2341 -> [w2355]
                        n769 = To Long Integer(number=w2359) -> (32bit integer=w2357:i32)
                        n770 = Search 1D Array(1D array=w2373, element=w2358, start index (0)=w2371) -> (index of element=w2369:i32)
                        n771 = Greater Or Equal To 0?(x=w2369) -> (x >= 0?=w2374:bool)
                        n772 = case shown="False" w2374 {
                          tunnel: w2373 -> [w2389 w2394]
                          tunnel: [w2389 w2394] -> w2372
                          tunnel: w2371 -> [w2390 _]
                          tunnel: [w2390 w2392] -> w2370
                          tunnel: w2369 -> [_ w2393]
                          tunnel: [w2391 w2393] -> w2366
                          tunnel: w2358 -> [w2388 _]
                          frame False {
                            n773 = Search 1D Array(1D array=w2389, element=w2388) -> (index of element=w2391:i32)  [unwired: 1 in]
                          }
                          frame True {
                            n774 = Increment(x=w2393) -> (x+1=w2392:i32)
                          }
                        }
                        n775 = Index Array(array=w2367, index=w2366) -> (element=w2362:i32)
                        n776 = Greater Or Equal To 0?(x=w2366) -> (x >= 0?=w2364:bool)
                        n777 = Greater Or Equal To 0?(x=w2362) -> (x >= 0?=w2365:bool)
                        n778 = And(x=w2365, y=w2364) -> (x .and. y?=w2361:bool)
                        n779 = case shown="True" w2361 {
                          tunnel: w2368 -> [w2376 w2387]
                          tunnel: [w2376 w2386] -> w2363
                          tunnel: w2362 -> [_ w2379]
                          tunnel: w2357 -> [_ w2377]
                          tunnel: w2360 -> [_ w2378]
                          tunnel: w2356 -> [_ w2383]
                          tunnel: w2355 -> [w2375 w2381]
                          tunnel: [w2375 w2380] -> w2354
                          frame False {
                          }
                          frame True {
                            n780 = Index Array(array=w2383, index=w2377) -> (element=w2382:string)
                            n781 = String Subset(string=w2382, length (rest)=100 ("length (rest)")) -> (substring=w2384:string)  [unwired: 1 in]
                            n782 = Replace Array Subset(array=w2381, new element=w2377, index (row)=w2379, index (col)=w2378) -> (w2380:i32[][])
                            n783 = Replace Array Subset(array=w2387, new element=w2384, index (row)=w2379, index (col)=w2378) -> (w2386:string[][])
                          }
                        }
                      }
                    }
                  }
                }
              }
            }
            "log table" <- w2175
          }
          frame #2 {
            n784 = call <vilib>:"Unset Busy.vi"() -> ()  [unwired: 11 in, 1 out]
          }
        }
      }
      frame "abort query" {
        # "ignore errors:\nthis serves to free server-side\nmemory but is not essential"
        n785 = local read "query"() -> (w2401:T3)
        n786 = call "obj_ClientSrv Client Access State.vi"() -> ("certificate"=w2403:string, "error out"=w2404:errorcluster)  [unwired: 14 in]
        n787 = call-by-ref "?"(reference=w2401, error in=w2404, "method"=t_DataLog_Query_Served_Methods."clear", "certificate"=w2403) -> ()  [unwired: 8 in, 8 out]
        n788 = Build Array (concatenate)(t_DataLog_Log_Table_States."clear query" ("states"), w2410) -> (w2408:T6[])
      }
      frame "clear query" {
        n789 = Reshape Array(w2436, 0 ("dimension size")) -> (w2434:T20)
        n790 = Reshape Array(w2431, 0 ("dimension size")) -> (w2430:dbl[])
        n791 = Reshape Array(w2415, 0 ("dimension size")) -> (w2414:i32[])
        n792 = local write "included"(0 ("dimension size")) -> ()
        n793 = local write "excluded"(0 ("dimension size")) -> ()
        n794 = call "obj_DataLog Table Columns.vi"("method"=t_Datalog_Table_Columns_Methods."update") -> ()  [unwired: 9 in, 6 out]
        n795 = Reshape Array(w2426, 0 ("dimension size")) -> (w2425:i32[])
        n796 = Reshape Array(w2419, 0 ("dimension size"), 0 ("dimension size")) -> (w2418:i32[][])
        n797 = Build Array (concatenate)(t_DataLog_Log_Table_States."ablement" ("states"), w2435) -> (w2428:T6[])
      }
      frame "clear all" {
        w2471 = string[] [] ("Row Headers[]")
        n798 = local write "included"(0 ("dimension size")) -> ()
        n799 = local write "excluded"(0 ("dimension size")) -> ()
        n800 = control-ref of="log table"() -> (w2463:refnum<vi>)
        n801 = local read "database infos"() -> (w2462:T4)
        n802 = call "obj_DataLog Table Columns.vi"("method"=t_Datalog_Table_Columns_Methods."clear", "database"=w2464, "database infos"=w2462, "table ref"=w2463) -> ()  [unwired: 6 in, 6 out]
        n803 = Reshape Array(w2458, 0 ("dimension size")) -> (w2457:dbl[])
        n804 = property on="log table" class="Tbl (strict)"("Row Header Strings[]"=w2471, "Column Header Strings[]"=w2471, "Value"=string[][] [] ("log table"), "Active Cell:Active Cell"=cluster{"Column":i32, "Row":i32} {"Column"=-2, "Row"=-2} ("Active Cell"), "Active Cell:Cell Background Color"=u32 15790320, "Active Cell:Cell FG Color"=u32 0, "Active Cell:Cell Size:Width"=u32 68 ("Cell Size:Width"), "Active Cell:Active Cell"=cluster{"Column":i32, "Row":i32} {"Column"=0, "Row"=-1} ("Active Cell"), "Active Cell:Cell Size:Width"=u32 130 ("Cell Size:Width")) -> ()  [unwired: 2 in, 2 out]
        n805 = Reshape Array(w2451, 0 ("dimension size")) -> (w2450:i32[])
        n806 = Reshape Array(w2441, 0 ("dimension size")) -> (w2440:i32[])
        n807 = Reshape Array(w2445, 0 ("dimension size"), 0 ("dimension size")) -> (w2444:i32[][])
        n808 = Build Array (concatenate)(t_DataLog_Log_Table_States."ablement" ("states"), w2473) -> (w2453:T6[])
        n809 = Initialize Array(T11 {"times"=[], "values"=[], "strings"=[]}, 0 ("dimension size")) -> (w2461:T20)
      }
      frame "set database" {
        n810 = property on="database" class="Ring (strict)"() -> ("Strings []"=w2485:string[])  [unwired: 2 in, 2 out]
        n811 = Index Array(array=w2485, index="database") -> (element=w2486:string)
        n812 = Empty String/Path?(string/path=w2486) -> (empty?=w2487:bool)
        n813 = case shown="True" w2487 {
          tunnel: w2485 -> [_ w2493]
          tunnel: w2486 -> [w2490 _]
          tunnel: [w2490 w2492] -> w2484
          frame False {
          }
          frame True {
            w2491 = 0 ("index")
            n814 = Index Array(array=w2493, index=w2491) -> (element=w2492:string)
            n815 = local write "database"(w2491) -> ()
          }
        }
        n816 = Build Array (concatenate)(t_DataLog_Log_Table_States."clear all" ("states"), w2489) -> (w2483:T6[])
      }
      frame "deselect" {
        n817 = Greater Or Equal To 0?(x=w2500) -> (x >= 0?=w2499:bool)
        n818 = case shown="True" w2499 {
          tunnel: w2500 -> [_ w2509]
          frame False {
          }
          frame True {
            n819 = Bundle("Row"=-1, "dimension size"=w2509) -> (w2508:cluster{"Row":i32, "dimension size":i32})  [unwired: 1 in]
            n820 = property on="log table" class="Tbl (strict)"("Active Cell:Active Cell"=w2508, "Active Cell:Cell Background Color"=u32 15790320, "Active Cell:Cell FG Color"=u32 0) -> ()  [unwired: 2 in, 2 out]
          }
        }
        n821 = Build Array (concatenate)(t_DataLog_Log_Table_States."ablement" ("states"), w2505) -> (w2502:T6[])
      }
      frame "ablement" {
        w2534 = u8 0 items=["enabled", "disabled", "grayed"] ("disabled state")
        w2516 = u8 2 items=["enabled", "disabled", "grayed"] ("disabled state")
        n822 = local read "begin time"() -> (w2574:timestamp)
        n823 = local read "end time"() -> (w2575:timestamp)
        n824 = case shown="Default" "comparison" {
          tunnel: [w2582 w2583] -> w2519
          frame "all", "==NaN", "~=NaN" {
            w2582 = u8 2 items=["enabled", "disabled", "grayed"] ("disabled state")
          }
          frame Default {
            w2583 = u8 0 items=["enabled", "disabled", "grayed"] ("disabled state")
          }
        }
        n825 = call "obj_DataLog Table Columns.vi"("method"=t_Datalog_Table_Columns_Methods."ats?") -> ("flag"=w2545:bool)  [unwired: 9 in, 5 out]
        n826 = call "obj_DataLog Table Columns.vi"("method"=t_Datalog_Table_Columns_Methods."index", "index"=w2542) -> ("tag config"=w2541:T13)  [unwired: 8 in, 5 out]
        n827 = To Double Precision Float(number=w2575) -> (double precision float=w2569:dbl)
        n828 = To Double Precision Float(number=w2574) -> (double precision float=w2568:dbl)
        n829 = Unbundle By Name(w2541) -> ("value"=w2538:T12)
        n830 = Less?(x=w2568, y=w2569) -> (x < y?=w2570:bool)
        n831 = call "obj_DataLog Table Columns.vi"("method"=t_Datalog_Table_Columns_Methods."#columns") -> ("#columns"=w2561:i32)  [unwired: 9 in, 5 out]
        n832 = call "obj_DataLog Table Columns.vi"("method"=t_Datalog_Table_Columns_Methods."interpolatable?", "index"=w2542) -> ("flag"=w2557:bool)  [unwired: 8 in, 5 out]
        n833 = Or(x="enable/disable", y=w2545) -> (x .or. y?=w2544:bool)
        n834 = Compound Arithmetic op=OR("earliest", "latest", w2570) -> (w2573:bool)
        n835 = Array Size(array=w2536) -> (size(s)=w2565:i32)
        n836 = And(x=w2544, y=w2573) -> (x .and. y?=w2547:bool)
        n837 = Equal To 0?(x=w2565) -> (x = 0?=w2529:bool)
        n838 = Greater?(x=w2561, y=1) -> (0:w2524:bool)
        n839 = call "obj_DataLog Table Columns.vi"("method"=t_Datalog_Table_Columns_Methods."#number") -> ("#columns"=w2515:i32)  [unwired: 9 in, 5 out]
        n840 = Greater Than 0?(x=w2561) -> (x > 0?=w2563:bool)
        n841 = Equal?(x=t_DataLog_Value_Types."number" ("value"), y=w2538) -> (x = y?=w2533:bool)
        n842 = case shown="\"all\", \"UNDEFINED\", \"DEFINED\"" "match" {
          tunnel: [w2580 w2581] -> w2535
          frame "all", "UNDEFINED", "DEFINED" {
            w2580 = u8 2 items=["enabled", "disabled", "grayed"] ("disabled state")
          }
          frame Default {
            w2581 = u8 0 items=["enabled", "disabled", "grayed"] ("disabled state")
          }
        }
        n843 = Greater Than 0?(x=w2515) -> (x > 0?=w2514:bool)
        n844 = Greater?(x=w2515, y=1) -> (0:w2518:bool)
        n845 = Greater Or Equal To 0?(x=w2542) -> (x >= 0?=w2550:bool)
        n846 = Select(t=w2516, s="earliest", f=w2534) -> (s? t:f=w2577:u8)
        n847 = Select(t=w2516, s="latest", f=w2534) -> (s? t:f=w2576:u8)
        n848 = Select(t=w2516, s=w2529, f=w2534) -> (s? t:f=w2517:u8)
        n849 = Select(t=w2534, s=w2529, f=w2516) -> (s? t:f=w2556:u8)
        n850 = Select(t=w2534, s="enable/disable", f=w2516) -> (s? t:f=w2554:u8)
        n851 = Select(t=w2534, s=w2550, f=w2516) -> (s? t:f=w2537:u8)
        n852 = Select(t=w2534, s=w2547, f=w2516) -> (s? t:f=w2523:u8)
        n853 = Select(t=w2519, s=w2533, f=w2516) -> (s? t:f=w2532:u8)
        n854 = Select(t=w2516, s=w2533, f=w2535) -> (s? t:f=w2530:u8)
        n855 = Select(t=w2516, s=w2529, f=w2537) -> (s? t:f=w2549:u8)
        n856 = Select(t=w2516, s=w2529, f=w2532) -> (s? t:f=w2531:u8)
        n857 = Select(t=w2516, s=w2529, f=w2530) -> (s? t:f=w2528:u8)
        n858 = Select(t=w2517, s=w2514, f=w2516) -> (s? t:f=w2513:u8)
        n859 = Select(t=w2517, s=w2518, f=w2516) -> (s? t:f=w2522:u8)
        n860 = Select(t=w2556, s=w2550, f=w2516) -> (s? t:f=w2566:u8)
        n861 = Select(t=w2556, s=w2557, f=w2516) -> (s? t:f=w2555:u8)
        n862 = Select(t=w2556, s=w2563, f=w2516) -> (s? t:f=w2562:u8)
        n863 = Select(t=w2556, s=w2524, f=w2516) -> (s? t:f=w2559:u8)
        n864 = stacked-sequence {
          tunnel: w2577 -> [_ w2585 _ _ _ _ _ _ _ _ _ _ _ _ _ _ _ _ _ _ _ _ _ _ _]
          tunnel: w2576 -> [_ _ _ w2587 _ _ _ _ _ _ _ _ _ _ _ _ _ _ _ _ _ _ _ _ _]
          tunnel: w2523 -> [_ _ _ _ w2588 _ _ _ _ _ _ _ _ _ _ _ _ _ _ _ _ _ _ _ _]
          tunnel: w2566 -> [_ _ _ _ _ _ _ _ _ _ _ _ _ _ _ w2599 w2600 _ _ _ _ _ _ _ _]
          tunnel: w2556 -> [_ _ _ _ _ _ _ _ _ _ _ _ _ _ _ _ _ w2601 w2602 w2603 _ _ _ _ _]
          tunnel: w2562 -> [_ _ _ _ _ _ _ _ _ _ _ _ _ _ _ _ _ _ _ _ _ w2605 _ _ _]
          tunnel: w2559 -> [_ _ _ _ _ _ _ _ _ _ _ _ _ _ _ _ _ _ _ _ _ _ w2606 w2607 _]
          tunnel: w2555 -> [_ _ _ _ _ _ _ _ _ _ _ _ _ _ _ _ _ _ _ _ w2604 _ _ _ _]
          tunnel: w2554 -> [w2584 _ _ _ _ _ _ _ _ _ _ _ _ _ _ _ _ _ _ _ _ _ _ _ _]
          tunnel: w2517 -> [_ _ _ _ _ _ w2590 w2591 w2592 w2593 w2594 w2595 _ _ _ _ _ _ _ _ _ _ _ _ _]
          tunnel: w2549 -> [_ _ _ _ _ _ _ _ _ _ _ _ w2596 w2597 _ _ _ _ _ _ _ _ _ _ _]
          tunnel: w2531 -> [_ _ _ _ _ _ _ _ _ _ _ _ _ _ w2598 _ _ _ _ _ _ _ _ _ _]
          tunnel: w2528 -> [_ _ _ _ _ _ _ _ _ _ _ _ _ _ _ _ _ _ _ _ _ _ _ _ w2608]
          tunnel: w2522 -> [_ _ _ _ _ w2589 _ _ _ _ _ _ _ _ _ _ _ _ _ _ _ _ _ _ _]
          tunnel: w2513 -> [_ _ w2586 _ _ _ _ _ _ _ _ _ _ _ _ _ _ _ _ _ _ _ _ _ _]
          frame #0 {
            n865 = property on="time step" class="DigNum (strict)"("Disabled"=w2584) -> ()  [unwired: 2 in, 2 out]
          }
          frame #1 {
            n866 = property on="begin time" class="AbsTime (strict)"("Disabled"=w2585) -> ()  [unwired: 2 in, 2 out]
          }
          frame #2 {
            n867 = property on="time graph" class="Bool"("Disabled"=w2586) -> ()  [unwired: 2 in, 2 out]
          }
          frame #3 {
            n868 = property on="end time" class="AbsTime (strict)"("Disabled"=w2587) -> ()  [unwired: 2 in, 2 out]
          }
          frame #4 {
            n869 = property on="retrieve" class="Bool"("Disabled"=w2588) -> ()  [unwired: 2 in, 2 out]
          }
          frame #5 {
            n870 = property on="xy graph" class="Bool"("Disabled"=w2589) -> ()  [unwired: 2 in, 2 out]
          }
          frame #6 {
            n871 = property on="export" class="Bool"("Disabled"=w2590) -> ()  [unwired: 2 in, 2 out]
          }
          frame #7 {
            n872 = property on="clear" class="Bool"("Disabled"=w2591) -> ()  [unwired: 2 in, 2 out]
          }
          frame #8 {
            n873 = property on="excluded" class="DigNum (strict)"("Disabled"=w2592) -> ()  [unwired: 2 in, 2 out]
          }
          frame #9 {
            n874 = property on="included" class="DigNum (strict)"("Disabled"=w2593) -> ()  [unwired: 2 in, 2 out]
          }
          frame #10 {
            n875 = property on="comparison" class="Enum (strict)"("Disabled"=w2594) -> ()  [unwired: 2 in, 2 out]
          }
          frame #11 {
            n876 = property on="match" class="Enum (strict)"("Disabled"=w2595) -> ()  [unwired: 2 in, 2 out]
          }
          frame #12 {
            n877 = property on="exclude" class="Bool"("Disabled"=w2596) -> ()  [unwired: 2 in, 2 out]
          }
          frame #13 {
            n878 = property on="include" class="Bool"("Disabled"=w2597) -> ()  [unwired: 2 in, 2 out]
          }
          frame #14 {
            n879 = property on="number" class="DigNum (strict)"("Disabled"=w2598) -> ()  [unwired: 2 in, 2 out]
          }
          frame #15 {
            n880 = property on="remove" class="Bool"("Disabled"=w2599) -> ()  [unwired: 2 in, 2 out]
          }
          frame #16 {
            n881 = property on="insert" class="Bool"("Disabled"=w2600) -> ()  [unwired: 2 in, 2 out]
          }
          frame #17 {
            n882 = property on="add" class="Bool"("Disabled"=w2601) -> ()  [unwired: 2 in, 2 out]
          }
          frame #18 {
            n883 = property on="multi" class="Bool"("Disabled"=w2602) -> ()  [unwired: 2 in, 2 out]
          }
          frame #19 {
            n884 = property on="subset" class="Bool"("Disabled"=w2603) -> ()  [unwired: 2 in, 2 out]
          }
          frame #20 {
            n885 = property on="mode" class="Bool"("Disabled"=w2604) -> ()  [unwired: 2 in, 2 out]
          }
          frame #21 {
            n886 = property on="remove all" class="Bool"("Disabled"=w2605) -> ()  [unwired: 2 in, 2 out]
          }
          frame #22 {
            n887 = property on="reorder" class="Bool"("Disabled"=w2606) -> ()  [unwired: 2 in, 2 out]
          }
          frame #23 {
            n888 = property on="sort" class="Bool"("Disabled"=w2607) -> ()  [unwired: 2 in, 2 out]
          }
          frame #24 {
            n889 = property on="string" class="Str"("Disabled"=w2608) -> ()  [unwired: 2 in, 2 out]
          }
        }
      }
      frame "resize" {
        n890 = flat-sequence {
          frame #0 {
            n891 = property class="VI"() -> ("Front Panel"=w2619:refnum<vi>)  [unwired: 2 in, 2 out]
            n892 = property class="Pnl"(reference=w2619, "Defer Panel Updates"=TRUE) -> ()  [unwired: 1 in, 2 out]
          }
          frame #1 {
            n893 = property on="log table" class="Tbl (strict)"() -> ("Position:Top"=w2632:i32, "Position:Left"=w2629:i32, "Bounds:Width"=w2628:u32)  [unwired: 2 in, 2 out]
            n894 = property on="sort" class="Bool"() -> ("Position:Left"=w2626:i32, "Bounds:Width"=w2625:u32)  [unwired: 2 in, 2 out]
            n895 = To Long Integer(number=w2628) -> (32bit integer=w2627:i32)
            n896 = To Long Integer(number=w2625) -> (32bit integer=w2624:i32)
            n897 = Add(x=w2629, y=w2627) -> (x+y=w2623:i32)
            n898 = Add(x=w2626, y=w2624) -> (x+y=w2622:i32)
            n899 = Subtract(x=w2632, y=24) -> (x-y=w2630:i32)
            n900 = Subtract(x=w2623, y=w2622) -> (x-y=w2621:i32)
            n901 = stacked-sequence {
              tunnel: w2630 -> [w2636 w2640 w2644 w2648 w2652 w2656 w2660 w2664 w2668]
              tunnel: w2621 -> [w2633 w2637 w2641 w2645 w2649 w2653 w2657 w2661 w2665]
              frame #0 {
                n902 = property on="add" class="Bool"() -> ("Position:Left"=w2635:i32)  [unwired: 2 in, 2 out]
                n903 = Add(x=w2635, y=w2633) -> (x+y=w2634:i32)
                n904 = property on="add" class="Bool"("Position:Top"=w2636, "Position:Left"=w2634) -> ()  [unwired: 2 in, 2 out]
              }
              frame #1 {
                n905 = property on="multi" class="Bool"() -> ("Position:Left"=w2639:i32)  [unwired: 2 in, 2 out]
                n906 = Add(x=w2639, y=w2637) -> (x+y=w2638:i32)
                n907 = property on="multi" class="Bool"("Position:Top"=w2640, "Position:Left"=w2638) -> ()  [unwired: 2 in, 2 out]
              }
              frame #2 {
                n908 = property on="subset" class="Bool"() -> ("Position:Left"=w2643:i32)  [unwired: 2 in, 2 out]
                n909 = Add(x=w2643, y=w2641) -> (x+y=w2642:i32)
                n910 = property on="subset" class="Bool"("Position:Top"=w2644, "Position:Left"=w2642) -> ()  [unwired: 2 in, 2 out]
              }
              frame #3 {
                n911 = property on="insert" class="Bool"() -> ("Position:Left"=w2647:i32)  [unwired: 2 in, 2 out]
                n912 = Add(x=w2647, y=w2645) -> (x+y=w2646:i32)
                n913 = property on="insert" class="Bool"("Position:Top"=w2648, "Position:Left"=w2646) -> ()  [unwired: 2 in, 2 out]
              }
              frame #4 {
                n914 = property on="mode" class="Bool"() -> ("Position:Left"=w2651:i32)  [unwired: 2 in, 2 out]
                n915 = Add(x=w2651, y=w2649) -> (x+y=w2650:i32)
                n916 = property on="mode" class="Bool"("Position:Top"=w2652, "Position:Left"=w2650) -> ()  [unwired: 2 in, 2 out]
              }
              frame #5 {
                n917 = property on="remove all" class="Bool"() -> ("Position:Left"=w2655:i32)  [unwired: 2 in, 2 out]
                n918 = Add(x=w2655, y=w2653) -> (x+y=w2654:i32)
                n919 = property on="remove all" class="Bool"("Position:Top"=w2656, "Position:Left"=w2654) -> ()  [unwired: 2 in, 2 out]
              }
              frame #6 {
                n920 = property on="reorder" class="Bool"() -> ("Position:Left"=w2659:i32)  [unwired: 2 in, 2 out]
                n921 = Add(x=w2659, y=w2657) -> (x+y=w2658:i32)
                n922 = property on="reorder" class="Bool"("Position:Top"=w2660, "Position:Left"=w2658) -> ()  [unwired: 2 in, 2 out]
              }
              frame #7 {
                n923 = property on="sort" class="Bool"() -> ("Position:Left"=w2663:i32)  [unwired: 2 in, 2 out]
                n924 = Add(x=w2663, y=w2661) -> (x+y=w2662:i32)
                n925 = property on="sort" class="Bool"("Position:Top"=w2664, "Position:Left"=w2662) -> ()  [unwired: 2 in, 2 out]
              }
              frame #8 {
                n926 = property on="remove" class="Bool"() -> ("Position:Left"=w2667:i32)  [unwired: 2 in, 2 out]
                n927 = Add(x=w2667, y=w2665) -> (x+y=w2666:i32)
                n928 = property on="remove" class="Bool"("Position:Top"=w2668, "Position:Left"=w2666) -> ()  [unwired: 2 in, 2 out]
              }
            }
          }
          frame #2 {
            n929 = property class="VI"() -> ("Front Panel"=w2670:refnum<vi>)  [unwired: 2 in, 2 out]
            n930 = property class="Pnl"(reference=w2670, "Defer Panel Updates"=FALSE) -> ()  [unwired: 1 in, 2 out]
          }
        }
      }
      frame "initialize" {
        n931 = while "rebuild init list on first run or after load or recompile" {
          shift-left: _ -> [w2683]
          shift-right: [w2682] -> w2680
          stop <- FALSE continue-if-true
          n932 = Array Size(array=w2683) -> (size(s)=w2684:i32)
          n933 = case shown="0" w2684 {
            tunnel: [w2685 w2705] -> w2682
            tunnel: w2683 -> [w2686 w2705]
            frame 0 {
              n934 = while {
                shift-left: w2686 -> [w2695]
                shift-right: [w2693] -> w2685
                shift-left: _ -> [w2697]
                shift-right: [w2692] -> _
                i -> [w2700]
                stop <- w2688 continue-if-true
                n935 = To Unsigned Word Integer(number=w2700) -> (unsigned 16bit integer=w2698:u16)
                n936 = Type Cast(type=t_DataLog_Log_Table_States."initialize" ("states"), x=w2698) -> (*(type *) &x=w2694:T6)
                n937 = Format Into String(format string="%s" ("Format String"), w2694) -> (resulting string=w2692:string)  [unwired: 2 in, 1 out]
                n938 = Not Equal?(x=w2692, y=w2697) -> (x != y?=w2688:bool)
                n939 = Match Pattern(string=w2692, regular expression="^init ") -> (offset past match=w2690:i32)  [unwired: 1 in, 3 out]
                n940 = Greater Or Equal To 0?(x=w2690) -> (x >= 0?=w2689:bool)
                n941 = And(x=w2689, y=w2688) -> (x .and. y?=w2687:bool)
                n942 = case shown="True" w2687 {
                  tunnel: w2695 -> [w2701 w2704]
                  tunnel: w2694 -> [_ w2703]
                  tunnel: [w2701 w2702] -> w2693
                  frame False {
                  }
                  frame True {
                    n943 = Build Array (concatenate)(w2704, w2703) -> (w2702:T6[])
                  }
                }
              }
            }
            frame Default {
            }
          }
        }
      }
      frame "init refs" {
        w2740 = T6[] [enum."cleanup"] items=["empty queue", "retrieve", "ret clear", "ret presize", "ret range", "ret merge", "ret at", "ret step", "ret times", "ret interpolate", "ret tabulate", "ret free", "num. exclude", "num. include", "str. exclude", "str. include", "time graph", "graph xy", "xy query", "xy check", "xy open", "xy set", "xy correlate", "xy run", "export", "show string", "count rows", "time headers", "tabulate", "abort query", "clear query", "clear all", "set database", "deselect", "ablement", "resize", "initialize", "init refs", "init databases", "init persist", "cleanup", "stop"] ("Array Constant")
        n944 = call "obj_ClientSrv Connection State.vi"("machine{connect}/VI{get state} name (local/no path resolution)"="DataLog Databases_srv.vi") -> ("server app ref"=w2714:refnum<vi>, "resolved server path"=w2715:path, "error out"=w2716:errorcluster)  [unwired: 7 in, 5 out]
        n945 = local read "databases"() -> (w2713:T5)
        n946 = local read "query"() -> (w2722:T3)
        n947 = stacked-sequence {
          tunnel: [w2768] -> w2712
          tunnel: [w2767] -> w2717
          tunnel: w2716 -> [w2766]
          tunnel: w2714 -> [w2765]
          tunnel: w2715 -> [w2764]
          tunnel: w2713 -> [w2763]
          frame #0 {
            # "avoid LV8 complaints"
            n948 = Path to Array of Strings(0:w2764) -> (2:w2769:string[])  [unwired: 1 out]
            n949 = Array Size(array=w2769) -> (size(s)=w2770:i32)
            n950 = case shown="1" w2770 {
              tunnel: w2764 -> [w2777 w2783]
              tunnel: w2765 -> [w2775 w2782]
              tunnel: [w2773 w2778] -> w2768
              tunnel: [w2771 w2781] -> w2767
              tunnel: w2763 -> [w2772 w2780]
              tunnel: w2766 -> [w2774 w2779]
              frame 1 {
                n951 = Path To String(path=w2777) -> (string=w2776:string)
                n952 = Open VI Reference(type specifier VI Refnum (for type only)=w2772, application reference (local)=w2775, vi path=w2776, error in (no error)=w2774) -> (vi reference=w2773:T5, error out=w2771:errorcluster)  [unwired: 2 in]
              }
              frame Default {
                n953 = Open VI Reference(type specifier VI Refnum (for type only)=w2780, application reference (local)=w2782, vi path=w2783, error in (no error)=w2779) -> (vi reference=w2778:T5, error out=w2781:errorcluster)  [unwired: 2 in]
              }
            }
          }
        }
        "databases" <- w2712
        n954 = call "Library Open VI Ref Error Clarifier.vi"("VI path"=w2715, "called VI error (no error)"=w2717) -> ("error out"=w2735:errorcluster)  [unwired: 13 in]
        n955 = call "obj_ClientSrv Connection State.vi"("machine{connect}/VI{get state} name (local/no path resolution)"="DataLog Database Infos_srv.vi", "error in (no error)"=w2735) -> ("server app ref"=w2708:refnum<vi>, "resolved server path"=w2707:path, "error out"=w2706:errorcluster)  [unwired: 6 in, 5 out]
        n956 = local read "database infos"() -> (w2710:T4)
        n957 = stacked-sequence {
          tunnel: [w2747] -> w2709
          tunnel: [w2746] -> w2711
          tunnel: w2706 -> [w2745]
          tunnel: w2708 -> [w2744]
          tunnel: w2707 -> [w2743]
          tunnel: w2710 -> [w2742]
          frame #0 {
            # "avoid LV8 complaints"
            n958 = Path to Array of Strings(0:w2743) -> (2:w2748:string[])  [unwired: 1 out]
            n959 = Array Size(array=w2748) -> (size(s)=w2749:i32)
            n960 = case shown="1" w2749 {
              tunnel: w2743 -> [w2756 w2762]
              tunnel: w2744 -> [w2754 w2761]
              tunnel: [w2752 w2757] -> w2747
              tunnel: [w2750 w2760] -> w2746
              tunnel: w2742 -> [w2751 w2759]
              tunnel: w2745 -> [w2753 w2758]
              frame 1 {
                n961 = Path To String(path=w2756) -> (string=w2755:string)
                n962 = Open VI Reference(type specifier VI Refnum (for type only)=w2751, application reference (local)=w2754, vi path=w2755, error in (no error)=w2753) -> (vi reference=w2752:T4, error out=w2750:errorcluster)  [unwired: 2 in]
              }
              frame Default {
                n963 = Open VI Reference(type specifier VI Refnum (for type only)=w2759, application reference (local)=w2761, vi path=w2762, error in (no error)=w2758) -> (vi reference=w2757:T4, error out=w2760:errorcluster)  [unwired: 2 in]
              }
            }
          }
        }
        "database infos" <- w2709
        n964 = call "Library Open VI Ref Error Clarifier.vi"("VI path"=w2707, "called VI error (no error)"=w2711) -> ("error out"=w2733:errorcluster)  [unwired: 13 in]
        n965 = call "obj_ClientSrv Connection State.vi"("machine{connect}/VI{get state} name (local/no path resolution)"="re_DataLog Query_srv.vi", "error in (no error)"=w2733) -> ("server app ref"=w2720:refnum<vi>, "resolved server path"=w2719:path, "error out"=w2718:errorcluster)  [unwired: 6 in, 5 out]
        n966 = stacked-sequence {
          tunnel: [w2789] -> w2721
          tunnel: [w2788] -> w2723
          tunnel: w2718 -> [w2787]
          tunnel: w2720 -> [w2786]
          tunnel: w2719 -> [w2785]
          tunnel: w2722 -> [w2784]
          frame #0 {
            # "avoid LV8 complaints"
            n967 = Path to Array of Strings(0:w2785) -> (2:w2790:string[])  [unwired: 1 out]
            n968 = Array Size(array=w2790) -> (size(s)=w2791:i32)
            n969 = case shown="1" w2791 {
              tunnel: w2785 -> [w2798 w2804]
              tunnel: w2786 -> [w2796 w2803]
              tunnel: [w2794 w2799] -> w2789
              tunnel: [w2792 w2802] -> w2788
              tunnel: w2784 -> [w2793 w2801]
              tunnel: w2787 -> [w2795 w2800]
              frame 1 {
                n970 = Path To String(path=w2798) -> (string=w2797:string)
                n971 = Open VI Reference(type specifier VI Refnum (for type only)=w2793, application reference (local)=w2796, vi path=w2797, error in (no error)=w2795) -> (vi reference=w2794:T3, error out=w2792:errorcluster)  [unwired: 2 in]
              }
              frame Default {
                n972 = Open VI Reference(type specifier VI Refnum (for type only)=w2801, application reference (local)=w2803, vi path=w2804, error in (no error)=w2800) -> (vi reference=w2799:T3, error out=w2802:errorcluster)  [unwired: 2 in]
              }
            }
          }
        }
        "query" <- w2721
        n973 = call "Library Open VI Ref Error Clarifier.vi"("VI path"=w2719, "called VI error (no error)"=w2723) -> ("error out"=w2732:errorcluster)  [unwired: 13 in]
        n974 = call "Library Log Error to Window.vi"("error in (no error)"=w2732) -> ()  [unwired: 13 in, 2 out]
        n975 = Select(t=w2740, s=w2732, f=w2739) -> (s? t:f=w2741:T6[])
      }
      frame "init databases" {
        w2822 = T6[] [enum."cleanup"] items=["empty queue", "retrieve", "ret clear", "ret presize", "ret range", "ret merge", "ret at", "ret step", "ret times", "ret interpolate", "ret tabulate", "ret free", "num. exclude", "num. include", "str. exclude", "str. include", "time graph", "graph xy", "xy query", "xy check", "xy open", "xy set", "xy correlate", "xy run", "export", "show string", "count rows", "time headers", "tabulate", "abort query", "clear query", "clear all", "set database", "deselect", "ablement", "resize", "initialize", "init refs", "init databases", "init persist", "cleanup", "stop"] ("Array Constant")
        n976 = call "obj_ClientSrv Client Access State.vi"() -> ("certificate"=w2817:string, "error out"=w2820:errorcluster)  [unwired: 14 in]
        n977 = local read "databases"() -> (w2819:T5)
        n978 = call-by-ref "?"(reference=w2819, error in=w2820, "certificate in"=w2817) -> (error out=w2821:errorcluster, "database names"=w2813:string[], 15:"error out"=w2818:errorcluster)  [unwired: 13 in, 1 out]
        n979 = call "Library Remote Call Error Merger.vi"("call by reference node error"=w2821, "called VI error (no error)"=w2818) -> ("error out"=w2816:errorcluster)  [unwired: 13 in]
        n980 = property on="database" class="Ring (strict)"(error in=w2816, "Value"=0 ("index"), "Strings []"=w2813) -> (error out=w2814:errorcluster)  [unwired: 1 in, 1 out]
        n981 = call "Library Log Error to Window.vi"("error in (no error)"=w2814) -> ("dup error"=w2824:errorcluster)  [unwired: 13 in, 1 out]
        n982 = Select(t=w2822, s=w2824, f=w2823) -> (s? t:f=w2825:T6[])
      }
      frame "init persist" {
        w2832 = T6[] [enum."resize", enum."set database"] items=["empty queue", "retrieve", "ret clear", "ret presize", "ret range", "ret merge", "ret at", "ret step", "ret times", "ret interpolate", "ret tabulate", "ret free", "num. exclude", "num. include", "str. exclude", "str. include", "time graph", "graph xy", "xy query", "xy check", "xy open", "xy set", "xy correlate", "xy run", "export", "show string", "count rows", "time headers", "tabulate", "abort query", "clear query", "clear all", "set database", "deselect", "ablement", "resize", "initialize", "init refs", "init databases", "init persist", "cleanup", "stop"] ("Array Constant")
        n983 = call "Libary Persist Position and Controls.vi"("action"=enum16{"save", "load"}."load") -> ()  [unwired: 13 in, 2 out]
        n984 = Build Array (concatenate)(w2832, w2837) -> (w2836:T6[])
      }
      frame "cleanup" {
        w2854 = T6[] [enum."clear all", enum."stop"] items=["empty queue", "retrieve", "ret clear", "ret presize", "ret range", "ret merge", "ret at", "ret step", "ret times", "ret interpolate", "ret tabulate", "ret free", "num. exclude", "num. include", "str. exclude", "str. include", "time graph", "graph xy", "xy query", "xy check", "xy open", "xy set", "xy correlate", "xy run", "export", "show string", "count rows", "time headers", "tabulate", "abort query", "clear query", "clear all", "set database", "deselect", "ablement", "resize", "initialize", "init refs", "init databases", "init persist", "cleanup", "stop"] ("Array Constant")
        n985 = local read "database infos"() -> (w2850:T4)
        n986 = local read "databases"() -> (w2851:T5)
        n987 = local read "query"() -> (w2849:T3)
        n988 = call "obj_Library Session.vi"("method"=t_Library_Session_Methods."delist") -> ()  [unwired: 11 in, 4 out]
        n989 = call "Libary Persist Position and Controls.vi"("action"=enum16{"save", "load"}."save") -> ()  [unwired: 13 in, 2 out]
        n990 = Close Reference(reference=w2851) -> ()  [unwired: 1 in, 1 out]
        n991 = Close Reference(reference=w2850) -> ()  [unwired: 1 in, 1 out]
        n992 = Close Reference(reference=w2849) -> ()  [unwired: 1 in, 1 out]
      }
      frame "stop" {
        n993 = invoke class="VI" method="FP.Close"() -> ()  [unwired: 3 in, 3 out]
      }
    }
  }
